vi "PLC_comm.vi"() -> ()   [LabVIEW 2017]
uses:
  <vilib>/addons/database/NI_Database_API.lvlib
  Global/DATA LOG.vi
  Global/Global 1.vi
  <vilib>/DATA AHEAD/SP7/typedefs/PLC Type.ctl
  <vilib>/DATA AHEAD/SP7/SP7.lvlib
  <vilib>/DATA AHEAD/SP7/functions/read/read String.vi
  <vilib>/DATA AHEAD/SP7/functions/write/write Dint array.vi
  <vilib>/DATA AHEAD/SP7/functions/read/read Dint array.vi
  <vilib>/Utility/error.llb/DialogType.ctl
  <vilib>/DATA AHEAD/SP7/functions/read/read real array.vi
  <vilib>/DATA AHEAD/SP7/functions/write/writeString.vi
  84f8396c-11e3-4f6e-927f-d6cb52f8486f.vi
  edb3f7e3-deb4-4efd-b63a-82a20ab466dd.vi
  737c4a97-5810-4f09-bfe1-7e6a970161fd.vi
  98a23aa7-5d76-4ce5-89a1-7ffa2d6e86d6.vi
  065602cd-1ec6-46a4-aff5-3b00a0c776c3.vi
  <vilib>/DATA AHEAD/SP7/typedefs/S7 Connection.ctl
  Control/PLC_Comm_State.ctl
  <vilib>/addons/database/Connection.llb/DB Tools Open Connec (String).vi
  f53d9a16-31ea-4c58-9ec6-4ab155e6634a.vi
  f2e501b8-8033-40fd-b99e-90a89dd29cf5.vi
  a17ecfbb-e8aa-4e6f-9723-a9b27e8c0652.vi
  3deaaee4-0312-4209-8b7c-ccc637c44985.vi
  adc7d8b8-ea76-443b-992e-07ffa118bf03.vi
  cf2a4f70-d875-4391-b4be-4b1ea527ec99.vi
  b767813d-b0bc-4642-82b7-59e8eeaf8486.vi
panel:
  out "error out 4":errorcluster
  out "error out 3":errorcluster
  out "IP1 8":string
  out "PLC 8":bool
  out "IP1 7":string
  out "PLC 7":bool
  out "IP1 6":string
  out "PLC 6":bool
  out "IP1 5":string
  out "PLC 5":bool
  out "PLC 4":bool
  out "PLC 3":bool
  out "PLC 1":bool
  out "IP1 4":string
  out "IP1 3":string
  out "IP1 2":string
  out "IP1":string
  in  "stop":bool
  out "error out":errorcluster
  in  "error in (no error)":errorcluster
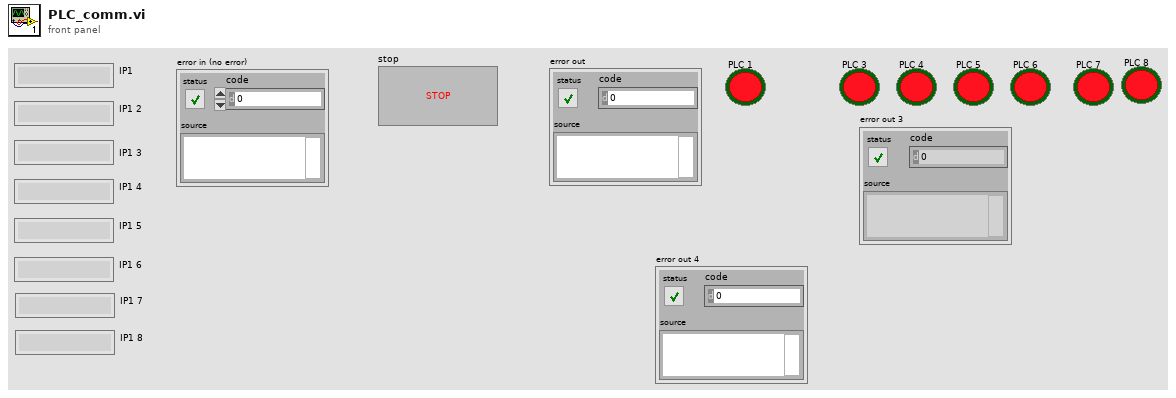
[diagram p1: front panel]
types:
  T1 = typedef "PLC_Comm_State.ctl" = enum16{"Int", "Connect", "Write", "Write2", "Write3", "Read", "Read2", "Read3", "Error", "Disconnect"}
  T2 = typedef "DialogType.ctl" = u16
  T3 = typedef "NI_Database_API.lvlib/Conn ObjectReference.ctl" = refnum<k1>
  T4 = typedef "SP7.lvlib/PLC Type.ctl" = enum16{"S7 200", "S7 300/400", "S7 1200", "S7 1500", "LOGO!8"}
  T5 = typedef "SP7.lvlib/S7 Connection.ctl" = cluster{"TCP Connection Ref":refnum<k5>, "IP address":string, "timeout ms":i32, "Connected?":bool, "PLC Type":T4, "Rack S7 400":u8, "Slot S7 400":u8, "PDU Size":u16, "connection semaphore":T6}
  T6 = typedef "Semaphore RefNum" = refnum<k1>
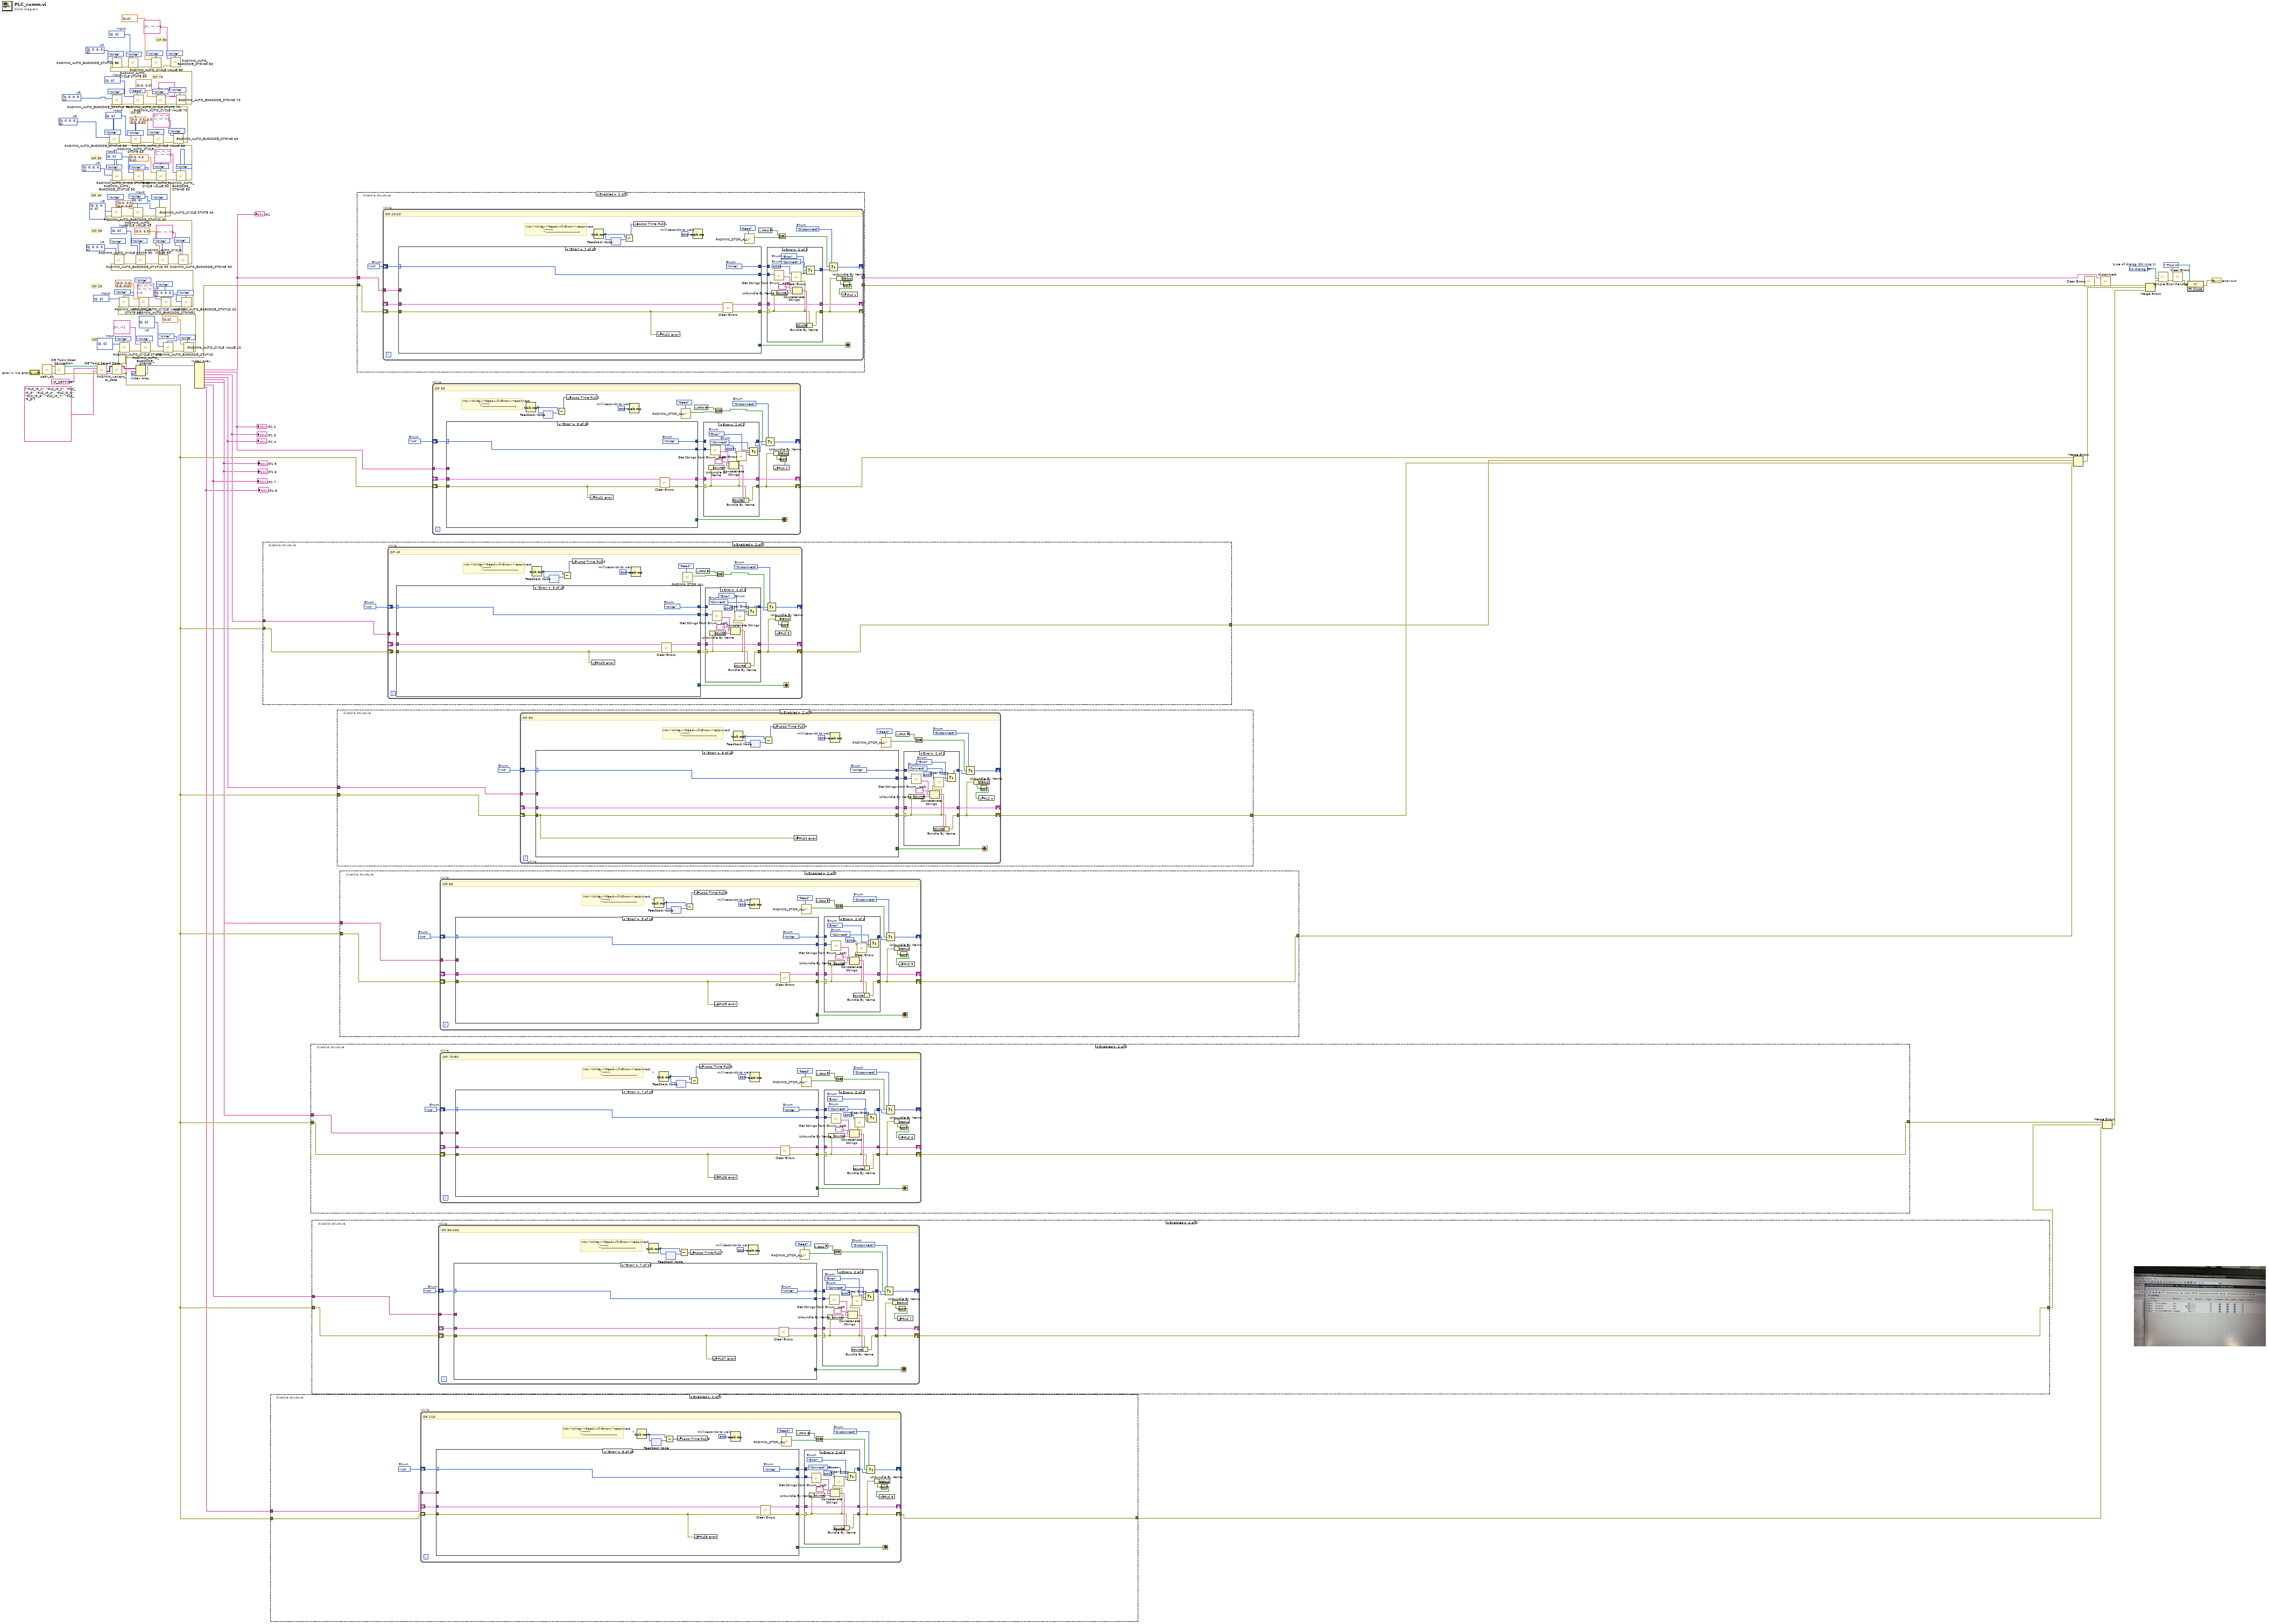
[diagram p0: block diagram]
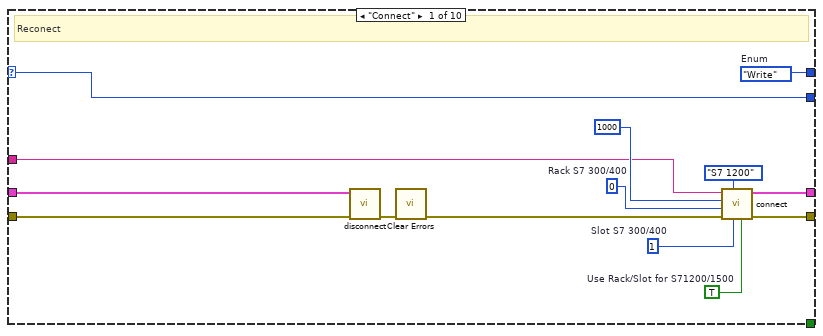
[diagram p3: hidden frame]
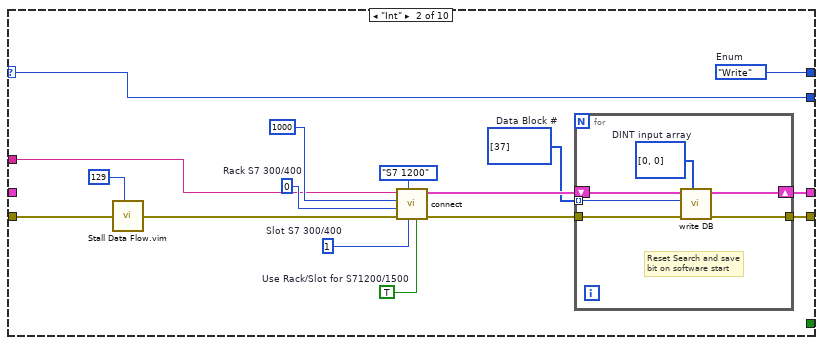
[diagram p4: hidden frame]
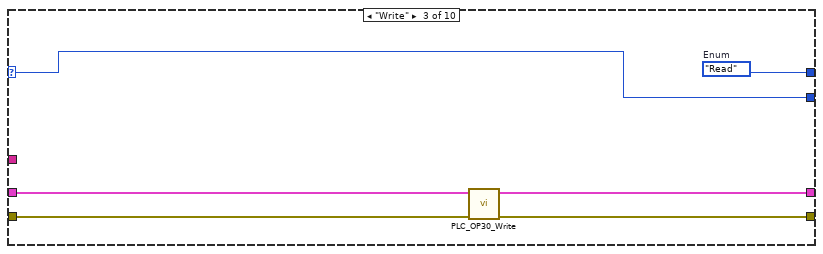
[diagram p5: hidden frame]
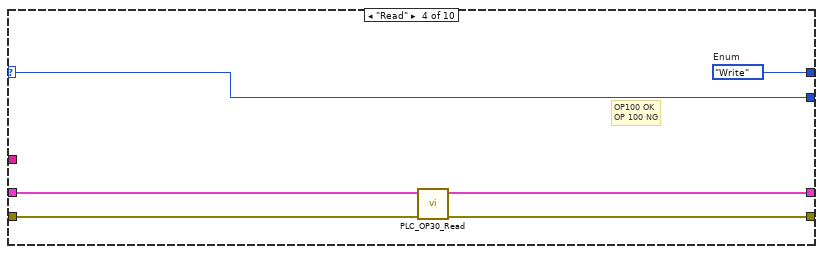
[diagram p6: hidden frame]
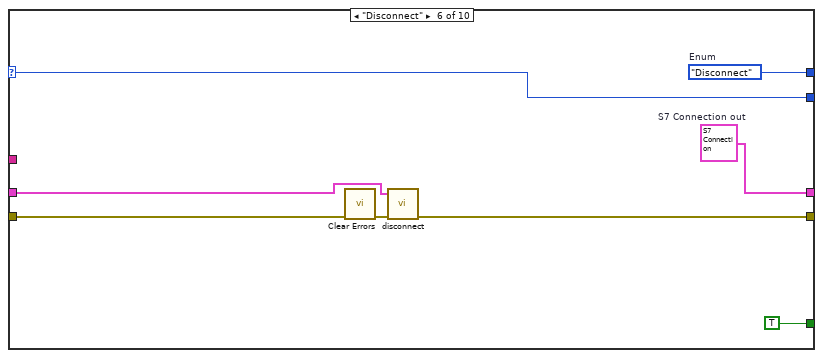
[diagram p7: hidden frame]
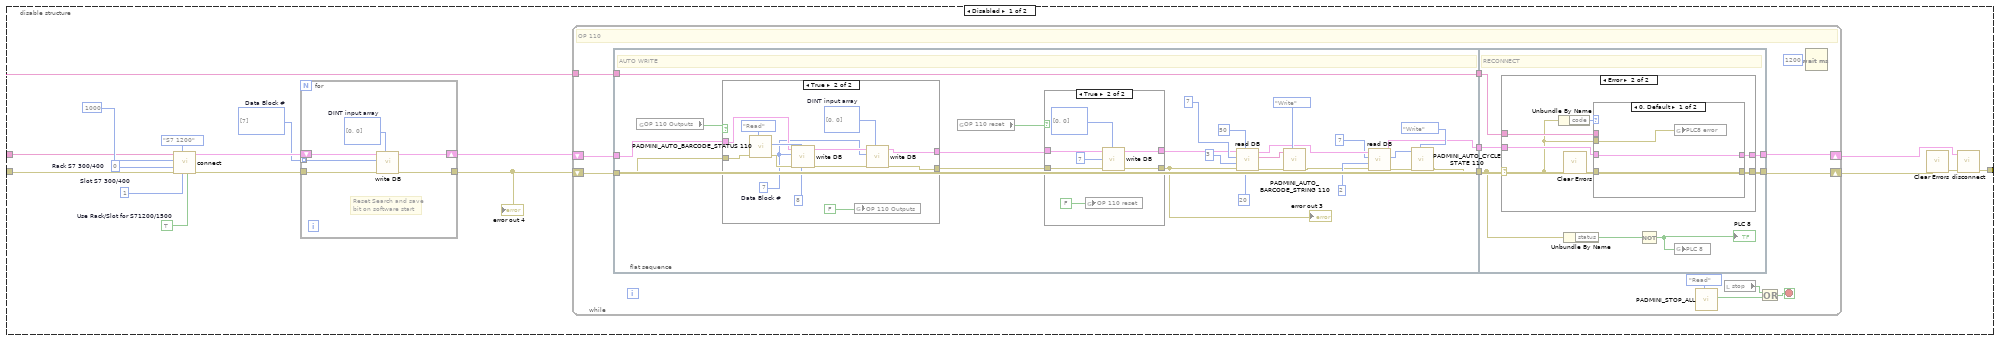
[diagram p12: hidden frame]
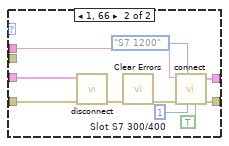
[diagram p16: hidden frame]
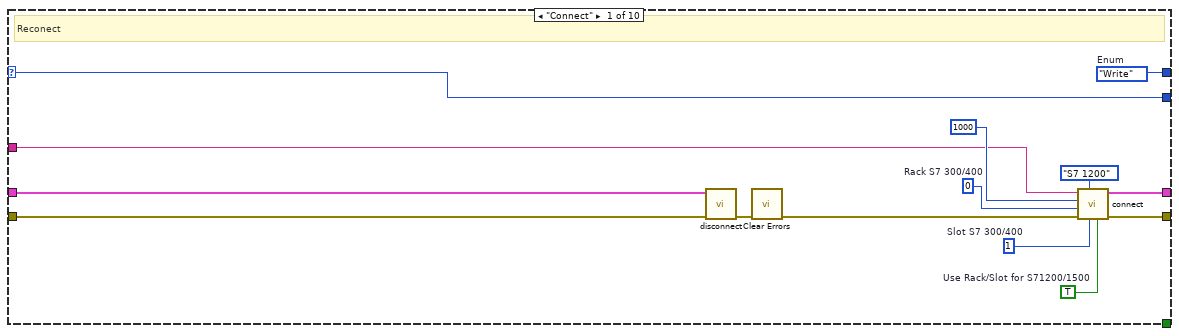
[diagram p18: hidden frame]
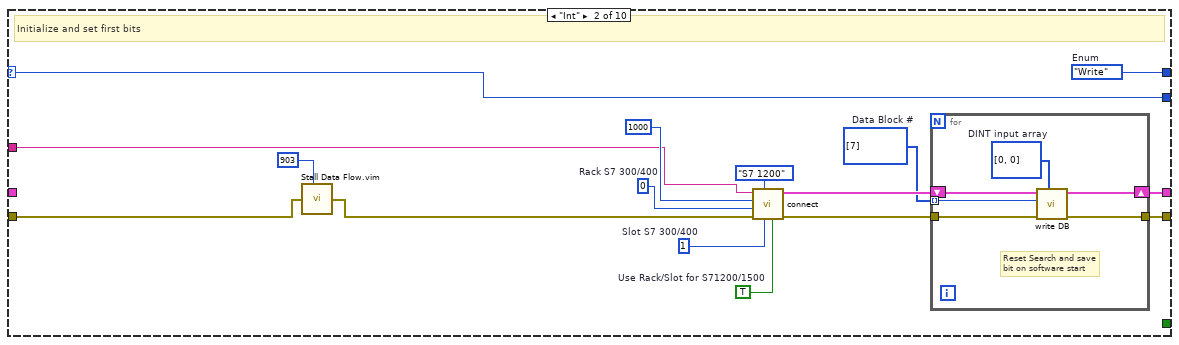
[diagram p19: hidden frame]
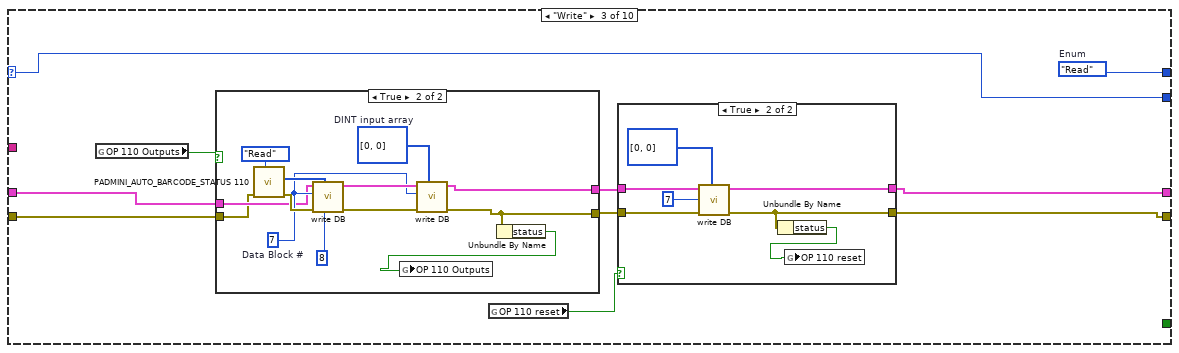
[diagram p20: hidden frame]
diagram:
  w1 = PLC_Comm_State."Int"  # Enum
  w10 = T2 0 items=["no dialog", "OK message", "continue or stop message", "OK message + warnings", "continue/stop + warnings"]  # type of dialog (OK msg:1)
  w12 = i32[] [0, 0, 0, 0, 0]  # I/P
  w13 = i32[] [0, 0]  # Input
  w15 = i32[] [0, 0]  # Input
  w16 = i32[] [0, 0]  # Input
  w18 = i32[] [0, 0]  # Input
  w14 = i32[] [0, 0, 0, 0, 0]  # I/P
  w17 = i32[] [0, 0, 0, 0, 0]  # I/P
  w19 = i32[] [0, 0, 0, 0, 0]  # I/P
  w20 = i32[] [0, 0, 0, 0, 0]  # I/P
  w21 = i32[] [0, 0]  # Input
  w22 = i32[] [0, 0]  # Input
  w23 = i32[] [0, 0, 0, 0, 0]  # I/P
  w24 = i32[] [0, 0, 0, 0, 0]  # I/P
  w25 = i32[] [0, 0]  # Input
  w26 = i32[] [0, 0]  # I/P
  w27 = i32[] [0, 0]  # Input
  # "OP 80"
  # "OP 70"
  # "OP 60"
  # "OP 50"
  # "OP 40"
  # "OP 30"
  # "OP 20"
  # "OP 10"
  n1 = call "path_db.vi"("error in"="error in (no error)") -> ("error out"=w128:errorcluster, "resulting string"=w133:string)  [unwired: 9 in]
  n2 = call-poly <vilib>:"DB Tools Open Connection.vi"("error in (no error)"=w128, "connection information"=w133) -> ("error out"=w132:errorcluster, "connection reference"=w131:T3)  [unwired: 6 in]
  n3 = call <vilib>:"DB Tools Select Data.vi"("error in (no error)"=w132, "columns"=string[] ["PLC_IP_1", "PLC_IP_2", "PLC_IP_3", "PLC_IP_4", "PLC_IP_5", "PLC_IP_6", "PLC_IP_7", "PLC_IP_8"], "table"="IP_SETTING", "connection reference"=w131) -> ("error out"=w130:errorcluster, "data"=w129:variant[][])  [unwired: 2 in, 1 out]
  n4 = call "PADMINI_varient_to_data.vi"("error in (no error)"=w130, "data"=w129) -> ("error out"=w9:errorcluster, "Array"=w124:string[][])  [unwired: 8 in]
  n5 = call "PADMINI_AUTO_CYCLE STATE.vi"("Enum"=enum16{"Read", "Write"}."Write", "error in (no error)"=w9, "Input"=w27) -> ("error out"=w114:errorcluster)  [unwired: 7 in, 1 out]
  n6 = Index Array(array=w124, index (row)=0) -> (element=w123:string[])  [unwired: 1 in]
  n7 = call "PADMINI_AUTO_BARCODE_STRING.vi"("Enum"=enum16{"Read", "Write"}."Write", "error in (no error)"=w114, "Input"=string[] ["", ""]) -> ("error out"=w111:errorcluster)  [unwired: 7 in, 1 out]
  n8 = call "PADMINI_AUTO_BARCODE_STATUS.vi"("Enum"=enum16{"Read", "Write"}."Write", "error in (no error)"=w111, "I/P"=w26) -> ("error out"=w109:errorcluster)  [unwired: 7 in, 1 out]
  n9 = call "PADMINI_AUTO_CYCLE VALUE 10.vi"("Enum"=enum16{"Read", "Write"}."Write", "error in (no error)"=w109, "Input"=dbl[] [0.0]) -> ("error out"=w103:errorcluster)  [unwired: 7 in, 1 out]
  n10 = call "PADMINI_AUTO_CYCLE STATE 20.vi"("Enum"=enum16{"Read", "Write"}."Write", "error in (no error)"=w103, "Input"=w13) -> ("error out"=w101:errorcluster)  [unwired: 7 in, 1 out]
  n11 = call "PADMINI_AUTO_CYCLE VALUE 20.vi"("Enum"=enum16{"Read", "Write"}."Write", "error in (no error)"=w101, "Input"=dbl[] [0.0, 0.0, 0.0, 0.0]) -> ("error out"=w97:errorcluster)  [unwired: 7 in, 1 out]
  n12 = call "PADMINI_AUTO_BARCODE_STRING2.vi"("Enum"=enum16{"Read", "Write"}."Write", "error in (no error)"=w97, "Input"=string[] ["", "", "", "", "", "", ""]) -> ("error out"=w95:errorcluster)  [unwired: 7 in, 1 out]
  n13 = call "PADMINI_AUTO_BARCODE_STATUS 20.vi"("Enum"=enum16{"Read", "Write"}."Write", "error in (no error)"=w95, "I/P"=w12) -> ("error out"=w93:errorcluster)  [unwired: 7 in, 1 out]
  n14 = call "PADMINI_AUTO_BARCODE_STATUS 30.vi"("Enum"=enum16{"Read", "Write"}."Write", "error in (no error)"=w93, "I/P"=w14) -> ("error out"=w90:errorcluster)  [unwired: 7 in, 1 out]
  n15 = call "PADMINI_AUTO_CYCLE STATE 30.vi"("Enum"=enum16{"Read", "Write"}."Write", "error in (no error)"=w90, "Input"=w15) -> ("error out"=w89:errorcluster)  [unwired: 7 in, 1 out]
  n16 = call "PADMINI_AUTO_CYCLE VALUE 30.vi"("Enum"=enum16{"Read", "Write"}."Write", "error in (no error)"=w89, "Input"=dbl[] [0.0, 0.0]) -> ("error out"=w86:errorcluster)  [unwired: 7 in, 1 out]
  n17 = call "PADMINI_AUTO_BARCODE_STRING 30.vi"("Enum"=enum16{"Read", "Write"}."Write", "error in (no error)"=w86, "Input"=string[] ["", "", ""]) -> ("error out"=w76:errorcluster)  [unwired: 7 in, 1 out]
  n18 = call "PADMINI_AUTO_BARCODE_STATUS 40.vi"("Enum"=enum16{"Read", "Write"}."Write", "error in (no error)"=w76, "I/P"=w17) -> ("error out"=w75:errorcluster)  [unwired: 7 in, 1 out]
  n19 = call "PADMINI_AUTO_CYCLE VALUE 40.vi"("Enum"=enum16{"Read", "Write"}."Write", "error in (no error)"=w75, "Input"=dbl[] [0.0, 0.0, 0.0, 0.0]) -> ("error out"=w74:errorcluster)  [unwired: 7 in, 1 out]
  n20 = call "PADMINI_AUTO_CYCLE STATE 40.vi"("Enum"=enum16{"Read", "Write"}."Write", "error in (no error)"=w74, "Input"=w16) -> ("error out"=w73:errorcluster)  [unwired: 7 in, 1 out]
  n21 = call "PADMINI_AUTO_BARCODE_STATUS 50.vi"("Enum"=enum16{"Read", "Write"}."Write", "error in (no error)"=w73, "I/P"=w19) -> ("error out"=w65:errorcluster)  [unwired: 7 in, 1 out]
  n22 = call "PADMINI_AUTO_CYCLE STATE 50.vi"("Enum"=enum16{"Read", "Write"}."Write", "error in (no error)"=w65, "Input"=w18) -> ("error out"=w69:errorcluster)  [unwired: 7 in, 1 out]
  n23 = call "PADMINI_AUTO_CYCLE VALUE 50.vi"("Enum"=enum16{"Read", "Write"}."Write", "error in (no error)"=w69, "Input"=dbl[] [0.0, 0.0, 0.0]) -> ("error out"=w66:errorcluster)  [unwired: 7 in, 1 out]
  n24 = call "PADMINI_AUTO_BARCODE_STRING 50.vi"("Enum"=enum16{"Read", "Write"}."Write", "error in (no error)"=w66, "Input"=string[] ["", "", "", "", "", ""]) -> ("error out"=w51:errorcluster)  [unwired: 7 in, 1 out]
  n25 = call "PADMINI_AUTO_BARCODE_STATUS 60.vi"("Enum"=enum16{"Read", "Write"}."Write", "error in (no error)"=w51, "I/P"=w20) -> ("error out"=w55:errorcluster)  [unwired: 7 in, 1 out]
  n26 = call "PADMINI_AUTO_CYCLE STATE 60.vi"("Enum"=enum16{"Read", "Write"}."Write", "error in (no error)"=w55, "Input"=w21) -> ("error out"=w57:errorcluster)  [unwired: 7 in, 1 out]
  n27 = call "PADMINI_AUTO_CYCLE VALUE 60.vi"("Enum"=enum16{"Read", "Write"}."Write", "error in (no error)"=w57, "Input"=dbl[] [0.0, 0.0, 0.0, 0.0, 0.0]) -> ("error out"=w60:errorcluster)  [unwired: 7 in, 1 out]
  n28 = call "PADMINI_AUTO_BARCODE_STRING 60.vi"("Enum"=enum16{"Read", "Write"}."Write", "error in (no error)"=w60, "Input"=string[] ["", "", "", "", "", ""]) -> ("error out"=w34:errorcluster)  [unwired: 7 in, 1 out]
  n29 = call "PADMINI_AUTO_BARCODE_STATUS 70.vi"("Enum"=enum16{"Read", "Write"}."Write", "error in (no error)"=w34, "I/P"=w23) -> ("error out"=w37:errorcluster)  [unwired: 7 in, 1 out]
  n30 = call "PADMINI_AUTO_CYCLE STATE 70.vi"("Enum"=enum16{"Read", "Write"}."Read", "error in (no error)"=w37, "Input"=w22) -> ("error out"=w49:errorcluster)  [unwired: 7 in, 1 out]
  n31 = call "PADMINI_AUTO_CYCLE VALUE 70.vi"("Enum"=enum16{"Read", "Write"}."Write", "error in (no error)"=w49, "Input"=dbl[] [0.0, 0.0]) -> ("error out"=w46:errorcluster)  [unwired: 7 in, 1 out]
  n32 = call "PADMINI_AUTO_BARCODE_STRING 70.vi"("Enum"=enum16{"Read", "Write"}."Write", "error in (no error)"=w46, "Input"=string[] ["", ""]) -> ("error out"=w31:errorcluster)  [unwired: 7 in, 1 out]
  n33 = call "PADMINI_AUTO_BARCODE_STATUS 80.vi"("Enum"=enum16{"Read", "Write"}."Write", "error in (no error)"=w31, "I/P"=w24) -> ("error out"=w38:errorcluster)  [unwired: 7 in, 1 out]
  n34 = call "PADMINI_AUTO_CYCLE STATE 80.vi"("Enum"=enum16{"Read", "Write"}."Write", "error in (no error)"=w38, "Input"=w25) -> ("error out"=w42:errorcluster)  [unwired: 7 in, 1 out]
  n35 = call "PADMINI_AUTO_CYCLE VALUE 80.vi"("Enum"=enum16{"Read", "Write"}."Write", "error in (no error)"=w42, "Input"=sgl[] [0.0]) -> ("error out"=w45:errorcluster)  [unwired: 7 in, 1 out]
  n36 = call "PADMINI_AUTO_BARCODE_STRING 80.vi"("Enum"=enum16{"Read", "Write"}."Write", "error in (no error)"=w45, "Input"=string[] ["", "", ""]) -> ()  [unwired: 7 in, 2 out]
  n37 = Index Array(array=w123) -> (element #1=w82:string, element #2=w83:string, element #3=w81:string, element #4=w71:string, element #5=w61:string, element #6=w30:string, element #7=w29:string, element #8=w8:string)  [unwired: 8 in]
  "IP1" <- w82
  "IP1 2" <- w83
  "IP1 3" <- w81
  "IP1 4" <- w71
  "IP1 5" <- w61
  "IP1 6" <- w30
  "IP1 7" <- w29
  "IP1 8" <- w8
  n38 = disable-structure shown="Enabled" {
    disable-tunnel: w81 -> [w148 w270]
    disable-tunnel: w9 -> [w139 w269]
    disable-tunnel: [w134 w268] -> w3
    frame Disabled {
      w136 = TRUE  # Use Rack/Slot for S71200/1500
      w137 = u8 0  # Rack S7 300/400
      w138 = u8 1  # Slot S7 300/400
      w144 = i32[] [0, 0]  # DINT input array
      # "Reset Search and save \nbit on software start"
      n39 = call <vilib>:"connect.vi"("Use Rack/Slot for S71200/1500"=w136, "Slot S7 300/400"=w138, "PLC Type"=PLC_Type."S7 1200" ("PLC Type 2"), "error in (no error)"=w139, "Rack S7 300/400"=w137, "timeout [ms]"=1000 ("timeout [ms] 2"), "IP address"=w148) -> ("error out"=w141:errorcluster, "S7 Connection out"=w140:T5)  [unwired: 3 in]
      n40 = call-poly <vilib>:"write DB.vi"("DINT input array"=w144, "error in (no error)"=w141, "Data Block #"=u16 56, "S7 Connection in"=w140) -> ("error out"=w143:errorcluster, "S7 Connection out"=w142:T5)  [unwired: 4 in, 2 out]
      n41 = while {
        shift-right: [w153] -> w146
        shift-left: w142 -> [w163]
        shift-right: [w161] -> w147
        shift-left: w143 -> [w162]
        tunnel: w148 -> [w152]
        stop <- w155 stop-if-true
        # "OP 40"
        n42 = flat-sequence {
          tunnel: [w165] -> w159
          tunnel: [w168] -> w154
          tunnel: w162 -> [w213]
          tunnel: w163 -> [w212]
          tunnel: w152 -> [w200]
          tunnel: [w200] -> w151
          tunnel: [w241] -> w161
          tunnel: [w240] -> w153
          tunnel: w159 -> [w243]
          tunnel: w154 -> [w242]
          tunnel: w151 -> [w239]
          frame #0 {
            w193 = u16 57 ("Data Block #")
            w164 = u16 56 ("Data Block #")
            # "AUTO WRITE"
            n43 = global read "DATA LOG.vi" "OP 40 Outputs"() -> (w211:bool)
            n44 = case shown="True" w211 {
              tunnel: w212 -> [w224 w237]
              tunnel: [w225 w229] -> w198
              tunnel: [w224 w231] -> w199
              tunnel: w213 -> [w225 w234]
              frame False {
              }
              frame True {
                w238 = u16 57  # Data Block #
                n45 = call "PADMINI_AUTO_BARCODE_STATUS 40.vi"("Enum"=enum16{"Read", "Write"}."Read", "error in (no error)"=w234) -> ("error out"=w233:errorcluster, "O/P"=w235:i32[])  [unwired: 8 in]
                n46 = global write "DATA LOG.vi" "OP 40 Outputs"(FALSE) -> ()
                n47 = call-poly <vilib>:"write DB.vi"("DINT input array"=w235, "error in (no error)"=w233, "Data Block #"=w238, "S7 Connection in"=w237) -> ("error out"=w228:errorcluster, "S7 Connection out"=w230:T5)  [unwired: 4 in, 2 out]
                n48 = call-poly <vilib>:"write DB.vi"("DINT input array"=i32[] [0], "error in (no error)"=w228, "Data Block #"=u16 56, "S7 Connection in"=w230) -> ("error out"=w229:errorcluster, "S7 Connection out"=w231:T5)  [unwired: 4 in, 2 out]
              }
            }
            n49 = global read "DATA LOG.vi" "OP 40 reset"() -> (w197:bool)
            n50 = global read "DATA LOG.vi" "Auto Cycle On"() -> (w175:bool)
            n51 = case shown="True" w197 {
              tunnel: w198 -> [w214 w223]
              tunnel: [w214 w222] -> w186
              tunnel: w199 -> [w215 w221]
              tunnel: [w215 w220] -> w187
              frame False {
              }
              frame True {
                n52 = global write "DATA LOG.vi" "OP 40 reset"(FALSE) -> ()
                n53 = call-poly <vilib>:"write DB.vi"("Item offset [byte]"=u16 4 ("Data Block #"), "DINT input array"=i32[] [0], "error in (no error)"=w223, "Data Block #"=u16 56, "S7 Connection in"=w221) -> ("error out"=w222:errorcluster, "S7 Connection out"=w220:T5)  [unwired: 3 in, 2 out]
              }
            }
            n54 = Boolean To (0,1)(Boolean=w175) -> (0, 1=w174:i16)
            n55 = Build Array(w174) -> (w173:i16[])
            n56 = global read "Global 1.vi" "Filtered BARCODE selected"() -> (w196:string[])
            n57 = call-poly <vilib>:"write DB.vi"("Item offset [byte]"=u32 20, "DINT input array"=w173, "error in (no error)"=w186, "Data Block #"=w193, "S7 Connection in"=w187) -> ("error out"=w191:errorcluster, "S7 Connection out"=w190:T5)  [unwired: 3 in, 2 out]
            n58 = call-poly <vilib>:"write DB.vi"("Item offset [byte]"=u32 24, "Input STRINGS"=w196, "error in (no error)"=w191, "String length reserved in DB (default=254)"=u16 15, "Data Block #"=w193, "S7 Connection in"=w190) -> ("error out"=w188:errorcluster, "S7 Connection out"=w189:T5)  [unwired: 2 in, 2 out]
            n59 = call-poly <vilib>:"read DB.vi"("Item offset [byte]"=u32 8, "error in (no error)"=w188, "items #"=u16 4 ("Items # [byte]"), "Data Block #"=w164, "S7 Connection in"=w189) -> ("error out"=w203:errorcluster, "REAL result array"=w201:sgl[], "S7 Connection out"=w209:T5)  [unwired: 4 in]
            n60 = call "PADMINI_AUTO_CYCLE VALUE 40.vi"("Enum"=enum16{"Read", "Write"}."Write", "error in (no error)"=w203, "Input"=w201) -> ("error out"=w202:errorcluster)  [unwired: 7 in, 1 out]
            n61 = call-poly <vilib>:"read DB.vi"("Item offset [byte]"=u32 24, "String length reserved in DB (default=254)"=u16 50, "error in (no error)"=w202, "items #"=u16 1 ("Items # [byte]"), "Data Block #"=w164, "S7 Connection in"=w209) -> ("error out"=w185:errorcluster, "STRING result Array"=w178:string[], "S7 Connection out"=w183:T5)  [unwired: 2 in, 1 out]
            n62 = call-poly <vilib>:"read DB.vi"("Item offset [byte]"=u32 76, "String length reserved in DB (default=254)"=u16 10, "error in (no error)"=w185, "items #"=u16 4 ("Items # [byte]"), "Data Block #"=w164, "S7 Connection in"=w183) -> ("error out"=w184:errorcluster, "STRING result Array"=w177:string[], "S7 Connection out"=w166:T5)  [unwired: 2 in, 1 out]
            n63 = Build Array (concatenate)(w178, w177) -> (w176:string[])
            n64 = call "PADMINI_AUTO_BARCODE_STRING 40.vi"("Enum"=enum16{"Read", "Write"}."Write", "error in (no error)"=w184, "Input"=w176) -> ("error out"=w167:errorcluster)  [unwired: 7 in, 1 out]
            n65 = call-poly <vilib>:"read DB.vi"("error in (no error)"=w167, "items #"=u16 2 ("Items # [byte]"), "Data Block #"=w164, "S7 Connection in"=w166) -> ("error out"=w172:errorcluster, "DINT result array"=w171:i32[], "S7 Connection out"=w165:T5)  [unwired: 5 in]
            n66 = call "PADMINI_AUTO_CYCLE STATE 40.vi"("Enum"=enum16{"Read", "Write"}."Write", "error in (no error)"=w172, "Input"=w171) -> ("error out"=w168:errorcluster)  [unwired: 7 in, 1 out]
          }
          frame #1 {
            # "RECONNECT"
            n67 = case shown="Error" w242 {
              selector: w242 -> [w247 w248]
              tunnel: [w246 w252] -> w240
              tunnel: [w247 w253] -> w241
              tunnel: w243 -> [w246 w251]
              tunnel: w239 -> [_ w250]
              frame No Error {
              }
              frame Error {
                n68 = Unbundle By Name(w248) -> ("code"=w249:i32)
                n69 = call <vilib>:"Clear Errors.vi"("error in (no error)"=w248) -> ("error out"=w254:errorcluster)  [unwired: 5 in, 1 out]
                n70 = case shown="0, Default" w249 {
                  tunnel: w254 -> [w256 w267]
                  tunnel: [w256 w265] -> w253
                  tunnel: [w257 w264] -> w252
                  tunnel: w251 -> [w257 w261]
                  tunnel: w250 -> [_ w260]
                  tunnel: w248 -> [w255 _]
                  frame 0, Default {
                    n71 = global write "Global 1.vi" "PLC3 error"(w255) -> ()
                  }
                  frame 1 {
                    n72 = call <vilib>:"disconnect.vi"("error in (no error)"=w267, "S7 Connection in"=w261) -> ("error out"=w266:errorcluster)  [unwired: 8 in, 1 out]
                    n73 = call <vilib>:"Clear Errors.vi"("error in (no error)"=w266) -> ("error out"=w263:errorcluster)  [unwired: 5 in, 1 out]
                    n74 = call <vilib>:"connect.vi"("Use Rack/Slot for S71200/1500"=TRUE, "Slot S7 300/400"=u8 1, "PLC Type"=PLC_Type."S7 1200" ("PLC Type 2"), "error in (no error)"=w263, "IP address"=w260) -> ("error out"=w265:errorcluster, "S7 Connection out"=w264:T5)  [unwired: 5 in]
                  }
                }
              }
            }
            n75 = Unbundle By Name(w242) -> ("status"=w245:bool)
            n76 = Not(x=w245) -> (.not. x?=w244:bool)
            "PLC 3" <- w244
            n77 = global write "Global 1.vi" "PLC 3"(w244) -> ()
          }
        }
        n78 = call "PADMINI_STOP_ALL.vi"("Enum"=enum16{"Read", "Write"}."Read") -> ("Boolean 2"=w157:bool)  [unwired: 9 in, 1 out]
        n79 = local read "stop"() -> (w156:bool)
        n80 = Or(x=w156, y=w157) -> (x .or. y?=w155:bool)
        n81 = Wait (ms)(milliseconds to wait=u32 1200) -> ()  [unwired: 1 out]
      }
      n82 = call <vilib>:"Clear Errors.vi"("error in (no error)"=w147) -> ("error out"=w135:errorcluster)  [unwired: 5 in, 1 out]
      n83 = call <vilib>:"disconnect.vi"("error in (no error)"=w135, "S7 Connection in"=w146) -> ("error out"=w134:errorcluster)  [unwired: 8 in, 1 out]
    }
    frame Enabled {
      w271 = PLC_Comm_State."Int"  # Enum
      n84 = while {
        shift-right: [w285] -> _
        shift-left: w271 -> [w294]
        shift-right: [w275] -> w268
        shift-left: w269 -> [w293]
        shift-right: [w288] -> _
        shift-left: _ -> [w292]
        tunnel: w270 -> [w291]
        stop <- w286 stop-if-true
        w282 = PLC_Comm_State."Disconnect"  # Enum
        w290 = u32 800  # milliseconds to wait
        # "Int-->Write-->Read---if--Error-->reconnect\n               ^------v                                       v\n                ^------------------------------v"
        # "OP 40"
        n85 = case shown="\"Error\"" w294 {
          selector: w294 -> [w313 w331 w369 w422 w434 w438 _ _ _ _]
          tunnel: [w318 w333 w350 w397 w435 w443 w445 w448 w450 w452] -> w295
          tunnel: [w319 w329 w348 w395 w436 w440 w446 w447 w449 w451] -> w287
          tunnel: w293 -> [w316 w327 w351 w398 w432 w441 w445 w448 w450 w452]
          tunnel: w292 -> [w314 _ w349 w396 w436 w442 w446 w447 w449 w451]
          tunnel: w291 -> [w320 w332 _ _ _ _ _ _ _ _]
          tunnel: [w312 w330 w368 w421 w433 w437 _ _ _ _] -> w289
          tunnel: [_ _ _ _ _ TRUE _ _ _ _] -> w286
          tunnel: [w313 w331 w369 w422 w434 w438 _ _ _ _] -> w283
          frame "Connect" {
            w312 = PLC_Comm_State."Write"  # Enum
            w325 = TRUE  # Use Rack/Slot for S71200/1500
            w324 = u8 1  # Slot S7 300/400
            w322 = u8 0  # Rack S7 300/400
            # "Reconect"
            n86 = call <vilib>:"disconnect.vi"("error in (no error)"=w316, "S7 Connection in"=w314) -> ("error out"=w317:errorcluster)  [unwired: 8 in, 1 out]
            n87 = call <vilib>:"Clear Errors.vi"("error in (no error)"=w317) -> ("error out"=w315:errorcluster)  [unwired: 5 in, 1 out]
            n88 = call <vilib>:"connect.vi"("Use Rack/Slot for S71200/1500"=w325, "Slot S7 300/400"=w324, "PLC Type"=PLC_Type."S7 1200" ("PLC Type 2"), "error in (no error)"=w315, "Rack S7 300/400"=w322, "timeout [ms]"=1000 ("timeout [ms] 2"), "IP address"=w320) -> ("error out"=w318:errorcluster, "S7 Connection out"=w319:T5)  [unwired: 3 in]
          }
          frame "Int" {
            w330 = PLC_Comm_State."Write"  # Enum
            w334 = TRUE  # Use Rack/Slot for S71200/1500
            w335 = u8 1  # Slot S7 300/400
            w336 = u8 0  # Rack S7 300/400
            w337 = u16[] [56]  # Data Block #
            n89 = call "Stall Data Flow.vim"("value in"=w327, "milliseconds to wait"=u32 258) -> ("value out"=w326:errorcluster)  [unwired: 1 out]
            n90 = call <vilib>:"connect.vi"("Use Rack/Slot for S71200/1500"=w334, "Slot S7 300/400"=w335, "PLC Type"=PLC_Type."S7 1200" ("PLC Type 2"), "error in (no error)"=w326, "Rack S7 300/400"=w336, "timeout [ms]"=1000 ("timeout [ms] 2"), "IP address"=w332) -> ("error out"=w339:errorcluster, "S7 Connection out"=w338:T5)  [unwired: 3 in]
            n91 = for {
              tunnel: w337 -> [w347] mode=indexing
              shift-right: [w345] -> w329
              shift-left: w338 -> [w343]
              tunnel: w339 -> [w344]
              tunnel: [w342] -> w333
              w346 = i32[] [0, 0]  # DINT input array
              # "Reset Search and save \nbit on software start"
              n92 = call-poly <vilib>:"write DB.vi"("DINT input array"=w346, "error in (no error)"=w344, "Data Block #"=w347, "S7 Connection in"=w343) -> ("error out"=w342:errorcluster, "S7 Connection out"=w345:T5)  [unwired: 4 in, 2 out]
            }
          }
          frame "Write" {
            w353 = u16 57 ("Data Block #")
            w368 = PLC_Comm_State."Read"  # Enum
            n93 = global read "DATA LOG.vi" "OP 40 Outputs"() -> (w367:bool)
            n94 = case shown="True" w367 {
              tunnel: w349 -> [w380 w382]
              tunnel: [w381 w384] -> w365
              tunnel: [w380 w389] -> w366
              tunnel: w351 -> [w381 w391]
              frame False {
              }
              frame True {
                w394 = u16 57  # Data Block #
                n95 = call "PADMINI_AUTO_BARCODE_STATUS 40.vi"("Enum"=enum16{"Read", "Write"}."Read", "error in (no error)"=w391) -> ("error out"=w390:errorcluster, "O/P"=w392:i32[])  [unwired: 8 in]
                n96 = call-poly <vilib>:"write DB.vi"("DINT input array"=w392, "error in (no error)"=w390, "Data Block #"=w394, "S7 Connection in"=w382) -> ("error out"=w387:errorcluster, "S7 Connection out"=w388:T5)  [unwired: 4 in, 2 out]
                n97 = call-poly <vilib>:"write DB.vi"("DINT input array"=i32[] [0], "error in (no error)"=w387, "Data Block #"=u16 56, "S7 Connection in"=w388) -> ("error out"=w384:errorcluster, "S7 Connection out"=w389:T5)  [unwired: 4 in, 2 out]
                n98 = Unbundle By Name(w384) -> ("status"=w383:bool)
                n99 = global write "DATA LOG.vi" "OP 40 Outputs"(w383) -> ()
              }
            }
            n100 = global read "DATA LOG.vi" "OP 40 reset"() -> (w364:bool)
            n101 = case shown="True" w364 {
              tunnel: w365 -> [w370 w379]
              tunnel: [w370 w374] -> w359
              tunnel: w366 -> [w371 w378]
              tunnel: [w371 w372] -> w360
              frame False {
              }
              frame True {
                n102 = call-poly <vilib>:"write DB.vi"("Item offset [byte]"=u16 4 ("Data Block #"), "DINT input array"=i32[] [0], "error in (no error)"=w379, "Data Block #"=u16 56, "S7 Connection in"=w378) -> ("error out"=w374:errorcluster, "S7 Connection out"=w372:T5)  [unwired: 3 in, 2 out]
                n103 = Unbundle By Name(w374) -> ("status"=w373:bool)
                n104 = global write "DATA LOG.vi" "OP 40 reset"(w373) -> ()
              }
            }
            n105 = global read "DATA LOG.vi" "Auto Cycle On"() -> (w358:bool)
            n106 = global read "Global 1.vi" "Filtered BARCODE selected"() -> (w363:string[])
            n107 = Boolean To (0,1)(Boolean=w358) -> (0, 1=w357:i16)
            n108 = Build Array(w357) -> (w356:i16[])
            n109 = call-poly <vilib>:"write DB.vi"("Item offset [byte]"=u32 20, "DINT input array"=w356, "error in (no error)"=w359, "Data Block #"=w353, "S7 Connection in"=w360) -> ("error out"=w362:errorcluster, "S7 Connection out"=w361:T5)  [unwired: 3 in, 2 out]
            n110 = call-poly <vilib>:"write DB.vi"("Item offset [byte]"=u32 24, "Input STRINGS"=w363, "error in (no error)"=w362, "String length reserved in DB (default=254)"=u16 15, "Data Block #"=w353, "S7 Connection in"=w361) -> ("error out"=w350:errorcluster, "S7 Connection out"=w348:T5)  [unwired: 2 in, 2 out]
          }
          frame "Read" {
            w407 = u16 56 ("Data Block #")
            w421 = PLC_Comm_State."Write"  # Enum
            n111 = call-poly <vilib>:"read DB.vi"("Item offset [byte]"=u32 8, "error in (no error)"=w398, "items #"=u16 4 ("Items # [byte]"), "Data Block #"=w407, "S7 Connection in"=w396) -> ("error out"=w417:errorcluster, "REAL result array"=w420:sgl[], "S7 Connection out"=w418:T5)  [unwired: 4 in]
            n112 = call-poly <vilib>:"read DB.vi"("Item offset [byte]"=u32 24, "String length reserved in DB (default=254)"=u16 50, "error in (no error)"=w417, "items #"=u16 1 ("Items # [byte]"), "Data Block #"=w407, "S7 Connection in"=w418) -> ("error out"=w416:errorcluster, "STRING result Array"=w413:string[], "S7 Connection out"=w414:T5)  [unwired: 2 in, 1 out]
            n113 = call-poly <vilib>:"read DB.vi"("Item offset [byte]"=u32 76, "String length reserved in DB (default=254)"=u16 10, "error in (no error)"=w416, "items #"=u16 4 ("Items # [byte]"), "Data Block #"=w407, "S7 Connection in"=w414) -> ("error out"=w415:errorcluster, "STRING result Array"=w412:string[], "S7 Connection out"=w409:T5)  [unwired: 2 in, 1 out]
            n114 = Build Array (concatenate)(w413, w412) -> (w419:string[])
            n115 = call-poly <vilib>:"read DB.vi"("error in (no error)"=w415, "items #"=u16 2 ("Items # [byte]"), "Data Block #"=w407, "S7 Connection in"=w409) -> ("error out"=w411:errorcluster, "DINT result array"=w410:i32[], "S7 Connection out"=w395:T5)  [unwired: 5 in]
            n116 = case shown="No Error" w411 {
              selector: w411 -> [w426 w431]
              tunnel: w410 -> [w430 _]
              tunnel: w419 -> [w428 _]
              tunnel: w420 -> [w424 _]
              tunnel: [w423 w431] -> w397
              frame No Error {
                w425 = enum16{"Read", "Write"}."Write" ("Enum")
                n117 = call "PADMINI_AUTO_CYCLE VALUE 40.vi"("Enum"=w425, "error in (no error)"=w426, "Input"=w424) -> ("error out"=w427:errorcluster)  [unwired: 7 in, 1 out]
                n118 = call "PADMINI_AUTO_BARCODE_STRING 40.vi"("Enum"=w425, "error in (no error)"=w427, "Input"=w428) -> ("error out"=w429:errorcluster)  [unwired: 7 in, 1 out]
                n119 = call "PADMINI_AUTO_CYCLE STATE 40.vi"("Enum"=w425, "error in (no error)"=w429, "Input"=w430) -> ("error out"=w423:errorcluster)  [unwired: 7 in, 1 out]
              }
              frame Error {
              }
            }
          }
          frame "Error" {
            w433 = PLC_Comm_State."Write"  # Enum
            n120 = global write "Global 1.vi" "PLC3 error"(w432) -> ()
            n121 = call <vilib>:"Clear Errors.vi"("error in (no error)"=w432) -> ("error out"=w435:errorcluster)  [unwired: 5 in, 1 out]
          }
          frame "Disconnect" {
            w437 = PLC_Comm_State."Disconnect"  # Enum
            w440 = T5 {"TCP Connection Ref"=refnum, "IP address"="", "timeout ms"=5000, "Connected?"=FALSE, "PLC Type"=enum."S7 1200", "Rack S7 400"=0, "Slot S7 400"=0, "PDU Size"=0, "connection semaphore"=refnum}  # S7 Connection out
            n122 = call <vilib>:"Clear Errors.vi"("error in (no error)"=w441) -> ("error out"=w444:errorcluster)  [unwired: 5 in, 1 out]
            n123 = call <vilib>:"disconnect.vi"("error in (no error)"=w444, "S7 Connection in"=w442) -> ("error out"=w443:errorcluster)  [unwired: 8 in, 1 out]
          }
          frame "Write2" {
            # "No Use"
          }
          frame "Write3" {
            # "No Use"
          }
          frame "Read2" {
            # "No Use"
          }
          frame "Read3" {
            # "No Use"
          }
        }
        n124 = Tick Count (ms)() -> (millisecond timer value=w274:u32)
        n125 = feedback #1() -> (w273:u32)  [unwired: 1 in]
        n126 = feedback-in #1(w274) -> ()
        n127 = Subtract(x=w274, y=w273) -> (x-y=w272:u32)
        n128 = global write "Global 1.vi" "Loop Time PLC 3"(w272) -> ()
        n129 = Wait (ms)(milliseconds to wait=w290) -> ()  [unwired: 1 out]
        n130 = call "PADMINI_STOP_ALL.vi"("Enum"=enum16{"Read", "Write"}."Read") -> ("Boolean 2"=w281:bool)  [unwired: 9 in, 1 out]
        n131 = local read "stop"() -> (w280:bool)
        n132 = case shown="Error" w295 {
          selector: w295 -> [w298 w301]
          tunnel: [w298 w305] -> w275
          tunnel: [w297 w300] -> w284
          tunnel: w289 -> [w297 _]
          tunnel: [w296 w311] -> w288
          tunnel: w287 -> [w296 w311]
          tunnel: w283 -> [_ w309]
          frame No Error {
          }
          frame Error {
            w302 = PLC_Comm_State."Connect"  # Enum
            w299 = PLC_Comm_State."Error"  # Enum
            n133 = Unbundle By Name(w301) -> ("source"=w310:string)
            n134 = call <userlib>:"Get Strings from Enum__ogtk.vi"("Enum"=w309) -> ("String Value"=w308:string)  [unwired: 7 in, 3 out]
            n135 = Concatenate Strings(w308, "    " ("string"), w310) -> (w306:string)
            n136 = Bundle By Name(cluster=w301, "source"=w306) -> (w305:errorcluster)
            n137 = call <vilib>:"Clear Errors.vi"("error in (no error)"=w301, "specific error code to clear (0: all)"=6002) -> ("specific error cleared?"=w304:bool)  [unwired: 4 in, 1 out]
            n138 = Select(t=w302, s=w304, f=w299) -> (s? t:f=w300:T1)
          }
        }
        n139 = Or(x=w280, y=w281) -> (x .or. y?=w278:bool)
        n140 = Select(t=w282, s=w278, f=w284) -> (s? t:f=w285:T1)
        n141 = Unbundle By Name(w275) -> ("status"=w277:bool)
        n142 = Not(x=w277) -> (.not. x?=w276:bool)
        n143 = global write "Global 1.vi" "PLC 3"(w276) -> ()
      }
    }
  }
  n144 = disable-structure shown="Enabled" {
    disable-tunnel: w9 -> [w462 w567]
    disable-tunnel: w8 -> [w460 w568]
    disable-tunnel: [w456 w566] -> w7
    frame Disabled {
      w453 = TRUE  # Use Rack/Slot for S71200/1500
      w454 = u8 1  # Slot S7 300/400
      w455 = u8 0  # Rack S7 300/400
      w461 = u16[] [7]  # Data Block #
      n145 = call <vilib>:"connect.vi"("Use Rack/Slot for S71200/1500"=w453, "Slot S7 300/400"=w454, "PLC Type"=PLC_Type."S7 1200" ("PLC Type 2"), "error in (no error)"=w462, "Rack S7 300/400"=w455, "timeout [ms]"=1000 ("timeout [ms] 2"), "IP address"=w460) -> ("error out"=w464:errorcluster, "S7 Connection out"=w463:T5)  [unwired: 3 in]
      n146 = for {
        tunnel: w461 -> [w474] mode=indexing
        shift-right: [w472] -> w467
        shift-left: w463 -> [w469]
        tunnel: w464 -> [w470]
        tunnel: [w471] -> w468
        w473 = i32[] [0, 0]  # DINT input array
        # "Reset Search and save \nbit on software start"
        n147 = call-poly <vilib>:"write DB.vi"("DINT input array"=w473, "error in (no error)"=w470, "Data Block #"=w474, "S7 Connection in"=w469) -> ("error out"=w471:errorcluster, "S7 Connection out"=w472:T5)  [unwired: 4 in, 2 out]
      }
      "error out 4" <- w468
      n148 = while {
        shift-right: [w477] -> w457
        shift-left: w467 -> [w487]
        shift-right: [w485] -> w458
        shift-left: w468 -> [w486]
        tunnel: w460 -> [w476]
        stop <- w479 stop-if-true
        # "OP 110"
        n149 = flat-sequence {
          tunnel: [w491] -> w483
          tunnel: [w492] -> w478
          tunnel: w486 -> [w510]
          tunnel: w487 -> [w511]
          tunnel: w476 -> [w512]
          tunnel: [w512] -> w475
          tunnel: [w539] -> w485
          tunnel: [w538] -> w477
          tunnel: w483 -> [w541]
          tunnel: w478 -> [w540]
          tunnel: w475 -> [w537]
          frame #0 {
            # "AUTO WRITE"
            n150 = global read "DATA LOG.vi" "OP 110 Outputs"() -> (w509:bool)
            n151 = case shown="True" w509 {
              tunnel: [w522 w527] -> w501
              tunnel: [w523 w528] -> w500
              tunnel: w510 -> [w522 w532]
              tunnel: w511 -> [w523 w531]
              frame False {
              }
              frame True {
                w524 = i32[] [0, 0]  # DINT input array
                w525 = u16 7  # Data Block #
                n152 = call "PADMINI_AUTO_BARCODE_STATUS 110.vi"("Enum"=enum16{"Read", "Write"}."Read", "error in (no error)"=w532) -> ("error out"=w534:errorcluster, "O/P"=w535:i32[])  [unwired: 8 in]
                n153 = call-poly <vilib>:"write DB.vi"("Item offset [byte]"=u32 8, "DINT input array"=w535, "error in (no error)"=w534, "Data Block #"=w525, "S7 Connection in"=w531) -> ("error out"=w526:errorcluster, "S7 Connection out"=w529:T5)  [unwired: 3 in, 2 out]
                n154 = global write "DATA LOG.vi" "OP 110 Outputs"(FALSE) -> ()
                n155 = call-poly <vilib>:"write DB.vi"("DINT input array"=w524, "error in (no error)"=w526, "Data Block #"=w525, "S7 Connection in"=w529) -> ("error out"=w527:errorcluster, "S7 Connection out"=w528:T5)  [unwired: 4 in, 2 out]
              }
            }
            n156 = global read "DATA LOG.vi" "OP 110 reset"() -> (w498:bool)
            n157 = case shown="True" w498 {
              tunnel: w501 -> [w513 w521]
              tunnel: [w513 w520] -> w502
              tunnel: w500 -> [w514 w519]
              tunnel: [w514 w518] -> w499
              frame False {
              }
              frame True {
                n158 = global write "DATA LOG.vi" "OP 110 reset"(FALSE) -> ()
                n159 = call-poly <vilib>:"write DB.vi"("DINT input array"=i32[] [0, 0], "error in (no error)"=w521, "Data Block #"=u16 7, "S7 Connection in"=w519) -> ("error out"=w520:errorcluster, "S7 Connection out"=w518:T5)  [unwired: 4 in, 2 out]
              }
            }
            "error out 3" <- w502
            n160 = call-poly <vilib>:"read DB.vi"("Item offset [byte]"=u32 20, "String length reserved in DB (default=254)"=u16 50, "error in (no error)"=w502, "items #"=u16 3 ("Items # [byte]"), "Data Block #"=u16 7, "S7 Connection in"=w499) -> ("error out"=w504:errorcluster, "STRING result Array"=w505:string[], "S7 Connection out"=w490:T5)  [unwired: 2 in, 1 out]
            n161 = call "PADMINI_AUTO_BARCODE_STRING 110.vi"("Enum"=enum16{"Read", "Write"}."Write", "error in (no error)"=w504, "Input"=w505) -> ("error out"=w493:errorcluster)  [unwired: 7 in, 1 out]
            n162 = call-poly <vilib>:"read DB.vi"("error in (no error)"=w493, "items #"=u16 2 ("Items # [byte]"), "Data Block #"=u16 7, "S7 Connection in"=w490) -> ("error out"=w497:errorcluster, "DINT result array"=w496:i32[], "S7 Connection out"=w491:T5)  [unwired: 5 in]
            n163 = call "PADMINI_AUTO_CYCLE STATE 110.vi"("Enum"=enum16{"Read", "Write"}."Write", "error in (no error)"=w497, "Input"=w496) -> ("error out"=w492:errorcluster)  [unwired: 7 in, 1 out]
          }
          frame #1 {
            # "RECONNECT"
            n164 = case shown="Error" w540 {
              selector: w540 -> [w545 w546]
              tunnel: [w544 w550] -> w538
              tunnel: [w545 w551] -> w539
              tunnel: w541 -> [w544 w549]
              tunnel: w537 -> [_ w548]
              frame No Error {
              }
              frame Error {
                n165 = Unbundle By Name(w546) -> ("code"=w547:i32)
                n166 = call <vilib>:"Clear Errors.vi"("error in (no error)"=w546) -> ("error out"=w552:errorcluster)  [unwired: 5 in, 1 out]
                n167 = case shown="0, Default" w547 {
                  tunnel: w552 -> [w554 w565]
                  tunnel: [w554 w563] -> w551
                  tunnel: [w555 w562] -> w550
                  tunnel: w549 -> [w555 w559]
                  tunnel: w548 -> [_ w558]
                  tunnel: w546 -> [w553 _]
                  frame 0, Default {
                    n168 = global write "Global 1.vi" "PLC8 error"(w553) -> ()
                  }
                  frame 1, 66 {
                    w557 = u8 1  # Slot S7 300/400
                    n169 = call <vilib>:"disconnect.vi"("error in (no error)"=w565, "S7 Connection in"=w559) -> ("error out"=w564:errorcluster)  [unwired: 8 in, 1 out]
                    n170 = call <vilib>:"Clear Errors.vi"("error in (no error)"=w564) -> ("error out"=w561:errorcluster)  [unwired: 5 in, 1 out]
                    n171 = call <vilib>:"connect.vi"("Use Rack/Slot for S71200/1500"=TRUE, "Slot S7 300/400"=w557, "PLC Type"=PLC_Type."S7 1200" ("PLC Type 2"), "error in (no error)"=w561, "IP address"=w558) -> ("error out"=w563:errorcluster, "S7 Connection out"=w562:T5)  [unwired: 5 in]
                  }
                }
              }
            }
            n172 = Unbundle By Name(w540) -> ("status"=w543:bool)
            n173 = Not(x=w543) -> (.not. x?=w542:bool)
            "PLC 8" <- w542
            n174 = global write "Global 1.vi" "PLC 8"(w542) -> ()
          }
        }
        n175 = call "PADMINI_STOP_ALL.vi"("Enum"=enum16{"Read", "Write"}."Read") -> ("Boolean 2"=w481:bool)  [unwired: 9 in, 1 out]
        n176 = local read "stop"() -> (w480:bool)
        n177 = Or(x=w480, y=w481) -> (x .or. y?=w479:bool)
        n178 = Wait (ms)(milliseconds to wait=u32 1200) -> ()  [unwired: 1 out]
      }
      n179 = call <vilib>:"Clear Errors.vi"("error in (no error)"=w458) -> ("error out"=w459:errorcluster)  [unwired: 5 in, 1 out]
      n180 = call <vilib>:"disconnect.vi"("error in (no error)"=w459, "S7 Connection in"=w457) -> ("error out"=w456:errorcluster)  [unwired: 8 in, 1 out]
    }
    frame Enabled {
      w569 = PLC_Comm_State."Int"  # Enum
      n181 = while {
        shift-right: [w584] -> _
        shift-left: w569 -> [w592]
        shift-right: [w576] -> w566
        shift-left: w567 -> [w591]
        shift-right: [w587] -> _
        shift-left: _ -> [w590]
        tunnel: w568 -> [w573]
        stop <- w585 stop-if-true
        w581 = PLC_Comm_State."Disconnect"  # Enum
        w589 = u32 800  # milliseconds to wait
        # "Int-->Write-->Read---if--Error-->reconnect\n               ^------v                                       v\n                ^------------------------------v"
        # "OP 110"
        n182 = case shown="\"Error\"" w592 {
          selector: w592 -> [w612 w629 w655 w696 w706 w710 _ _ _ _]
          tunnel: [w617 w631 w648 w682 w707 w715 w717 w720 w722 w724] -> w593
          tunnel: [w618 w630 w649 w683 w708 w712 w718 w719 w721 w723] -> w586
          tunnel: w591 -> [w615 w625 w646 w680 w704 w713 w717 w720 w722 w724]
          tunnel: w590 -> [w613 _ w647 w681 w708 w714 w718 w719 w721 w723]
          tunnel: [w611 w628 w654 w695 w705 w709 _ _ _ _] -> w588
          tunnel: [_ _ _ _ _ TRUE _ _ _ _] -> w585
          tunnel: [w612 w629 w655 w696 w706 w710 _ _ _ _] -> w582
          tunnel: w573 -> [w610 w627 _ _ _ _ _ _ _ _]
          frame "Connect" {
            w611 = PLC_Comm_State."Write"  # Enum
            w623 = TRUE  # Use Rack/Slot for S71200/1500
            w622 = u8 1  # Slot S7 300/400
            w620 = u8 0  # Rack S7 300/400
            # "Reconect"
            n183 = call <vilib>:"disconnect.vi"("error in (no error)"=w615, "S7 Connection in"=w613) -> ("error out"=w616:errorcluster)  [unwired: 8 in, 1 out]
            n184 = call <vilib>:"Clear Errors.vi"("error in (no error)"=w616) -> ("error out"=w614:errorcluster)  [unwired: 5 in, 1 out]
            n185 = call <vilib>:"connect.vi"("Use Rack/Slot for S71200/1500"=w623, "Slot S7 300/400"=w622, "PLC Type"=PLC_Type."S7 1200" ("PLC Type 2"), "error in (no error)"=w614, "Rack S7 300/400"=w620, "timeout [ms]"=1000 ("timeout [ms] 2"), "IP address"=w610) -> ("error out"=w617:errorcluster, "S7 Connection out"=w618:T5)  [unwired: 3 in]
          }
          frame "Int" {
            w628 = PLC_Comm_State."Write"  # Enum
            w632 = TRUE  # Use Rack/Slot for S71200/1500
            w633 = u8 1  # Slot S7 300/400
            w634 = u8 0  # Rack S7 300/400
            w635 = u16[] [7]  # Data Block #
            # "Initialize and set first bits"
            n186 = call "Stall Data Flow.vim"("value in"=w625, "milliseconds to wait"=u32 903) -> ("value out"=w624:errorcluster)  [unwired: 1 out]
            n187 = call <vilib>:"connect.vi"("Use Rack/Slot for S71200/1500"=w632, "Slot S7 300/400"=w633, "PLC Type"=PLC_Type."S7 1200" ("PLC Type 2"), "error in (no error)"=w624, "Rack S7 300/400"=w634, "timeout [ms]"=1000 ("timeout [ms] 2"), "IP address"=w627) -> ("error out"=w637:errorcluster, "S7 Connection out"=w636:T5)  [unwired: 3 in]
            n188 = for {
              tunnel: w635 -> [w645] mode=indexing
              shift-right: [w643] -> w630
              shift-left: w636 -> [w641]
              tunnel: w637 -> [w642]
              tunnel: [w640] -> w631
              w644 = i32[] [0, 0]  # DINT input array
              # "Reset Search and save \nbit on software start"
              n189 = call-poly <vilib>:"write DB.vi"("DINT input array"=w644, "error in (no error)"=w642, "Data Block #"=w645, "S7 Connection in"=w641) -> ("error out"=w640:errorcluster, "S7 Connection out"=w643:T5)  [unwired: 4 in, 2 out]
            }
          }
          frame "Write" {
            w654 = PLC_Comm_State."Read"  # Enum
            n190 = global read "DATA LOG.vi" "OP 110 Outputs"() -> (w653:bool)
            n191 = case shown="True" w653 {
              tunnel: [w665 w670] -> w652
              tunnel: [w666 w674] -> w651
              tunnel: w647 -> [w666 w668]
              tunnel: w646 -> [w665 w667]
              frame False {
              }
              frame True {
                w671 = i32[] [0, 0]  # DINT input array
                w672 = u16 7  # Data Block #
                n192 = call "PADMINI_AUTO_BARCODE_STATUS 110.vi"("Enum"=enum16{"Read", "Write"}."Read", "error in (no error)"=w667) -> ("error out"=w677:errorcluster, "O/P"=w678:i32[])  [unwired: 8 in]
                n193 = call-poly <vilib>:"write DB.vi"("Item offset [byte]"=u32 8, "DINT input array"=w678, "error in (no error)"=w677, "Data Block #"=w672, "S7 Connection in"=w668) -> ("error out"=w673:errorcluster, "S7 Connection out"=w675:T5)  [unwired: 3 in, 2 out]
                n194 = call-poly <vilib>:"write DB.vi"("DINT input array"=w671, "error in (no error)"=w673, "Data Block #"=w672, "S7 Connection in"=w675) -> ("error out"=w670:errorcluster, "S7 Connection out"=w674:T5)  [unwired: 4 in, 2 out]
                n195 = Unbundle By Name(w670) -> ("status"=w669:bool)
                n196 = global write "DATA LOG.vi" "OP 110 Outputs"(w669) -> ()
              }
            }
            n197 = global read "DATA LOG.vi" "OP 110 reset"() -> (w650:bool)
            n198 = case shown="True" w650 {
              tunnel: w652 -> [w656 w664]
              tunnel: [w656 w659] -> w648
              tunnel: w651 -> [w657 w663]
              tunnel: [w657 w662] -> w649
              frame False {
              }
              frame True {
                n199 = call-poly <vilib>:"write DB.vi"("DINT input array"=i32[] [0, 0], "error in (no error)"=w664, "Data Block #"=u16 7, "S7 Connection in"=w663) -> ("error out"=w659:errorcluster, "S7 Connection out"=w662:T5)  [unwired: 4 in, 2 out]
                n200 = Unbundle By Name(w659) -> ("status"=w658:bool)
                n201 = global write "DATA LOG.vi" "OP 110 reset"(w658) -> ()
              }
            }
          }
          frame "Read" {
            w695 = PLC_Comm_State."Write"  # Enum
            n202 = call-poly <vilib>:"read DB.vi"("Item offset [byte]"=u32 20, "String length reserved in DB (default=254)"=u16 50, "error in (no error)"=w680, "items #"=u16 3 ("Items # [byte]"), "Data Block #"=u16 7, "S7 Connection in"=w681) -> ("error out"=w693:errorcluster, "STRING result Array"=w694:string[], "S7 Connection out"=w690:T5)  [unwired: 2 in, 1 out]
            n203 = call-poly <vilib>:"read DB.vi"("error in (no error)"=w693, "items #"=u16 2 ("Items # [byte]"), "Data Block #"=u16 7, "S7 Connection in"=w690) -> ("error out"=w692:errorcluster, "DINT result array"=w691:i32[], "S7 Connection out"=w683:T5)  [unwired: 5 in]
            n204 = case shown="Error" w692 {
              selector: w692 -> [w701 w703]
              tunnel: w691 -> [w702 _]
              tunnel: w694 -> [w698 _]
              tunnel: [w697 w703] -> w682
              frame No Error {
                w699 = enum16{"Read", "Write"}."Write" ("Enum")
                n205 = call "PADMINI_AUTO_BARCODE_STRING 110.vi"("Enum"=w699, "error in (no error)"=w701, "Input"=w698) -> ("error out"=w700:errorcluster)  [unwired: 7 in, 1 out]
                n206 = call "PADMINI_AUTO_CYCLE STATE 110.vi"("Enum"=w699, "error in (no error)"=w700, "Input"=w702) -> ("error out"=w697:errorcluster)  [unwired: 7 in, 1 out]
              }
              frame Error {
              }
            }
          }
          frame "Error" {
            w705 = PLC_Comm_State."Write"  # Enum
            n207 = global write "Global 1.vi" "PLC8 error"(w704) -> ()
            n208 = call <vilib>:"Clear Errors.vi"("error in (no error)"=w704) -> ("error out"=w707:errorcluster)  [unwired: 5 in, 1 out]
          }
          frame "Disconnect" {
            w709 = PLC_Comm_State."Disconnect"  # Enum
            w712 = T5 {"TCP Connection Ref"=refnum, "IP address"="", "timeout ms"=5000, "Connected?"=FALSE, "PLC Type"=enum."S7 1200", "Rack S7 400"=0, "Slot S7 400"=0, "PDU Size"=0, "connection semaphore"=refnum}  # S7 Connection out
            n209 = call <vilib>:"Clear Errors.vi"("error in (no error)"=w713) -> ("error out"=w716:errorcluster)  [unwired: 5 in, 1 out]
            n210 = call <vilib>:"disconnect.vi"("error in (no error)"=w716, "S7 Connection in"=w714) -> ("error out"=w715:errorcluster)  [unwired: 8 in, 1 out]
          }
          frame "Write2" {
            # "No Use"
          }
          frame "Write3" {
            # "No Use"
          }
          frame "Read2" {
            # "No Use"
          }
          frame "Read3" {
            # "No Use"
          }
        }
        n211 = Tick Count (ms)() -> (millisecond timer value=w572:u32)
        n212 = feedback #2() -> (w571:u32)  [unwired: 1 in]
        n213 = feedback-in #2(w572) -> ()
        n214 = Subtract(x=w572, y=w571) -> (x-y=w570:u32)
        n215 = global write "Global 1.vi" "Loop Time PLC 8"(w570) -> ()
        n216 = Wait (ms)(milliseconds to wait=w589) -> ()  [unwired: 1 out]
        n217 = call "PADMINI_STOP_ALL.vi"("Enum"=enum16{"Read", "Write"}."Read") -> ("Boolean 2"=w580:bool)  [unwired: 9 in, 1 out]
        n218 = local read "stop"() -> (w575:bool)
        n219 = case shown="Error" w593 {
          selector: w593 -> [w596 w597]
          tunnel: [w596 w603] -> w576
          tunnel: [w595 w599] -> w583
          tunnel: w588 -> [w595 _]
          tunnel: [w594 w609] -> w587
          tunnel: w586 -> [w594 w609]
          tunnel: w582 -> [_ w607]
          frame No Error {
          }
          frame Error {
            w600 = PLC_Comm_State."Connect"  # Enum
            w598 = PLC_Comm_State."Error"  # Enum
            n220 = Unbundle By Name(w597) -> ("source"=w608:string)
            n221 = call <userlib>:"Get Strings from Enum__ogtk.vi"("Enum"=w607) -> ("String Value"=w606:string)  [unwired: 7 in, 3 out]
            n222 = Concatenate Strings(w606, "    " ("string"), w608) -> (w604:string)
            n223 = Bundle By Name(cluster=w597, "source"=w604) -> (w603:errorcluster)
            n224 = call <vilib>:"Clear Errors.vi"("error in (no error)"=w597, "specific error code to clear (0: all)"=6002) -> ("specific error cleared?"=w602:bool)  [unwired: 4 in, 1 out]
            n225 = Select(t=w600, s=w602, f=w598) -> (s? t:f=w599:T1)
          }
        }
        n226 = Or(x=w575, y=w580) -> (x .or. y?=w578:bool)
        n227 = Select(t=w581, s=w578, f=w583) -> (s? t:f=w584:T1)
        n228 = Unbundle By Name(w576) -> ("status"=w577:bool)
        n229 = Not(x=w577) -> (.not. x?=w574:bool)
        n230 = global write "Global 1.vi" "PLC 8"(w574) -> ()
      }
    }
  }
  n231 = disable-structure shown="Enabled" {
    disable-tunnel: w30 -> [w736 w950]
    disable-tunnel: w9 -> [w730 w949]
    disable-tunnel: [w725 w947] -> w5
    frame Disabled {
      w727 = TRUE  # Use Rack/Slot for S71200/1500
      w728 = u8 1  # Slot S7 300/400
      w729 = u8 0  # Rack S7 300/400
      n232 = call <vilib>:"connect.vi"("Use Rack/Slot for S71200/1500"=w727, "Slot S7 300/400"=w728, "PLC Type"=PLC_Type."S7 1200" ("PLC Type 2"), "error in (no error)"=w730, "Rack S7 300/400"=w729, "timeout [ms]"=1000 ("timeout [ms] 2"), "IP address"=w736) -> ("error out"=w731:errorcluster, "S7 Connection out"=w732:T5)  [unwired: 3 in]
      n233 = for {
        tunnel: u16[] [80, 82] ("Data Block #") -> [w746] mode=indexing
        shift-right: [w744] -> w733
        shift-left: w732 -> [w741]
        tunnel: w731 -> [w742]
        tunnel: [w743] -> w734
        w745 = i32[] [0, 0]  # DINT input array
        # "Reset Search and save \nbit on software start"
        n234 = call-poly <vilib>:"write DB.vi"("DINT input array"=w745, "error in (no error)"=w742, "Data Block #"=w746, "S7 Connection in"=w741) -> ("error out"=w743:errorcluster, "S7 Connection out"=w744:T5)  [unwired: 4 in, 2 out]
      }
      n235 = while {
        shift-right: [w749] -> w737
        shift-left: w733 -> [w759]
        shift-right: [w757] -> w738
        shift-left: w734 -> [w758]
        tunnel: w736 -> [w748]
        stop <- w751 stop-if-true
        # "OP 70 - 80"
        n236 = flat-sequence {
          tunnel: [w761] -> w755
          tunnel: [w765] -> w750
          tunnel: w758 -> [w867]
          tunnel: w759 -> [w866]
          tunnel: w748 -> [w854]
          tunnel: [w854] -> w747
          tunnel: [w920] -> w757
          tunnel: [w919] -> w749
          tunnel: w755 -> [w922]
          tunnel: w750 -> [w921]
          tunnel: w747 -> [w918]
          frame #0 {
            w786 = u32 500  # milliseconds to wait
            w813 = u16 83 ("Data Block #")
            w836 = u16 81 ("Data Block #")
            w797 = u16 82 ("Data Block #")
            w773 = u16 80 ("Data Block #")
            # "AUTO WRITE"
            n237 = global read "DATA LOG.vi" "OP 70 Outputs"() -> (w865:bool)
            n238 = case shown="True" w865 {
              tunnel: w866 -> [w903 w916]
              tunnel: [w904 w907] -> w841
              tunnel: [w903 w908] -> w840
              tunnel: w867 -> [w904 w913]
              frame False {
              }
              frame True {
                w917 = u16 81  # Data Block #
                n239 = call "PADMINI_AUTO_BARCODE_STATUS 70.vi"("Enum"=enum16{"Read", "Write"}."Read", "error in (no error)"=w913) -> ("error out"=w912:errorcluster, "O/P"=w914:i32[])  [unwired: 8 in]
                n240 = global write "DATA LOG.vi" "OP 70 Outputs"(FALSE) -> ()
                n241 = call-poly <vilib>:"write DB.vi"("DINT input array"=w914, "error in (no error)"=w912, "Data Block #"=w917, "S7 Connection in"=w916) -> ("error out"=w905:errorcluster, "S7 Connection out"=w906:T5)  [unwired: 4 in, 2 out]
                n242 = call-poly <vilib>:"write DB.vi"("DINT input array"=i32[] [0] ("Data Byte"), "error in (no error)"=w905, "Data Block #"=u16 80, "S7 Connection in"=w906) -> ("error out"=w907:errorcluster, "S7 Connection out"=w908:T5)  [unwired: 4 in, 2 out]
              }
            }
            n243 = global read "DATA LOG.vi" "OP 70 reset"() -> (w842:bool)
            n244 = global read "DATA LOG.vi" "Auto Cycle On"() -> (w790:bool)
            n245 = case shown="True" w842 {
              tunnel: w841 -> [w878 w887]
              tunnel: [w878 w886] -> w831
              tunnel: w840 -> [w879 w885]
              tunnel: [w879 w884] -> w832
              frame False {
              }
              frame True {
                n246 = global write "DATA LOG.vi" "OP 70 reset"(FALSE) -> ()
                n247 = call-poly <vilib>:"write DB.vi"("Item offset [byte]"=u16 4 ("Data Block #"), "DINT input array"=i32[] [0], "error in (no error)"=w887, "Data Block #"=u16 80, "S7 Connection in"=w885) -> ("error out"=w886:errorcluster, "S7 Connection out"=w884:T5)  [unwired: 3 in, 2 out]
              }
            }
            n248 = Boolean To (0,1)(Boolean=w790) -> (0, 1=w789:i16)
            n249 = Build Array(w789) -> (w788:i16[])
            n250 = call "Stall Data Flow.vim"("value in"=w831, "milliseconds to wait"=w786) -> ("value out"=w787:errorcluster)  [unwired: 1 out]
            n251 = global read "Global 1.vi" "Filtered BARCODE selected"() -> (w833:string[])
            n252 = call-poly <vilib>:"write DB.vi"("Item offset [byte]"=u32 20, "DINT input array"=w788, "error in (no error)"=w787, "Data Block #"=w836, "S7 Connection in"=w832) -> ("error out"=w838:errorcluster, "S7 Connection out"=w839:T5)  [unwired: 3 in, 2 out]
            n253 = call-poly <vilib>:"write DB.vi"("Item offset [byte]"=u32 24, "Input STRINGS"=w833, "error in (no error)"=w838, "String length reserved in DB (default=254)"=u16 15, "Data Block #"=w836, "S7 Connection in"=w839) -> ("error out"=w829:errorcluster, "S7 Connection out"=w830:T5)  [unwired: 2 in, 2 out]
            n254 = call "Stall Data Flow.vim"("value in"=w829, "milliseconds to wait"=u32 300) -> ("value out"=w785:errorcluster)  [unwired: 1 out]
            n255 = call-poly <vilib>:"read DB.vi"("Item offset [byte]"=u32 8, "error in (no error)"=w785, "items #"=u16 2 ("Items # [byte]"), "Data Block #"=w773, "S7 Connection in"=w830) -> ("error out"=w857:errorcluster, "REAL result array"=w855:sgl[], "S7 Connection out"=w863:T5)  [unwired: 4 in]
            n256 = call "PADMINI_AUTO_CYCLE VALUE 70.vi"("Enum"=enum16{"Read", "Write"}."Write", "error in (no error)"=w857, "Input"=w855) -> ("error out"=w856:errorcluster)  [unwired: 7 in, 1 out]
            n257 = call "Stall Data Flow.vim"("value in"=w856, "milliseconds to wait"=u32 0) -> ("value out"=w783:errorcluster)  [unwired: 1 out]
            n258 = call-poly <vilib>:"read DB.vi"("Item offset [byte]"=u32 16, "String length reserved in DB (default=254)"=u16 50, "error in (no error)"=w783, "items #"=u16 1 ("Items # [byte]"), "Data Block #"=w773, "S7 Connection in"=w863) -> ("error out"=w822:errorcluster, "STRING result Array"=w821:string[], "S7 Connection out"=w823:T5)  [unwired: 2 in, 1 out]
            n259 = call-poly <vilib>:"read DB.vi"("Item offset [byte]"=u32 68, "String length reserved in DB (default=254)"=u16 10, "error in (no error)"=w822, "items #"=u16 1 ("Items # [byte]"), "Data Block #"=w773, "S7 Connection in"=w823) -> ("error out"=w824:errorcluster, "STRING result Array"=w825:string[], "S7 Connection out"=w772:T5)  [unwired: 2 in, 1 out]
            n260 = Build Array (concatenate)(w821, w825) -> (w819:string[])
            n261 = call "PADMINI_AUTO_BARCODE_STRING 70.vi"("Enum"=enum16{"Read", "Write"}."Write", "error in (no error)"=w824, "Input"=w819) -> ("error out"=w770:errorcluster)  [unwired: 7 in, 1 out]
            n262 = call-poly <vilib>:"read DB.vi"("error in (no error)"=w770, "items #"=u16 2 ("Items # [byte]"), "Data Block #"=w773, "S7 Connection in"=w772) -> ("error out"=w775:errorcluster, "DINT result array"=w777:i32[], "S7 Connection out"=w771:T5)  [unwired: 5 in]
            n263 = call "PADMINI_AUTO_CYCLE STATE 70.vi"("Enum"=enum16{"Read", "Write"}."Write", "error in (no error)"=w775, "Input"=w777) -> ("error out"=w760:errorcluster)  [unwired: 7 in, 1 out]
            n264 = global read "DATA LOG.vi" "OP 80 Outputs"() -> (w843:bool)
            n265 = case shown="True" w843 {
              tunnel: [w889 w892] -> w818
              tunnel: [w888 w893] -> w795
              tunnel: w760 -> [w889 w899]
              tunnel: w771 -> [w888 w896]
              frame False {
              }
              frame True {
                w902 = u16 83  # Data Block #
                n266 = call "PADMINI_AUTO_BARCODE_STATUS 80.vi"("Enum"=enum16{"Read", "Write"}."Read", "error in (no error)"=w899) -> ("error out"=w898:errorcluster, "O/P"=w900:i32[])  [unwired: 8 in]
                n267 = global write "DATA LOG.vi" "OP 80 Outputs"(FALSE) -> ()
                n268 = call-poly <vilib>:"write DB.vi"("DINT input array"=w900, "error in (no error)"=w898, "Data Block #"=w902, "S7 Connection in"=w896) -> ("error out"=w890:errorcluster, "S7 Connection out"=w891:T5)  [unwired: 4 in, 2 out]
                n269 = call-poly <vilib>:"write DB.vi"("DINT input array"=i32[] [0] ("Data Byte"), "error in (no error)"=w890, "Data Block #"=u16 82, "S7 Connection in"=w891) -> ("error out"=w892:errorcluster, "S7 Connection out"=w893:T5)  [unwired: 4 in, 2 out]
              }
            }
            n270 = global read "DATA LOG.vi" "OP 80 reset"() -> (w817:bool)
            n271 = global read "DATA LOG.vi" "Auto Cycle On"() -> (w793:bool)
            n272 = case shown="True" w817 {
              tunnel: w818 -> [w869 w877]
              tunnel: [w869 w872] -> _
              tunnel: [w869 w872] -> w807
              tunnel: w795 -> [w868 w871]
              tunnel: [w868 w870] -> w794
              frame False {
              }
              frame True {
                n273 = global write "DATA LOG.vi" "OP 80 reset"(FALSE) -> ()
                n274 = call-poly <vilib>:"write DB.vi"("Item offset [byte]"=u16 4 ("Data Block #"), "DINT input array"=i32[] [0], "error in (no error)"=w877, "Data Block #"=u16 82, "S7 Connection in"=w871) -> ("error out"=w872:errorcluster, "S7 Connection out"=w870:T5)  [unwired: 3 in, 2 out]
              }
            }
            n275 = Boolean To (0,1)(Boolean=w793) -> (0, 1=w792:i16)
            n276 = Build Array(w792) -> (w791:i16[])
            n277 = global read "Global 1.vi" "Filtered BARCODE selected"() -> (w810:string[])
            n278 = call-poly <vilib>:"write DB.vi"("Item offset [byte]"=u32 20, "DINT input array"=w791, "error in (no error)"=w807, "Data Block #"=w813, "S7 Connection in"=w794) -> ("error out"=w815:errorcluster, "S7 Connection out"=w816:T5)  [unwired: 3 in, 2 out]
            n279 = call-poly <vilib>:"write DB.vi"("Item offset [byte]"=u32 24, "Input STRINGS"=w810, "error in (no error)"=w815, "String length reserved in DB (default=254)"=u16 15, "Data Block #"=w813, "S7 Connection in"=w816) -> ("error out"=w808:errorcluster, "S7 Connection out"=w809:T5)  [unwired: 2 in, 2 out]
            n280 = call-poly <vilib>:"read DB.vi"("Item offset [byte]"=u32 8, "error in (no error)"=w808, "items #"=u16 1 ("Items # [byte]"), "Data Block #"=w797, "S7 Connection in"=w809) -> ("error out"=w851:errorcluster, "REAL result array"=w853:sgl[], "S7 Connection out"=w845:T5)  [unwired: 4 in]
            n281 = call "PADMINI_AUTO_CYCLE VALUE 80.vi"("Enum"=enum16{"Read", "Write"}."Write", "error in (no error)"=w851, "Input"=w853) -> ("error out"=w852:errorcluster)  [unwired: 7 in, 1 out]
            n282 = call "Stall Data Flow.vim"("value in"=w852, "milliseconds to wait"=u32 300) -> ("value out"=w781:errorcluster)  [unwired: 1 out]
            n283 = call-poly <vilib>:"read DB.vi"("Item offset [byte]"=u32 12, "String length reserved in DB (default=254)"=u16 50, "error in (no error)"=w781, "items #"=u16 1 ("Items # [byte]"), "Data Block #"=w797, "S7 Connection in"=w845) -> ("error out"=w802:errorcluster, "STRING result Array"=w800:string[], "S7 Connection out"=w798:T5)  [unwired: 2 in, 1 out]
            n284 = call "Stall Data Flow.vim"("value in"=w802, "milliseconds to wait"=u32 300) -> ("value out"=w779:errorcluster)  [unwired: 1 out]
            n285 = call-poly <vilib>:"read DB.vi"("Item offset [byte]"=u32 64, "String length reserved in DB (default=254)"=u16 10, "error in (no error)"=w779, "items #"=u16 2 ("Items # [byte]"), "Data Block #"=w797, "S7 Connection in"=w798) -> ("error out"=w801:errorcluster, "STRING result Array"=w806:string[], "S7 Connection out"=w762:T5)  [unwired: 2 in, 1 out]
            n286 = Build Array (concatenate)(w800, w806) -> (w799:string[])
            n287 = call "PADMINI_AUTO_BARCODE_STRING 80.vi"("Enum"=enum16{"Read", "Write"}."Write", "error in (no error)"=w801, "Input"=w799) -> ("error out"=w764:errorcluster)  [unwired: 7 in, 1 out]
            n288 = call-poly <vilib>:"read DB.vi"("error in (no error)"=w764, "items #"=u16 2 ("Items # [byte]"), "Data Block #"=u16 82, "S7 Connection in"=w762) -> ("error out"=w768:errorcluster, "DINT result array"=w766:i32[], "S7 Connection out"=w761:T5)  [unwired: 5 in]
            n289 = call "PADMINI_AUTO_CYCLE STATE 80.vi"("Enum"=enum16{"Read", "Write"}."Write", "error in (no error)"=w768, "Input"=w766) -> ("error out"=w765:errorcluster)  [unwired: 7 in, 1 out]
          }
          frame #1 {
            # "RECONNECT"
            n290 = case shown="Error" w921 {
              selector: w921 -> [w926 w927]
              tunnel: [w925 w931] -> w919
              tunnel: [w926 w932] -> w920
              tunnel: w922 -> [w925 w930]
              tunnel: w918 -> [_ w929]
              frame No Error {
              }
              frame Error {
                n291 = Unbundle By Name(w927) -> ("code"=w928:i32)
                n292 = call <vilib>:"Clear Errors.vi"("error in (no error)"=w927) -> ("error out"=w933:errorcluster)  [unwired: 5 in, 1 out]
                n293 = case shown="1, 66" w928 {
                  tunnel: w933 -> [w935 w946]
                  tunnel: [w935 w944] -> w932
                  tunnel: [w936 w943] -> w931
                  tunnel: w930 -> [w936 w940]
                  tunnel: w929 -> [_ w939]
                  tunnel: w927 -> [w934 _]
                  frame 0, Default {
                    n294 = global write "Global 1.vi" "PLC6 error"(w934) -> ()
                  }
                  frame 1, 66 {
                    n295 = call <vilib>:"disconnect.vi"("error in (no error)"=w946, "S7 Connection in"=w940) -> ("error out"=w945:errorcluster)  [unwired: 8 in, 1 out]
                    n296 = call <vilib>:"Clear Errors.vi"("error in (no error)"=w945) -> ("error out"=w942:errorcluster)  [unwired: 5 in, 1 out]
                    n297 = call <vilib>:"connect.vi"("Use Rack/Slot for S71200/1500"=TRUE, "Slot S7 300/400"=u8 1, "PLC Type"=PLC_Type."S7 1200" ("PLC Type 2"), "error in (no error)"=w942, "IP address"=w939) -> ("error out"=w944:errorcluster, "S7 Connection out"=w943:T5)  [unwired: 5 in]
                  }
                }
              }
            }
            n298 = Unbundle By Name(w921) -> ("status"=w924:bool)
            n299 = Not(x=w924) -> (.not. x?=w923:bool)
            "PLC 6" <- w923
            n300 = global write "Global 1.vi" "PLC 6"(w923) -> ()
          }
        }
        n301 = call "PADMINI_STOP_ALL.vi"("Enum"=enum16{"Read", "Write"}."Read") -> ("Boolean 2"=w753:bool)  [unwired: 9 in, 1 out]
        n302 = local read "stop"() -> (w752:bool)
        n303 = Or(x=w752, y=w753) -> (x .or. y?=w751:bool)
        n304 = Wait (ms)(milliseconds to wait=u32 1000) -> ()  [unwired: 1 out]
      }
      n305 = call <vilib>:"Clear Errors.vi"("error in (no error)"=w738) -> ("error out"=w726:errorcluster)  [unwired: 5 in, 1 out]
      n306 = call <vilib>:"disconnect.vi"("error in (no error)"=w726, "S7 Connection in"=w737) -> ("error out"=w725:errorcluster)  [unwired: 8 in, 1 out]
    }
    frame Enabled {
      w948 = PLC_Comm_State."Int"  # Enum
      n307 = while {
        shift-right: [w965] -> _
        shift-left: w948 -> [w973]
        shift-right: [w957] -> w947
        shift-left: w949 -> [w972]
        shift-right: [w968] -> _
        shift-left: _ -> [w971]
        tunnel: w950 -> [w954]
        stop <- w966 stop-if-true
        w962 = PLC_Comm_State."Disconnect"  # Enum
        w970 = u32 800  # milliseconds to wait
        # "Int-->Write-->Read---if--Error-->reconnect\n               ^------v                                       v\n                ^------------------------------v"
        # "OP 70-80"
        n308 = case shown="\"Error\"" w973 {
          selector: w973 -> [w993 w1011 w1048 w1100 w1154 w1191 w1204 w1208 _ _]
          tunnel: [w998 w1013 w1028 w1082 w1128 w1167 w1205 w1213 w1216 w1218] -> w974
          tunnel: [w999 w1012 w1027 w1083 w1127 w1166 w1206 w1210 w1215 w1217] -> w967
          tunnel: w972 -> [w996 w1007 w1029 w1081 w1129 w1164 w1202 w1211 w1216 w1218]
          tunnel: w971 -> [w994 _ w1030 w1080 w1130 w1165 w1206 w1212 w1215 w1217]
          tunnel: [w992 w1010 w1047 w1101 w1153 w1192 w1203 w1207 _ _] -> w969
          tunnel: [_ _ _ _ _ _ _ TRUE _ _] -> w966
          tunnel: [w993 w1011 w1048 w1100 w1154 w1191 w1204 w1208 _ _] -> w963
          tunnel: w954 -> [w991 w1009 _ _ _ _ _ _ _ _]
          frame "Connect" {
            w992 = PLC_Comm_State."Write"  # Enum
            w1004 = TRUE  # Use Rack/Slot for S71200/1500
            w1003 = u8 1  # Slot S7 300/400
            w1001 = u8 0  # Rack S7 300/400
            # "Reconect"
            n309 = call <vilib>:"disconnect.vi"("error in (no error)"=w996, "S7 Connection in"=w994) -> ("error out"=w997:errorcluster)  [unwired: 8 in, 1 out]
            n310 = call <vilib>:"Clear Errors.vi"("error in (no error)"=w997) -> ("error out"=w995:errorcluster)  [unwired: 5 in, 1 out]
            n311 = call <vilib>:"connect.vi"("Use Rack/Slot for S71200/1500"=w1004, "Slot S7 300/400"=w1003, "PLC Type"=PLC_Type."S7 1200" ("PLC Type 2"), "error in (no error)"=w995, "Rack S7 300/400"=w1001, "timeout [ms]"=1000 ("timeout [ms] 2"), "IP address"=w991) -> ("error out"=w998:errorcluster, "S7 Connection out"=w999:T5)  [unwired: 3 in]
          }
          frame "Int" {
            w1010 = PLC_Comm_State."Write"  # Enum
            w1014 = TRUE  # Use Rack/Slot for S71200/1500
            w1015 = u8 1  # Slot S7 300/400
            w1016 = u8 0  # Rack S7 300/400
            # "Initialize and set first bits"
            n312 = call "Stall Data Flow.vim"("value in"=w1007, "milliseconds to wait"=u32 645) -> ("value out"=w1006:errorcluster)  [unwired: 1 out]
            n313 = call <vilib>:"connect.vi"("Use Rack/Slot for S71200/1500"=w1014, "Slot S7 300/400"=w1015, "PLC Type"=PLC_Type."S7 1200" ("PLC Type 2"), "error in (no error)"=w1006, "Rack S7 300/400"=w1016, "timeout [ms]"=1000 ("timeout [ms] 2"), "IP address"=w1009) -> ("error out"=w1018:errorcluster, "S7 Connection out"=w1017:T5)  [unwired: 3 in]
            n314 = for {
              tunnel: u16[] [80, 82] ("Data Block #") -> [w1026] mode=indexing
              shift-right: [w1024] -> w1012
              shift-left: w1017 -> [w1022]
              tunnel: w1018 -> [w1023]
              tunnel: [w1021] -> w1013
              w1025 = i32[] [0, 0]  # DINT input array
              # "Reset Search and save \nbit on software start"
              n315 = call-poly <vilib>:"write DB.vi"("DINT input array"=w1025, "error in (no error)"=w1023, "Data Block #"=w1026, "S7 Connection in"=w1022) -> ("error out"=w1021:errorcluster, "S7 Connection out"=w1024:T5)  [unwired: 4 in, 2 out]
            }
          }
          frame "Write" {
            w1032 = u16 81 ("Data Block #")
            w1047 = PLC_Comm_State."Write2"  # Enum
            # "OP 70 Write"
            n316 = global read "DATA LOG.vi" "OP 70 Outputs"() -> (w1046:bool)
            n317 = case shown="True" w1046 {
              tunnel: w1030 -> [w1062 w1075]
              tunnel: [w1063 w1064] -> w1044
              tunnel: [w1062 w1068] -> w1043
              tunnel: w1029 -> [w1063 w1072]
              frame False {
              }
              frame True {
                w1076 = u16 81  # Data Block #
                n318 = call "PADMINI_AUTO_BARCODE_STATUS 70.vi"("Enum"=enum16{"Read", "Write"}."Read", "error in (no error)"=w1072) -> ("error out"=w1071:errorcluster, "O/P"=w1073:i32[])  [unwired: 8 in]
                n319 = call-poly <vilib>:"write DB.vi"("DINT input array"=w1073, "error in (no error)"=w1071, "Data Block #"=w1076, "S7 Connection in"=w1075) -> ("error out"=w1066:errorcluster, "S7 Connection out"=w1067:T5)  [unwired: 4 in, 2 out]
                n320 = call-poly <vilib>:"write DB.vi"("DINT input array"=i32[] [0] ("Data Byte"), "error in (no error)"=w1066, "Data Block #"=u16 80, "S7 Connection in"=w1067) -> ("error out"=w1065:errorcluster, "S7 Connection out"=w1068:T5)  [unwired: 4 in, 2 out]
                n321 = case shown="No Error" w1065 {
                  selector: w1065 -> [w1077 w1079]
                  tunnel: [w1077 w1079] -> w1064
                  frame No Error {
                    n322 = global write "DATA LOG.vi" "OP 70 Outputs"(FALSE) -> ()
                  }
                  frame Error {
                  }
                }
              }
            }
            n323 = global read "DATA LOG.vi" "OP 70 reset"() -> (w1045:bool)
            n324 = global read "DATA LOG.vi" "Auto Cycle On"() -> (w1037:bool)
            n325 = case shown="True" w1045 {
              tunnel: w1044 -> [w1049 w1058]
              tunnel: [w1049 w1051] -> w1038
              tunnel: w1043 -> [w1050 w1057]
              tunnel: [w1050 w1056] -> w1039
              frame False {
              }
              frame True {
                n326 = call-poly <vilib>:"write DB.vi"("Item offset [byte]"=u16 4 ("Data Block #"), "DINT input array"=i32[] [0], "error in (no error)"=w1058, "Data Block #"=u16 80, "S7 Connection in"=w1057) -> ("error out"=w1052:errorcluster, "S7 Connection out"=w1056:T5)  [unwired: 3 in, 2 out]
                n327 = case shown="No Error" w1052 {
                  selector: w1052 -> [w1059 w1061]
                  tunnel: [w1059 w1061] -> w1051
                  frame No Error {
                    n328 = global write "DATA LOG.vi" "OP 70 reset"(FALSE) -> ()
                  }
                  frame Error {
                  }
                }
              }
            }
            n329 = Boolean To (0,1)(Boolean=w1037) -> (0, 1=w1036:i16)
            n330 = Build Array(w1036) -> (w1035:i16[])
            n331 = global read "Global 1.vi" "Filtered BARCODE selected"() -> (w1040:string[])
            n332 = call-poly <vilib>:"write DB.vi"("Item offset [byte]"=u32 20, "DINT input array"=w1035, "error in (no error)"=w1038, "Data Block #"=w1032, "S7 Connection in"=w1039) -> ("error out"=w1041:errorcluster, "S7 Connection out"=w1042:T5)  [unwired: 3 in, 2 out]
            n333 = call-poly <vilib>:"write DB.vi"("Item offset [byte]"=u32 24, "Input STRINGS"=w1040, "error in (no error)"=w1041, "String length reserved in DB (default=254)"=u16 15, "Data Block #"=w1032, "S7 Connection in"=w1042) -> ("error out"=w1028:errorcluster, "S7 Connection out"=w1027:T5)  [unwired: 2 in, 2 out]
          }
          frame "Write2" {
            w1085 = u16 83 ("Data Block #")
            w1101 = PLC_Comm_State."Read"  # Enum
            # "op 80 wirte 2"
            n334 = global read "DATA LOG.vi" "OP 80 Outputs"() -> (w1099:bool)
            n335 = case shown="True" w1099 {
              tunnel: [w1113 w1115] -> w1098
              tunnel: [w1112 w1118] -> w1092
              tunnel: w1081 -> [w1113 w1123]
              tunnel: w1080 -> [w1112 w1121]
              frame False {
              }
              frame True {
                w1126 = u16 83  # Data Block #
                n336 = call "PADMINI_AUTO_BARCODE_STATUS 80.vi"("Enum"=enum16{"Read", "Write"}."Read", "error in (no error)"=w1123) -> ("error out"=w1122:errorcluster, "O/P"=w1124:i32[])  [unwired: 8 in]
                n337 = call-poly <vilib>:"write DB.vi"("DINT input array"=w1124, "error in (no error)"=w1122, "Data Block #"=w1126, "S7 Connection in"=w1121) -> ("error out"=w1116:errorcluster, "S7 Connection out"=w1117:T5)  [unwired: 4 in, 2 out]
                n338 = call-poly <vilib>:"write DB.vi"("DINT input array"=i32[] [0] ("Data Byte"), "error in (no error)"=w1116, "Data Block #"=u16 82, "S7 Connection in"=w1117) -> ("error out"=w1115:errorcluster, "S7 Connection out"=w1118:T5)  [unwired: 4 in, 2 out]
                n339 = Unbundle By Name(w1115) -> ("status"=w1114:bool)
                n340 = global write "DATA LOG.vi" "OP 80 Outputs"(w1114) -> ()
              }
            }
            n341 = global read "DATA LOG.vi" "OP 80 reset"() -> (w1097:bool)
            n342 = case shown="True" w1097 {
              tunnel: w1098 -> [w1103 w1111]
              tunnel: [w1103 w1105] -> _
              tunnel: [w1103 w1105] -> w1093
              tunnel: w1092 -> [w1102 w1107]
              tunnel: [w1102 w1106] -> w1091
              frame False {
              }
              frame True {
                n343 = call-poly <vilib>:"write DB.vi"("Item offset [byte]"=u16 4 ("Data Block #"), "DINT input array"=i32[] [0], "error in (no error)"=w1111, "Data Block #"=u16 82, "S7 Connection in"=w1107) -> ("error out"=w1105:errorcluster, "S7 Connection out"=w1106:T5)  [unwired: 3 in, 2 out]
                n344 = Unbundle By Name(w1105) -> ("status"=w1104:bool)
                n345 = global write "DATA LOG.vi" "OP 80 reset"(w1104) -> ()
              }
            }
            n346 = global read "DATA LOG.vi" "Auto Cycle On"() -> (w1090:bool)
            n347 = Boolean To (0,1)(Boolean=w1090) -> (0, 1=w1089:i16)
            n348 = Build Array(w1089) -> (w1088:i16[])
            n349 = global read "Global 1.vi" "Filtered BARCODE selected"() -> (w1094:string[])
            n350 = call-poly <vilib>:"write DB.vi"("Item offset [byte]"=u32 20, "DINT input array"=w1088, "error in (no error)"=w1093, "Data Block #"=w1085, "S7 Connection in"=w1091) -> ("error out"=w1095:errorcluster, "S7 Connection out"=w1096:T5)  [unwired: 3 in, 2 out]
            n351 = call-poly <vilib>:"write DB.vi"("Item offset [byte]"=u32 24, "Input STRINGS"=w1094, "error in (no error)"=w1095, "String length reserved in DB (default=254)"=u16 15, "Data Block #"=w1085, "S7 Connection in"=w1096) -> ("error out"=w1082:errorcluster, "S7 Connection out"=w1083:T5)  [unwired: 2 in, 2 out]
          }
          frame "Read" {
            w1139 = u16 80 ("Data Block #")
            w1153 = PLC_Comm_State."Read2"  # Enum
            # "OP70 read"
            n352 = call-poly <vilib>:"read DB.vi"("Item offset [byte]"=u32 8, "error in (no error)"=w1129, "items #"=u16 2 ("Items # [byte]"), "Data Block #"=w1139, "S7 Connection in"=w1130) -> ("error out"=w1149:errorcluster, "REAL result array"=w1152:sgl[], "S7 Connection out"=w1150:T5)  [unwired: 4 in]
            n353 = call-poly <vilib>:"read DB.vi"("Item offset [byte]"=u32 16, "String length reserved in DB (default=254)"=u16 50, "error in (no error)"=w1149, "items #"=u16 1 ("Items # [byte]"), "Data Block #"=w1139, "S7 Connection in"=w1150) -> ("error out"=w1145:errorcluster, "STRING result Array"=w1144:string[], "S7 Connection out"=w1146:T5)  [unwired: 2 in, 1 out]
            n354 = call-poly <vilib>:"read DB.vi"("Item offset [byte]"=u32 68, "String length reserved in DB (default=254)"=u16 10, "error in (no error)"=w1145, "items #"=u16 1 ("Items # [byte]"), "Data Block #"=w1139, "S7 Connection in"=w1146) -> ("error out"=w1147:errorcluster, "STRING result Array"=w1148:string[], "S7 Connection out"=w1141:T5)  [unwired: 2 in, 1 out]
            n355 = Build Array (concatenate)(w1144, w1148) -> (w1151:string[])
            n356 = call-poly <vilib>:"read DB.vi"("error in (no error)"=w1147, "items #"=u16 2 ("Items # [byte]"), "Data Block #"=w1139, "S7 Connection in"=w1141) -> ("error out"=w1142:errorcluster, "DINT result array"=w1143:i32[], "S7 Connection out"=w1127:T5)  [unwired: 5 in]
            n357 = case shown="No Error" w1142 {
              selector: w1142 -> [w1157 w1163]
              tunnel: w1143 -> [w1162 _]
              tunnel: w1151 -> [w1161 _]
              tunnel: w1152 -> [w1158 _]
              tunnel: [w1156 w1163] -> w1128
              frame No Error {
                w1160 = enum16{"Read", "Write"}."Write" ("Enum")
                n358 = call "PADMINI_AUTO_BARCODE_STRING 70.vi"("Enum"=w1160, "error in (no error)"=w1157, "Input"=w1161) -> ("error out"=w1159:errorcluster)  [unwired: 7 in, 1 out]
                n359 = call "PADMINI_AUTO_CYCLE VALUE 70.vi"("Enum"=w1160, "error in (no error)"=w1159, "Input"=w1158) -> ("error out"=w1155:errorcluster)  [unwired: 7 in, 1 out]
                n360 = call "PADMINI_AUTO_CYCLE STATE 70.vi"("Enum"=w1160, "error in (no error)"=w1155, "Input"=w1162) -> ("error out"=w1156:errorcluster)  [unwired: 7 in, 1 out]
              }
              frame Error {
              }
            }
          }
          frame "Read2" {
            w1173 = u16 82 ("Data Block #")
            w1192 = PLC_Comm_State."Write"  # Enum
            # "Op80 Read2"
            n361 = call-poly <vilib>:"read DB.vi"("Item offset [byte]"=u32 8, "error in (no error)"=w1164, "items #"=u16 1 ("Items # [byte]"), "Data Block #"=w1173, "S7 Connection in"=w1165) -> ("error out"=w1179:errorcluster, "REAL result array"=w1190:sgl[], "S7 Connection out"=w1180:T5)  [unwired: 4 in]
            n362 = call-poly <vilib>:"read DB.vi"("Item offset [byte]"=u32 12, "String length reserved in DB (default=254)"=u16 50, "error in (no error)"=w1179, "items #"=u16 1 ("Items # [byte]"), "Data Block #"=w1173, "S7 Connection in"=w1180) -> ("error out"=w1182:errorcluster, "STRING result Array"=w1184:string[], "S7 Connection out"=w1185:T5)  [unwired: 2 in, 1 out]
            n363 = call-poly <vilib>:"read DB.vi"("Item offset [byte]"=u32 64, "String length reserved in DB (default=254)"=u16 10, "error in (no error)"=w1182, "items #"=u16 2 ("Items # [byte]"), "Data Block #"=w1173, "S7 Connection in"=w1185) -> ("error out"=w1183:errorcluster, "STRING result Array"=w1181:string[], "S7 Connection out"=w1188:T5)  [unwired: 2 in, 1 out]
            n364 = Build Array (concatenate)(w1184, w1181) -> (w1189:string[])
            n365 = call-poly <vilib>:"read DB.vi"("error in (no error)"=w1183, "items #"=u16 2 ("Items # [byte]"), "Data Block #"=u16 82, "S7 Connection in"=w1188) -> ("error out"=w1186:errorcluster, "DINT result array"=w1187:i32[], "S7 Connection out"=w1166:T5)  [unwired: 5 in]
            n366 = case shown="No Error" w1186 {
              selector: w1186 -> [w1195 w1201]
              tunnel: w1187 -> [w1200 _]
              tunnel: w1189 -> [w1198 _]
              tunnel: w1190 -> [w1197 _]
              tunnel: [w1193 w1201] -> w1167
              frame No Error {
                w1196 = enum16{"Read", "Write"}."Write" ("Enum")
                n367 = call "PADMINI_AUTO_CYCLE VALUE 80.vi"("Enum"=w1196, "error in (no error)"=w1195, "Input"=w1197) -> ("error out"=w1199:errorcluster)  [unwired: 7 in, 1 out]
                n368 = call "PADMINI_AUTO_BARCODE_STRING 80.vi"("Enum"=w1196, "error in (no error)"=w1199, "Input"=w1198) -> ("error out"=w1194:errorcluster)  [unwired: 7 in, 1 out]
                n369 = call "PADMINI_AUTO_CYCLE STATE 80.vi"("Enum"=w1196, "error in (no error)"=w1194, "Input"=w1200) -> ("error out"=w1193:errorcluster)  [unwired: 7 in, 1 out]
              }
              frame Error {
              }
            }
          }
          frame "Error" {
            w1203 = PLC_Comm_State."Write"  # Enum
            n370 = global write "Global 1.vi" "PLC6 error"(w1202) -> ()
            n371 = call <vilib>:"Clear Errors.vi"("error in (no error)"=w1202) -> ("error out"=w1205:errorcluster)  [unwired: 5 in, 1 out]
          }
          frame "Disconnect" {
            w1207 = PLC_Comm_State."Disconnect"  # Enum
            w1210 = T5 {"TCP Connection Ref"=refnum, "IP address"="", "timeout ms"=5000, "Connected?"=FALSE, "PLC Type"=enum."S7 1200", "Rack S7 400"=0, "Slot S7 400"=0, "PDU Size"=0, "connection semaphore"=refnum}  # S7 Connection out
            n372 = call <vilib>:"Clear Errors.vi"("error in (no error)"=w1211) -> ("error out"=w1214:errorcluster)  [unwired: 5 in, 1 out]
            n373 = call <vilib>:"disconnect.vi"("error in (no error)"=w1214, "S7 Connection in"=w1212) -> ("error out"=w1213:errorcluster)  [unwired: 8 in, 1 out]
          }
          frame "Write3" {
            # "No Use"
          }
          frame "Read3" {
            # "No Use"
          }
        }
        n374 = Tick Count (ms)() -> (millisecond timer value=w953:u32)
        n375 = feedback #3() -> (w952:u32)  [unwired: 1 in]
        n376 = feedback-in #3(w953) -> ()
        n377 = Subtract(x=w953, y=w952) -> (x-y=w951:u32)
        n378 = global write "Global 1.vi" "Loop Time PLC 6"(w951) -> ()
        n379 = Wait (ms)(milliseconds to wait=w970) -> ()  [unwired: 1 out]
        n380 = call "PADMINI_STOP_ALL.vi"("Enum"=enum16{"Read", "Write"}."Read") -> ("Boolean 2"=w961:bool)  [unwired: 9 in, 1 out]
        n381 = local read "stop"() -> (w956:bool)
        n382 = case shown="Error" w974 {
          selector: w974 -> [w977 w978]
          tunnel: [w977 w984] -> w957
          tunnel: [w976 w980] -> w964
          tunnel: w969 -> [w976 _]
          tunnel: [w975 w990] -> w968
          tunnel: w967 -> [w975 w990]
          tunnel: w963 -> [_ w988]
          frame No Error {
          }
          frame Error {
            w981 = PLC_Comm_State."Connect"  # Enum
            w979 = PLC_Comm_State."Error"  # Enum
            n383 = Unbundle By Name(w978) -> ("source"=w989:string)
            n384 = call <userlib>:"Get Strings from Enum__ogtk.vi"("Enum"=w988) -> ("String Value"=w987:string)  [unwired: 7 in, 3 out]
            n385 = Concatenate Strings(w987, "    " ("string"), w989) -> (w985:string)
            n386 = Bundle By Name(cluster=w978, "source"=w985) -> (w984:errorcluster)
            n387 = call <vilib>:"Clear Errors.vi"("error in (no error)"=w978, "specific error code to clear (0: all)"=6002) -> ("specific error cleared?"=w983:bool)  [unwired: 4 in, 1 out]
            n388 = Select(t=w981, s=w983, f=w979) -> (s? t:f=w980:T1)
          }
        }
        n389 = Or(x=w956, y=w961) -> (x .or. y?=w959:bool)
        n390 = Select(t=w962, s=w959, f=w964) -> (s? t:f=w965:T1)
        n391 = Unbundle By Name(w957) -> ("status"=w958:bool)
        n392 = Not(x=w958) -> (.not. x?=w955:bool)
        n393 = global write "Global 1.vi" "PLC 6"(w955) -> ()
      }
    }
  }
  n394 = disable-structure shown="Enabled" {
    disable-tunnel: w29 -> [w1231 w1431]
    disable-tunnel: [w1230 w1429] -> w2
    disable-tunnel: w9 -> [w1224 w1430]
    frame Disabled {
      w1221 = TRUE  # Use Rack/Slot for S71200/1500
      w1222 = u8 1  # Slot S7 300/400
      w1223 = u8 0  # Rack S7 300/400
      n395 = call <vilib>:"connect.vi"("Use Rack/Slot for S71200/1500"=w1221, "Slot S7 300/400"=w1222, "PLC Type"=PLC_Type."S7 1200" ("PLC Type 2"), "error in (no error)"=w1224, "Rack S7 300/400"=w1223, "timeout [ms]"=1000 ("timeout [ms] 2"), "IP address"=w1231) -> ("error out"=w1226:errorcluster, "S7 Connection out"=w1225:T5)  [unwired: 3 in]
      n396 = for {
        tunnel: u16[] [69, 71] ("Data Block #") -> [w1239] mode=indexing
        shift-right: [w1237] -> w1228
        shift-left: w1225 -> [w1234]
        tunnel: w1226 -> [w1235]
        tunnel: [w1236] -> w1227
        w1238 = i32[] [0, 0]  # DINT input array
        # "Reset Search and save \nbit on software start"
        n397 = call-poly <vilib>:"write DB.vi"("DINT input array"=w1238, "error in (no error)"=w1235, "Data Block #"=w1239, "S7 Connection in"=w1234) -> ("error out"=w1236:errorcluster, "S7 Connection out"=w1237:T5)  [unwired: 4 in, 2 out]
      }
      n398 = while {
        shift-right: [w1242] -> w1219
        shift-left: w1228 -> [w1252]
        shift-right: [w1250] -> w1230
        shift-left: w1227 -> [w1251]
        tunnel: w1231 -> [w1241]
        stop <- w1244 stop-if-true
        # "OP 90 - 100"
        n399 = flat-sequence {
          tunnel: [w1254] -> w1248
          tunnel: [w1324] -> w1243
          tunnel: w1251 -> [w1349]
          tunnel: w1252 -> [w1348]
          tunnel: w1241 -> [w1336]
          tunnel: [w1336] -> w1240
          tunnel: [w1402] -> w1250
          tunnel: [w1401] -> w1242
          tunnel: w1248 -> [w1404]
          tunnel: w1243 -> [w1403]
          tunnel: w1240 -> [w1400]
          frame #0 {
            w1293 = u16 72 ("Data Block #")
            w1317 = u16 70 ("Data Block #")
            w1253 = u16 71 ("Data Block #")
            w1261 = u16 69 ("Data Block #")
            # "AUTO WRITE"
            n400 = global read "DATA LOG.vi" "OP 90 Outputs"() -> (w1347:bool)
            n401 = case shown="True" w1347 {
              tunnel: w1348 -> [w1385 w1398]
              tunnel: [w1386 w1387] -> w1322
              tunnel: [w1385 w1388] -> w1323
              tunnel: w1349 -> [w1386 w1395]
              frame False {
              }
              frame True {
                w1399 = u16 70  # Data Block #
                n402 = call "PADMINI_AUTO_BARCODE_STATUS 90.vi"("Enum"=enum16{"Read", "Write"}."Read", "error in (no error)"=w1395) -> ("error out"=w1394:errorcluster, "O/P"=w1396:i32[])  [unwired: 8 in]
                n403 = global write "DATA LOG.vi" "OP 90 Outputs"(FALSE) -> ()
                n404 = call-poly <vilib>:"write DB.vi"("DINT input array"=w1396, "error in (no error)"=w1394, "Data Block #"=w1399, "S7 Connection in"=w1398) -> ("error out"=w1390:errorcluster, "S7 Connection out"=w1389:T5)  [unwired: 4 in, 2 out]
                n405 = call-poly <vilib>:"write DB.vi"("DINT input array"=i32[] [0] ("Data Byte"), "error in (no error)"=w1390, "Data Block #"=u16 69, "S7 Connection in"=w1389) -> ("error out"=w1387:errorcluster, "S7 Connection out"=w1388:T5)  [unwired: 4 in, 2 out]
              }
            }
            n406 = global read "DATA LOG.vi" "OP 90 reset"() -> (w1321:bool)
            n407 = case shown="True" w1321 {
              tunnel: w1322 -> [w1360 w1369]
              tunnel: [w1360 w1368] -> w1310
              tunnel: w1323 -> [w1361 w1367]
              tunnel: [w1361 w1366] -> w1311
              frame False {
              }
              frame True {
                n408 = global write "DATA LOG.vi" "OP 90 reset"(FALSE) -> ()
                n409 = call-poly <vilib>:"write DB.vi"("Item offset [byte]"=u16 4 ("Data Block #"), "DINT input array"=i32[] [0], "error in (no error)"=w1369, "Data Block #"=u16 69, "S7 Connection in"=w1367) -> ("error out"=w1368:errorcluster, "S7 Connection out"=w1366:T5)  [unwired: 3 in, 2 out]
              }
            }
            n410 = global read "DATA LOG.vi" "Auto Cycle On"() -> (w1276:bool)
            n411 = Boolean To (0,1)(Boolean=w1276) -> (0, 1=w1275:i16)
            n412 = Build Array(w1275) -> (w1274:i16[])
            n413 = global read "Global 1.vi" "Filtered BARCODE selected"() -> (w1320:string[])
            n414 = call-poly <vilib>:"write DB.vi"("Item offset [byte]"=u32 20, "DINT input array"=w1274, "error in (no error)"=w1310, "Data Block #"=w1317, "S7 Connection in"=w1311) -> ("error out"=w1315:errorcluster, "S7 Connection out"=w1314:T5)  [unwired: 3 in, 2 out]
            n415 = call-poly <vilib>:"write DB.vi"("Item offset [byte]"=u32 24, "Input STRINGS"=w1320, "error in (no error)"=w1315, "String length reserved in DB (default=254)"=u16 15, "Data Block #"=w1317, "S7 Connection in"=w1314) -> ("error out"=w1312:errorcluster, "S7 Connection out"=w1313:T5)  [unwired: 2 in, 2 out]
            n416 = call-poly <vilib>:"read DB.vi"("Item offset [byte]"=u32 8, "error in (no error)"=w1312, "items #"=u16 2 ("Items # [byte]"), "Data Block #"=w1261, "S7 Connection in"=w1313) -> ("error out"=w1339:errorcluster, "REAL result array"=w1337:sgl[], "S7 Connection out"=w1345:T5)  [unwired: 4 in]
            n417 = call "PADMINI_AUTO_CYCLE VALUE 90.vi"("Enum"=enum16{"Read", "Write"}."Write", "error in (no error)"=w1339, "Input"=w1337) -> ("error out"=w1338:errorcluster)  [unwired: 7 in, 1 out]
            n418 = call-poly <vilib>:"read DB.vi"("Item offset [byte]"=u32 16, "String length reserved in DB (default=254)"=u16 50, "error in (no error)"=w1338, "items #"=u16 1 ("Items # [byte]"), "Data Block #"=w1261, "S7 Connection in"=w1345) -> ("error out"=w1309:errorcluster, "STRING result Array"=w1302:string[], "S7 Connection out"=w1308:T5)  [unwired: 2 in, 1 out]
            n419 = call-poly <vilib>:"read DB.vi"("Item offset [byte]"=u32 68, "String length reserved in DB (default=254)"=u16 10, "error in (no error)"=w1309, "items #"=u16 3 ("Items # [byte]"), "Data Block #"=w1261, "S7 Connection in"=w1308) -> ("error out"=w1307:errorcluster, "STRING result Array"=w1301:string[], "S7 Connection out"=w1264:T5)  [unwired: 2 in, 1 out]
            n420 = Build Array (concatenate)(w1302, w1301) -> (w1300:string[])
            n421 = call "PADMINI_AUTO_BARCODE_STRING 90.vi"("Enum"=enum16{"Read", "Write"}."Write", "error in (no error)"=w1307, "Input"=w1300) -> ("error out"=w1263:errorcluster)  [unwired: 7 in, 1 out]
            n422 = call-poly <vilib>:"read DB.vi"("error in (no error)"=w1263, "items #"=u16 2 ("Items # [byte]"), "Data Block #"=w1261, "S7 Connection in"=w1264) -> ("error out"=w1267:errorcluster, "DINT result array"=w1269:i32[], "S7 Connection out"=w1265:T5)  [unwired: 5 in]
            n423 = call "PADMINI_AUTO_CYCLE STATE 90.vi"("Enum"=enum16{"Read", "Write"}."Write", "error in (no error)"=w1267, "Input"=w1269) -> ("error out"=w1262:errorcluster)  [unwired: 7 in, 1 out]
            n424 = global read "DATA LOG.vi" "OP 100 Outputs"() -> (w1325:bool)
            n425 = case shown="True" w1325 {
              tunnel: w1265 -> [w1370 w1383]
              tunnel: [w1371 w1374] -> w1298
              tunnel: [w1370 w1375] -> w1299
              tunnel: w1262 -> [w1371 w1380]
              frame False {
              }
              frame True {
                w1384 = u16 72  # Data Block #
                n426 = call "PADMINI_AUTO_BARCODE_STATUS 100.vi"("Enum"=enum16{"Read", "Write"}."Read", "error in (no error)"=w1380) -> ("error out"=w1379:errorcluster, "O/P"=w1381:i32[])  [unwired: 8 in]
                n427 = global write "DATA LOG.vi" "OP 100 Outputs"(FALSE) -> ()
                n428 = call-poly <vilib>:"write DB.vi"("DINT input array"=w1381, "error in (no error)"=w1379, "Data Block #"=w1384, "S7 Connection in"=w1383) -> ("error out"=w1373:errorcluster, "S7 Connection out"=w1372:T5)  [unwired: 4 in, 2 out]
                n429 = call-poly <vilib>:"write DB.vi"("DINT input array"=i32[] [0] ("Data Byte"), "error in (no error)"=w1373, "Data Block #"=u16 71, "S7 Connection in"=w1372) -> ("error out"=w1374:errorcluster, "S7 Connection out"=w1375:T5)  [unwired: 4 in, 2 out]
              }
            }
            n430 = global read "DATA LOG.vi" "OP 100 reset"() -> (w1297:bool)
            n431 = case shown="True" w1297 {
              tunnel: w1298 -> [w1350 w1359]
              tunnel: [w1350 w1358] -> w1289
              tunnel: w1299 -> [w1351 w1357]
              tunnel: [w1351 w1356] -> w1288
              frame False {
              }
              frame True {
                n432 = global write "DATA LOG.vi" "OP 100 reset"(FALSE) -> ()
                n433 = call-poly <vilib>:"write DB.vi"("Item offset [byte]"=u16 4 ("Data Block #"), "DINT input array"=i32[] [0], "error in (no error)"=w1359, "Data Block #"=u16 71, "S7 Connection in"=w1357) -> ("error out"=w1358:errorcluster, "S7 Connection out"=w1356:T5)  [unwired: 3 in, 2 out]
              }
            }
            n434 = global read "DATA LOG.vi" "Auto Cycle On"() -> (w1273:bool)
            n435 = Boolean To (0,1)(Boolean=w1273) -> (0, 1=w1272:i16)
            n436 = Build Array(w1272) -> (w1271:i16[])
            n437 = global read "Global 1.vi" "Filtered BARCODE selected"() -> (w1290:string[])
            n438 = call-poly <vilib>:"write DB.vi"("Item offset [byte]"=u32 20, "DINT input array"=w1271, "error in (no error)"=w1289, "Data Block #"=w1293, "S7 Connection in"=w1288) -> ("error out"=w1295:errorcluster, "S7 Connection out"=w1296:T5)  [unwired: 3 in, 2 out]
            n439 = call-poly <vilib>:"write DB.vi"("Item offset [byte]"=u32 24, "Input STRINGS"=w1290, "error in (no error)"=w1295, "String length reserved in DB (default=254)"=u16 15, "Data Block #"=w1293, "S7 Connection in"=w1296) -> ("error out"=w1286:errorcluster, "S7 Connection out"=w1287:T5)  [unwired: 2 in, 2 out]
            n440 = call-poly <vilib>:"read DB.vi"("Item offset [byte]"=u32 8, "error in (no error)"=w1286, "items #"=u16 11 ("Items # [byte]"), "Data Block #"=w1253, "S7 Connection in"=w1287) -> ("error out"=w1333:errorcluster, "REAL result array"=w1335:sgl[], "S7 Connection out"=w1327:T5)  [unwired: 4 in]
            n441 = call "PADMINI_AUTO_CYCLE VALUE 100.vi"("Enum"=enum16{"Read", "Write"}."Write", "error in (no error)"=w1333, "Input"=w1335) -> ("error out"=w1334:errorcluster)  [unwired: 7 in, 1 out]
            n442 = call-poly <vilib>:"read DB.vi"("Item offset [byte]"=u32 52, "String length reserved in DB (default=254)"=u16 50, "error in (no error)"=w1334, "items #"=u16 1 ("Items # [byte]"), "Data Block #"=w1253, "S7 Connection in"=w1327) -> ("error out"=w1283:errorcluster, "STRING result Array"=w1281:string[], "S7 Connection out"=w1282:T5)  [unwired: 2 in, 1 out]
            n443 = call-poly <vilib>:"read DB.vi"("Item offset [byte]"=u32 104, "String length reserved in DB (default=254)"=u16 10, "error in (no error)"=w1283, "items #"=u16 2 ("Items # [byte]"), "Data Block #"=w1253, "S7 Connection in"=w1282) -> ("error out"=w1284:errorcluster, "STRING result Array"=w1279:string[], "S7 Connection out"=w1255:T5)  [unwired: 2 in, 1 out]
            n444 = Build Array (concatenate)(w1281, w1279) -> (w1280:string[])
            n445 = call "PADMINI_AUTO_BARCODE_STRING 100.vi"("Enum"=enum16{"Read", "Write"}."Write", "error in (no error)"=w1284, "Input"=w1280) -> ("error out"=w1256:errorcluster)  [unwired: 7 in, 1 out]
            n446 = call-poly <vilib>:"read DB.vi"("error in (no error)"=w1256, "items #"=u16 2 ("Items # [byte]"), "Data Block #"=w1253, "S7 Connection in"=w1255) -> ("error out"=w1259:errorcluster, "DINT result array"=w1260:i32[], "S7 Connection out"=w1254:T5)  [unwired: 5 in]
            n447 = call "PADMINI_AUTO_CYCLE STATE 100.vi"("Enum"=enum16{"Read", "Write"}."Write", "error in (no error)"=w1259, "Input"=w1260) -> ("error out"=w1324:errorcluster)  [unwired: 7 in, 1 out]
          }
          frame #1 {
            # "RECONNECT"
            n448 = case shown="Error" w1403 {
              selector: w1403 -> [w1408 w1409]
              tunnel: [w1407 w1413] -> w1401
              tunnel: [w1408 w1414] -> w1402
              tunnel: w1404 -> [w1407 w1412]
              tunnel: w1400 -> [_ w1411]
              frame No Error {
              }
              frame Error {
                n449 = Unbundle By Name(w1409) -> ("code"=w1410:i32)
                n450 = call <vilib>:"Clear Errors.vi"("error in (no error)"=w1409) -> ("error out"=w1415:errorcluster)  [unwired: 5 in, 1 out]
                n451 = case shown="1, 66" w1410 {
                  tunnel: w1415 -> [w1417 w1428]
                  tunnel: [w1417 w1426] -> w1414
                  tunnel: [w1418 w1425] -> w1413
                  tunnel: w1412 -> [w1418 w1422]
                  tunnel: w1411 -> [_ w1421]
                  tunnel: w1409 -> [w1416 _]
                  frame 0, Default {
                    n452 = global write "Global 1.vi" "PLC7 error"(w1416) -> ()
                  }
                  frame 1, 66 {
                    n453 = call <vilib>:"disconnect.vi"("error in (no error)"=w1428, "S7 Connection in"=w1422) -> ("error out"=w1427:errorcluster)  [unwired: 8 in, 1 out]
                    n454 = call <vilib>:"Clear Errors.vi"("error in (no error)"=w1427) -> ("error out"=w1424:errorcluster)  [unwired: 5 in, 1 out]
                    n455 = call <vilib>:"connect.vi"("Use Rack/Slot for S71200/1500"=TRUE, "Slot S7 300/400"=u8 1, "PLC Type"=PLC_Type."S7 1200" ("PLC Type 2"), "error in (no error)"=w1424, "IP address"=w1421) -> ("error out"=w1426:errorcluster, "S7 Connection out"=w1425:T5)  [unwired: 5 in]
                  }
                }
              }
            }
            n456 = Unbundle By Name(w1403) -> ("status"=w1406:bool)
            n457 = Not(x=w1406) -> (.not. x?=w1405:bool)
            "PLC 7" <- w1405
            n458 = global write "Global 1.vi" "PLC 7"(w1405) -> ()
          }
        }
        n459 = call "PADMINI_STOP_ALL.vi"("Enum"=enum16{"Read", "Write"}."Read") -> ("Boolean 2"=w1246:bool)  [unwired: 9 in, 1 out]
        n460 = local read "stop"() -> (w1245:bool)
        n461 = Or(x=w1245, y=w1246) -> (x .or. y?=w1244:bool)
        n462 = Wait (ms)(milliseconds to wait=u32 1200) -> ()  [unwired: 1 out]
      }
      n463 = call <vilib>:"Clear Errors.vi"() -> ("error out"=w1220:errorcluster)  [unwired: 6 in, 1 out]
      n464 = call <vilib>:"disconnect.vi"("error in (no error)"=w1220, "S7 Connection in"=w1219) -> ()  [unwired: 8 in, 2 out]
    }
    frame Enabled {
      w1432 = PLC_Comm_State."Int"  # Enum
      n465 = while {
        shift-right: [w1447] -> _
        shift-left: w1432 -> [w1455]
        shift-right: [w1439] -> w1429
        shift-left: w1430 -> [w1454]
        shift-right: [w1450] -> _
        shift-left: _ -> [w1453]
        tunnel: w1431 -> [w1436]
        stop <- w1448 stop-if-true
        w1444 = PLC_Comm_State."Disconnect"  # Enum
        w1452 = u32 800  # milliseconds to wait
        # "Int-->Write-->Read---if--Error-->reconnect\n               ^------v                                       v\n                ^------------------------------v"
        # "OP 90-100"
        n466 = case shown="\"Error\"" w1455 {
          selector: w1455 -> [w1475 w1493 w1530 w1576 w1630 w1666 w1679 w1683 _ _]
          tunnel: [w1480 w1495 w1512 w1557 w1606 w1642 w1680 w1688 w1691 w1693] -> w1456
          tunnel: [w1481 w1494 w1511 w1556 w1607 w1643 w1681 w1685 w1690 w1692] -> w1449
          tunnel: w1454 -> [w1478 w1489 w1509 w1559 w1610 w1641 w1677 w1686 w1691 w1693]
          tunnel: w1453 -> [w1476 _ w1510 w1558 w1611 w1640 w1681 w1687 w1690 w1692]
          tunnel: [w1474 w1492 w1529 w1577 w1629 w1667 w1678 w1682 _ _] -> w1451
          tunnel: [_ _ _ _ _ _ _ TRUE _ _] -> w1448
          tunnel: [w1475 w1493 w1530 w1576 w1630 w1666 w1679 w1683 _ _] -> w1445
          tunnel: w1436 -> [w1473 w1491 _ _ _ _ _ _ _ _]
          frame "Connect" {
            w1474 = PLC_Comm_State."Write"  # Enum
            w1486 = TRUE  # Use Rack/Slot for S71200/1500
            w1485 = u8 1  # Slot S7 300/400
            w1483 = u8 0  # Rack S7 300/400
            # "Reconect"
            n467 = call <vilib>:"disconnect.vi"("error in (no error)"=w1478, "S7 Connection in"=w1476) -> ("error out"=w1479:errorcluster)  [unwired: 8 in, 1 out]
            n468 = call <vilib>:"Clear Errors.vi"("error in (no error)"=w1479) -> ("error out"=w1477:errorcluster)  [unwired: 5 in, 1 out]
            n469 = call <vilib>:"connect.vi"("Use Rack/Slot for S71200/1500"=w1486, "Slot S7 300/400"=w1485, "PLC Type"=PLC_Type."S7 1200" ("PLC Type 2"), "error in (no error)"=w1477, "Rack S7 300/400"=w1483, "timeout [ms]"=1000 ("timeout [ms] 2"), "IP address"=w1473) -> ("error out"=w1480:errorcluster, "S7 Connection out"=w1481:T5)  [unwired: 3 in]
          }
          frame "Int" {
            w1492 = PLC_Comm_State."Write"  # Enum
            w1496 = TRUE  # Use Rack/Slot for S71200/1500
            w1497 = u8 1  # Slot S7 300/400
            w1498 = u8 0  # Rack S7 300/400
            # "Initialize and set first bits"
            n470 = call "Stall Data Flow.vim"("value in"=w1489, "milliseconds to wait"=u32 774) -> ("value out"=w1488:errorcluster)  [unwired: 1 out]
            n471 = call <vilib>:"connect.vi"("Use Rack/Slot for S71200/1500"=w1496, "Slot S7 300/400"=w1497, "PLC Type"=PLC_Type."S7 1200" ("PLC Type 2"), "error in (no error)"=w1488, "Rack S7 300/400"=w1498, "timeout [ms]"=1000 ("timeout [ms] 2"), "IP address"=w1491) -> ("error out"=w1500:errorcluster, "S7 Connection out"=w1499:T5)  [unwired: 3 in]
            n472 = for {
              tunnel: u16[] [69, 71] ("Data Block #") -> [w1508] mode=indexing
              shift-right: [w1506] -> w1494
              shift-left: w1499 -> [w1504]
              tunnel: w1500 -> [w1505]
              tunnel: [w1503] -> w1495
              w1507 = i32[] [0, 0]  # DINT input array
              # "Reset Search and save \nbit on software start"
              n473 = call-poly <vilib>:"write DB.vi"("DINT input array"=w1507, "error in (no error)"=w1505, "Data Block #"=w1508, "S7 Connection in"=w1504) -> ("error out"=w1503:errorcluster, "S7 Connection out"=w1506:T5)  [unwired: 4 in, 2 out]
            }
          }
          frame "Write" {
            w1514 = u16 70 ("Data Block #")
            w1529 = PLC_Comm_State."Write2"  # Enum
            # "OP 90 Write"
            n474 = global read "DATA LOG.vi" "OP 90 Outputs"() -> (w1522:bool)
            n475 = case shown="True" w1522 {
              tunnel: [w1541 w1546] -> w1523
              tunnel: [w1542 w1547] -> w1524
              tunnel: w1510 -> [w1542 w1544]
              tunnel: w1509 -> [w1541 w1543]
              frame False {
              }
              frame True {
                w1555 = u16 70  # Data Block #
                n476 = call "PADMINI_AUTO_BARCODE_STATUS 90.vi"("Enum"=enum16{"Read", "Write"}."Read", "error in (no error)"=w1543) -> ("error out"=w1552:errorcluster, "O/P"=w1553:i32[])  [unwired: 8 in]
                n477 = call-poly <vilib>:"write DB.vi"("DINT input array"=w1553, "error in (no error)"=w1552, "Data Block #"=w1555, "S7 Connection in"=w1544) -> ("error out"=w1549:errorcluster, "S7 Connection out"=w1548:T5)  [unwired: 4 in, 2 out]
                n478 = call-poly <vilib>:"write DB.vi"("DINT input array"=i32[] [0] ("Data Byte"), "error in (no error)"=w1549, "Data Block #"=u16 69, "S7 Connection in"=w1548) -> ("error out"=w1546:errorcluster, "S7 Connection out"=w1547:T5)  [unwired: 4 in, 2 out]
                n479 = Unbundle By Name(w1546) -> ("status"=w1545:bool)
                n480 = global write "DATA LOG.vi" "OP 90 Outputs"(w1545) -> ()
              }
            }
            n481 = global read "DATA LOG.vi" "Auto Cycle On"() -> (w1518:bool)
            n482 = global read "DATA LOG.vi" "OP 90 reset"() -> (w1528:bool)
            n483 = Boolean To (0,1)(Boolean=w1518) -> (0, 1=w1517:i16)
            n484 = case shown="True" w1528 {
              tunnel: w1523 -> [w1531 w1537]
              tunnel: w1524 -> [w1532 w1536]
              tunnel: [w1532 w1535] -> w1525
              tunnel: [w1531 w1534] -> w1526
              frame False {
              }
              frame True {
                n485 = call-poly <vilib>:"write DB.vi"("Item offset [byte]"=u16 4 ("Data Block #"), "DINT input array"=i32[] [0], "error in (no error)"=w1537, "Data Block #"=u16 69, "S7 Connection in"=w1536) -> ("error out"=w1534:errorcluster, "S7 Connection out"=w1535:T5)  [unwired: 3 in, 2 out]
                n486 = Unbundle By Name(w1534) -> ("status"=w1533:bool)
                n487 = global write "DATA LOG.vi" "OP 90 reset"(w1533) -> ()
              }
            }
            n488 = Build Array(w1517) -> (w1527:i16[])
            n489 = global read "Global 1.vi" "Filtered BARCODE selected"() -> (w1521:string[])
            n490 = call-poly <vilib>:"write DB.vi"("Item offset [byte]"=u32 20, "DINT input array"=w1527, "error in (no error)"=w1526, "Data Block #"=w1514, "S7 Connection in"=w1525) -> ("error out"=w1520:errorcluster, "S7 Connection out"=w1519:T5)  [unwired: 3 in, 2 out]
            n491 = call-poly <vilib>:"write DB.vi"("Item offset [byte]"=u32 24, "Input STRINGS"=w1521, "error in (no error)"=w1520, "String length reserved in DB (default=254)"=u16 15, "Data Block #"=w1514, "S7 Connection in"=w1519) -> ("error out"=w1512:errorcluster, "S7 Connection out"=w1511:T5)  [unwired: 2 in, 2 out]
          }
          frame "Write2" {
            w1561 = u16 72 ("Data Block #")
            w1577 = PLC_Comm_State."Read"  # Enum
            # "op 100 wirte 2"
            n492 = global read "DATA LOG.vi" "OP 100 Outputs"() -> (w1575:bool)
            n493 = case shown="True" w1575 {
              tunnel: w1558 -> [w1588 w1601]
              tunnel: [w1589 w1591] -> w1573
              tunnel: [w1588 w1594] -> w1574
              tunnel: w1559 -> [w1589 w1598]
              frame False {
              }
              frame True {
                w1602 = u16 72  # Data Block #
                n494 = call "PADMINI_AUTO_BARCODE_STATUS 100.vi"("Enum"=enum16{"Read", "Write"}."Read", "error in (no error)"=w1598) -> ("error out"=w1597:errorcluster, "O/P"=w1599:i32[])  [unwired: 8 in]
                n495 = call-poly <vilib>:"write DB.vi"("DINT input array"=w1599, "error in (no error)"=w1597, "Data Block #"=w1602, "S7 Connection in"=w1601) -> ("error out"=w1593:errorcluster, "S7 Connection out"=w1592:T5)  [unwired: 4 in, 2 out]
                n496 = call-poly <vilib>:"write DB.vi"("DINT input array"=i32[] [0] ("Data Byte"), "error in (no error)"=w1593, "Data Block #"=u16 71, "S7 Connection in"=w1592) -> ("error out"=w1591:errorcluster, "S7 Connection out"=w1594:T5)  [unwired: 4 in, 2 out]
                n497 = Unbundle By Name(w1591) -> ("status"=w1590:bool)
                n498 = global write "DATA LOG.vi" "OP 100 Outputs"(w1590) -> ()
              }
            }
            n499 = global read "DATA LOG.vi" "OP 100 reset"() -> (w1572:bool)
            n500 = case shown="True" w1572 {
              tunnel: w1573 -> [w1578 w1587]
              tunnel: [w1578 w1581] -> w1568
              tunnel: w1574 -> [w1579 w1586]
              tunnel: [w1579 w1585] -> w1567
              frame False {
              }
              frame True {
                n501 = call-poly <vilib>:"write DB.vi"("Item offset [byte]"=u16 4 ("Data Block #"), "DINT input array"=i32[] [0], "error in (no error)"=w1587, "Data Block #"=u16 71, "S7 Connection in"=w1586) -> ("error out"=w1581:errorcluster, "S7 Connection out"=w1585:T5)  [unwired: 3 in, 2 out]
                n502 = Unbundle By Name(w1581) -> ("status"=w1580:bool)
                n503 = global write "DATA LOG.vi" "OP 100 reset"(w1580) -> ()
              }
            }
            n504 = global read "DATA LOG.vi" "Auto Cycle On"() -> (w1566:bool)
            n505 = global read "Global 1.vi" "Filtered BARCODE selected"() -> (w1569:string[])
            n506 = Boolean To (0,1)(Boolean=w1566) -> (0, 1=w1565:i16)
            n507 = Build Array(w1565) -> (w1564:i16[])
            n508 = call-poly <vilib>:"write DB.vi"("Item offset [byte]"=u32 20, "DINT input array"=w1564, "error in (no error)"=w1568, "Data Block #"=w1561, "S7 Connection in"=w1567) -> ("error out"=w1570:errorcluster, "S7 Connection out"=w1571:T5)  [unwired: 3 in, 2 out]
            n509 = call-poly <vilib>:"write DB.vi"("Item offset [byte]"=u32 24, "Input STRINGS"=w1569, "error in (no error)"=w1570, "String length reserved in DB (default=254)"=u16 15, "Data Block #"=w1561, "S7 Connection in"=w1571) -> ("error out"=w1557:errorcluster, "S7 Connection out"=w1556:T5)  [unwired: 2 in, 2 out]
          }
          frame "Read" {
            w1620 = u16 69 ("Data Block #")
            w1629 = PLC_Comm_State."Read2"  # Enum
            # "OP90 read"
            n510 = call-poly <vilib>:"read DB.vi"("Item offset [byte]"=u32 8, "error in (no error)"=w1610, "items #"=u16 2 ("Items # [byte]"), "Data Block #"=w1620, "S7 Connection in"=w1611) -> ("error out"=w1627:errorcluster, "REAL result array"=w1603:sgl[], "S7 Connection out"=w1628:T5)  [unwired: 4 in]
            n511 = call-poly <vilib>:"read DB.vi"("Item offset [byte]"=u32 16, "String length reserved in DB (default=254)"=u16 50, "error in (no error)"=w1627, "items #"=u16 1 ("Items # [byte]"), "Data Block #"=w1620, "S7 Connection in"=w1628) -> ("error out"=w1626:errorcluster, "STRING result Array"=w1624:string[], "S7 Connection out"=w1625:T5)  [unwired: 2 in, 1 out]
            n512 = call-poly <vilib>:"read DB.vi"("Item offset [byte]"=u32 68, "String length reserved in DB (default=254)"=u16 10, "error in (no error)"=w1626, "items #"=u16 3 ("Items # [byte]"), "Data Block #"=w1620, "S7 Connection in"=w1625) -> ("error out"=w1604:errorcluster, "STRING result Array"=w1623:string[], "S7 Connection out"=w1622:T5)  [unwired: 2 in, 1 out]
            n513 = Build Array (concatenate)(w1624, w1623) -> (w1609:string[])
            n514 = call-poly <vilib>:"read DB.vi"("error in (no error)"=w1604, "items #"=u16 2 ("Items # [byte]"), "Data Block #"=w1620, "S7 Connection in"=w1622) -> ("error out"=w1605:errorcluster, "DINT result array"=w1608:i32[], "S7 Connection out"=w1607:T5)  [unwired: 5 in]
            n515 = case shown="No Error" w1605 {
              selector: w1605 -> [w1633 w1639]
              tunnel: w1608 -> [w1638 _]
              tunnel: w1609 -> [w1637 _]
              tunnel: [w1632 w1639] -> w1606
              tunnel: w1603 -> [w1631 _]
              frame No Error {
                w1636 = enum16{"Read", "Write"}."Write" ("Enum")
                n516 = call "PADMINI_AUTO_CYCLE VALUE 90.vi"("Enum"=w1636, "error in (no error)"=w1633, "Input"=w1631) -> ("error out"=w1635:errorcluster)  [unwired: 7 in, 1 out]
                n517 = call "PADMINI_AUTO_BARCODE_STRING 90.vi"("Enum"=w1636, "error in (no error)"=w1635, "Input"=w1637) -> ("error out"=w1634:errorcluster)  [unwired: 7 in, 1 out]
                n518 = call "PADMINI_AUTO_CYCLE STATE 90.vi"("Enum"=w1636, "error in (no error)"=w1634, "Input"=w1638) -> ("error out"=w1632:errorcluster)  [unwired: 7 in, 1 out]
              }
              frame Error {
              }
            }
          }
          frame "Read2" {
            w1652 = u16 71 ("Data Block #")
            w1667 = PLC_Comm_State."Write"  # Enum
            # "Op100 Read2"
            n519 = call-poly <vilib>:"read DB.vi"("Item offset [byte]"=u32 8, "error in (no error)"=w1641, "items #"=u16 11 ("Items # [byte]"), "Data Block #"=w1652, "S7 Connection in"=w1640) -> ("error out"=w1663:errorcluster, "REAL result array"=w1665:sgl[], "S7 Connection out"=w1662:T5)  [unwired: 4 in]
            n520 = call-poly <vilib>:"read DB.vi"("Item offset [byte]"=u32 52, "String length reserved in DB (default=254)"=u16 50, "error in (no error)"=w1663, "items #"=u16 1 ("Items # [byte]"), "Data Block #"=w1652, "S7 Connection in"=w1662) -> ("error out"=w1660:errorcluster, "STRING result Array"=w1658:string[], "S7 Connection out"=w1659:T5)  [unwired: 2 in, 1 out]
            n521 = call-poly <vilib>:"read DB.vi"("Item offset [byte]"=u32 104, "String length reserved in DB (default=254)"=u16 10, "error in (no error)"=w1660, "items #"=u16 2 ("Items # [byte]"), "Data Block #"=w1652, "S7 Connection in"=w1659) -> ("error out"=w1661:errorcluster, "STRING result Array"=w1657:string[], "S7 Connection out"=w1654:T5)  [unwired: 2 in, 1 out]
            n522 = Build Array (concatenate)(w1658, w1657) -> (w1664:string[])
            n523 = call-poly <vilib>:"read DB.vi"("error in (no error)"=w1661, "items #"=u16 2 ("Items # [byte]"), "Data Block #"=w1652, "S7 Connection in"=w1654) -> ("error out"=w1655:errorcluster, "DINT result array"=w1656:i32[], "S7 Connection out"=w1643:T5)  [unwired: 5 in]
            n524 = case shown="No Error" w1655 {
              selector: w1655 -> [w1672 w1676]
              tunnel: w1656 -> [w1675 _]
              tunnel: w1664 -> [w1670 _]
              tunnel: w1665 -> [w1669 _]
              tunnel: [w1668 w1676] -> w1642
              frame No Error {
                w1671 = enum16{"Read", "Write"}."Write" ("Enum")
                n525 = call "PADMINI_AUTO_CYCLE VALUE 100.vi"("Enum"=w1671, "error in (no error)"=w1672, "Input"=w1669) -> ("error out"=w1673:errorcluster)  [unwired: 7 in, 1 out]
                n526 = call "PADMINI_AUTO_BARCODE_STRING 100.vi"("Enum"=w1671, "error in (no error)"=w1673, "Input"=w1670) -> ("error out"=w1674:errorcluster)  [unwired: 7 in, 1 out]
                n527 = call "PADMINI_AUTO_CYCLE STATE 100.vi"("Enum"=w1671, "error in (no error)"=w1674, "Input"=w1675) -> ("error out"=w1668:errorcluster)  [unwired: 7 in, 1 out]
              }
              frame Error {
              }
            }
          }
          frame "Error" {
            w1678 = PLC_Comm_State."Write"  # Enum
            n528 = global write "Global 1.vi" "PLC7 error"(w1677) -> ()
            n529 = call <vilib>:"Clear Errors.vi"("error in (no error)"=w1677) -> ("error out"=w1680:errorcluster)  [unwired: 5 in, 1 out]
          }
          frame "Disconnect" {
            w1682 = PLC_Comm_State."Disconnect"  # Enum
            w1685 = T5 {"TCP Connection Ref"=refnum, "IP address"="", "timeout ms"=5000, "Connected?"=FALSE, "PLC Type"=enum."S7 1200", "Rack S7 400"=0, "Slot S7 400"=0, "PDU Size"=0, "connection semaphore"=refnum}  # S7 Connection out
            n530 = call <vilib>:"Clear Errors.vi"("error in (no error)"=w1686) -> ("error out"=w1689:errorcluster)  [unwired: 5 in, 1 out]
            n531 = call <vilib>:"disconnect.vi"("error in (no error)"=w1689, "S7 Connection in"=w1687) -> ("error out"=w1688:errorcluster)  [unwired: 8 in, 1 out]
          }
          frame "Write3" {
            # "No Use"
          }
          frame "Read3" {
            # "No Use"
          }
        }
        n532 = Tick Count (ms)() -> (millisecond timer value=w1435:u32)
        n533 = feedback #4() -> (w1434:u32)  [unwired: 1 in]
        n534 = feedback-in #4(w1435) -> ()
        n535 = Subtract(x=w1435, y=w1434) -> (x-y=w1433:u32)
        n536 = global write "Global 1.vi" "Loop Time PLC 7"(w1433) -> ()
        n537 = Wait (ms)(milliseconds to wait=w1452) -> ()  [unwired: 1 out]
        n538 = call "PADMINI_STOP_ALL.vi"("Enum"=enum16{"Read", "Write"}."Read") -> ("Boolean 2"=w1443:bool)  [unwired: 9 in, 1 out]
        n539 = local read "stop"() -> (w1438:bool)
        n540 = case shown="Error" w1456 {
          selector: w1456 -> [w1459 w1460]
          tunnel: [w1459 w1466] -> w1439
          tunnel: [w1458 w1462] -> w1446
          tunnel: w1451 -> [w1458 _]
          tunnel: [w1457 w1472] -> w1450
          tunnel: w1449 -> [w1457 w1472]
          tunnel: w1445 -> [_ w1470]
          frame No Error {
          }
          frame Error {
            w1463 = PLC_Comm_State."Connect"  # Enum
            w1461 = PLC_Comm_State."Error"  # Enum
            n541 = Unbundle By Name(w1460) -> ("source"=w1471:string)
            n542 = call <userlib>:"Get Strings from Enum__ogtk.vi"("Enum"=w1470) -> ("String Value"=w1469:string)  [unwired: 7 in, 3 out]
            n543 = Concatenate Strings(w1469, "    " ("string"), w1471) -> (w1467:string)
            n544 = Bundle By Name(cluster=w1460, "source"=w1467) -> (w1466:errorcluster)
            n545 = call <vilib>:"Clear Errors.vi"("error in (no error)"=w1460, "specific error code to clear (0: all)"=6002) -> ("specific error cleared?"=w1465:bool)  [unwired: 4 in, 1 out]
            n546 = Select(t=w1463, s=w1465, f=w1461) -> (s? t:f=w1462:T1)
          }
        }
        n547 = Or(x=w1438, y=w1443) -> (x .or. y?=w1441:bool)
        n548 = Select(t=w1444, s=w1441, f=w1446) -> (s? t:f=w1447:T1)
        n549 = Unbundle By Name(w1439) -> ("status"=w1440:bool)
        n550 = Not(x=w1440) -> (.not. x?=w1437:bool)
        n551 = global write "Global 1.vi" "PLC 7"(w1437) -> ()
      }
    }
  }
  n552 = disable-structure shown="Enabled" {
    disable-tunnel: w71 -> [w1706 w1831]
    disable-tunnel: w9 -> [w1699 w1830]
    disable-tunnel: [w1694 w1829] -> w4
    frame Disabled {
      w1696 = TRUE  # Use Rack/Slot for S71200/1500
      w1697 = u8 1  # Slot S7 300/400
      w1698 = u8 0  # Rack S7 300/400
      w1705 = i32[] [0, 0]  # DINT input array
      # "Reset Search and save \nbit on software start"
      n553 = call <vilib>:"connect.vi"("Use Rack/Slot for S71200/1500"=w1696, "Slot S7 300/400"=w1697, "PLC Type"=PLC_Type."S7 1200" ("PLC Type 2"), "error in (no error)"=w1699, "Rack S7 300/400"=w1698, "timeout [ms]"=1000 ("timeout [ms] 2"), "IP address"=w1706) -> ("error out"=w1701:errorcluster, "S7 Connection out"=w1700:T5)  [unwired: 3 in]
      n554 = call-poly <vilib>:"write DB.vi"("DINT input array"=w1705, "error in (no error)"=w1701, "Data Block #"=u16 56, "S7 Connection in"=w1700) -> ("error out"=w1702:errorcluster, "S7 Connection out"=w1703:T5)  [unwired: 4 in, 2 out]
      n555 = while {
        shift-right: [w1713] -> w1710
        shift-left: w1703 -> [w1723]
        shift-right: [w1721] -> w1709
        shift-left: w1702 -> [w1722]
        tunnel: w1706 -> [w1712]
        stop <- w1715 stop-if-true
        # "OP 50"
        n556 = flat-sequence {
          tunnel: [w1726] -> w1719
          tunnel: [w1724] -> w1714
          tunnel: w1722 -> [w1774]
          tunnel: w1723 -> [w1773]
          tunnel: w1712 -> [w1761]
          tunnel: [w1761] -> w1711
          tunnel: [w1802] -> w1721
          tunnel: [w1801] -> w1713
          tunnel: w1719 -> [w1804]
          tunnel: w1714 -> [w1803]
          tunnel: w1711 -> [w1800]
          frame #0 {
            w1744 = u16 57 ("Data Block #")
            w1752 = u16 56 ("Data Block #")
            # "AUTO WRITE"
            n557 = global read "DATA LOG.vi" "OP 50 Outputs"() -> (w1772:bool)
            n558 = case shown="True" w1772 {
              tunnel: w1773 -> [w1785 w1798]
              tunnel: [w1786 w1787] -> w1760
              tunnel: [w1785 w1790] -> w1759
              tunnel: w1774 -> [w1786 w1795]
              frame False {
              }
              frame True {
                w1799 = u16 57  # Data Block #
                n559 = call "PADMINI_AUTO_BARCODE_STATUS 50.vi"("Enum"=enum16{"Read", "Write"}."Read", "error in (no error)"=w1795) -> ("error out"=w1794:errorcluster, "O/P"=w1796:i32[])  [unwired: 8 in]
                n560 = global write "DATA LOG.vi" "OP 50 Outputs"(FALSE) -> ()
                n561 = call-poly <vilib>:"write DB.vi"("DINT input array"=w1796, "error in (no error)"=w1794, "Data Block #"=w1799, "S7 Connection in"=w1798) -> ("error out"=w1788:errorcluster, "S7 Connection out"=w1789:T5)  [unwired: 4 in, 2 out]
                n562 = call-poly <vilib>:"write DB.vi"("DINT input array"=i32[] [0] ("Data Byte"), "error in (no error)"=w1788, "Data Block #"=u16 56, "S7 Connection in"=w1789) -> ("error out"=w1787:errorcluster, "S7 Connection out"=w1790:T5)  [unwired: 4 in, 2 out]
              }
            }
            n563 = global read "DATA LOG.vi" "OP 50 reset"() -> (w1758:bool)
            n564 = global read "DATA LOG.vi" "Auto Cycle On"() -> (w1735:bool)
            n565 = case shown="True" w1758 {
              tunnel: w1760 -> [w1775 w1784]
              tunnel: [w1775 w1783] -> w1737
              tunnel: w1759 -> [w1776 w1782]
              tunnel: [w1776 w1781] -> w1740
              frame False {
              }
              frame True {
                n566 = global write "DATA LOG.vi" "OP 50 reset"(FALSE) -> ()
                n567 = call-poly <vilib>:"write DB.vi"("Item offset [byte]"=u16 4 ("Data Block #"), "DINT input array"=i32[] [0], "error in (no error)"=w1784, "Data Block #"=u16 56, "S7 Connection in"=w1782) -> ("error out"=w1783:errorcluster, "S7 Connection out"=w1781:T5)  [unwired: 3 in, 2 out]
              }
            }
            n568 = Boolean To (0,1)(Boolean=w1735) -> (0, 1=w1734:i16)
            n569 = Build Array(w1734) -> (w1733:i16[])
            n570 = global read "Global 1.vi" "Filtered BARCODE selected"() -> (w1741:string[])
            n571 = call-poly <vilib>:"write DB.vi"("Item offset [byte]"=u32 20, "DINT input array"=w1733, "error in (no error)"=w1737, "Data Block #"=w1744, "S7 Connection in"=w1740) -> ("error out"=w1746:errorcluster, "S7 Connection out"=w1747:T5)  [unwired: 3 in, 2 out]
            n572 = call-poly <vilib>:"write DB.vi"("Item offset [byte]"=u32 24, "Input STRINGS"=w1741, "error in (no error)"=w1746, "String length reserved in DB (default=254)"=u16 15, "Data Block #"=w1744, "S7 Connection in"=w1747) -> ("error out"=w1738:errorcluster, "S7 Connection out"=w1739:T5)  [unwired: 2 in, 2 out]
            n573 = call-poly <vilib>:"read DB.vi"("Item offset [byte]"=u32 8, "error in (no error)"=w1738, "items #"=u16 3 ("Items # [byte]"), "Data Block #"=w1752, "S7 Connection in"=w1739) -> ("error out"=w1764:errorcluster, "REAL result array"=w1762:sgl[], "S7 Connection out"=w1770:T5)  [unwired: 4 in]
            n574 = call "PADMINI_AUTO_CYCLE VALUE 50.vi"("Enum"=enum16{"Read", "Write"}."Write", "error in (no error)"=w1764, "Input"=w1762) -> ("error out"=w1763:errorcluster)  [unwired: 7 in, 1 out]
            n575 = call-poly <vilib>:"read DB.vi"("Item offset [byte]"=u32 20, "String length reserved in DB (default=254)"=u16 50, "error in (no error)"=w1763, "items #"=u16 1 ("Items # [byte]"), "Data Block #"=w1752, "S7 Connection in"=w1770) -> ("error out"=w1754:errorcluster, "STRING result Array"=w1751:string[], "S7 Connection out"=w1753:T5)  [unwired: 2 in, 1 out]
            n576 = call-poly <vilib>:"read DB.vi"("Item offset [byte]"=u32 72, "String length reserved in DB (default=254)"=u16 10, "error in (no error)"=w1754, "items #"=u16 5 ("Items # [byte]"), "Data Block #"=w1752, "S7 Connection in"=w1753) -> ("error out"=w1755:errorcluster, "STRING result Array"=w1750:string[], "S7 Connection out"=w1727:T5)  [unwired: 2 in, 1 out]
            n577 = Build Array (concatenate)(w1751, w1750) -> (w1749:string[])
            n578 = call "PADMINI_AUTO_BARCODE_STRING 50.vi"("Enum"=enum16{"Read", "Write"}."Write", "error in (no error)"=w1755, "Input"=w1749) -> ("error out"=w1725:errorcluster)  [unwired: 7 in, 1 out]
            n579 = call-poly <vilib>:"read DB.vi"("error in (no error)"=w1725, "items #"=u16 2 ("Items # [byte]"), "Data Block #"=u16 56, "S7 Connection in"=w1727) -> ("error out"=w1729:errorcluster, "DINT result array"=w1731:i32[], "S7 Connection out"=w1726:T5)  [unwired: 5 in]
            n580 = call "PADMINI_AUTO_CYCLE STATE 50.vi"("Enum"=enum16{"Read", "Write"}."Write", "error in (no error)"=w1729, "Input"=w1731) -> ("error out"=w1724:errorcluster)  [unwired: 7 in, 1 out]
          }
          frame #1 {
            # "RECONNECT"
            n581 = case shown="Error" w1803 {
              selector: w1803 -> [w1808 w1809]
              tunnel: [w1807 w1813] -> w1801
              tunnel: [w1808 w1814] -> w1802
              tunnel: w1804 -> [w1807 w1812]
              tunnel: w1800 -> [_ w1811]
              frame No Error {
              }
              frame Error {
                n582 = Unbundle By Name(w1809) -> ("code"=w1810:i32)
                n583 = call <vilib>:"Clear Errors.vi"("error in (no error)"=w1809) -> ("error out"=w1815:errorcluster)  [unwired: 5 in, 1 out]
                n584 = case shown="1, 66" w1810 {
                  tunnel: w1815 -> [w1817 w1828]
                  tunnel: [w1817 w1826] -> w1814
                  tunnel: [w1818 w1825] -> w1813
                  tunnel: w1812 -> [w1818 w1822]
                  tunnel: w1811 -> [_ w1821]
                  tunnel: w1809 -> [w1816 _]
                  frame 0, Default {
                    n585 = global write "Global 1.vi" "PLC4 error"(w1816) -> ()
                  }
                  frame 1, 66 {
                    n586 = call <vilib>:"disconnect.vi"("error in (no error)"=w1828, "S7 Connection in"=w1822) -> ("error out"=w1827:errorcluster)  [unwired: 8 in, 1 out]
                    n587 = call <vilib>:"Clear Errors.vi"("error in (no error)"=w1827) -> ("error out"=w1824:errorcluster)  [unwired: 5 in, 1 out]
                    n588 = call <vilib>:"connect.vi"("Use Rack/Slot for S71200/1500"=TRUE, "Slot S7 300/400"=u8 1, "PLC Type"=PLC_Type."S7 1200" ("PLC Type 2"), "error in (no error)"=w1824, "IP address"=w1821) -> ("error out"=w1826:errorcluster, "S7 Connection out"=w1825:T5)  [unwired: 5 in]
                  }
                }
              }
            }
            n589 = Unbundle By Name(w1803) -> ("status"=w1806:bool)
            n590 = Not(x=w1806) -> (.not. x?=w1805:bool)
            "PLC 4" <- w1805
            n591 = global write "Global 1.vi" "PLC 4"(w1805) -> ()
          }
        }
        n592 = call "PADMINI_STOP_ALL.vi"("Enum"=enum16{"Read", "Write"}."Read") -> ("Boolean 2"=w1717:bool)  [unwired: 9 in, 1 out]
        n593 = local read "stop"() -> (w1716:bool)
        n594 = Or(x=w1716, y=w1717) -> (x .or. y?=w1715:bool)
        n595 = Wait (ms)(milliseconds to wait=u32 1200) -> ()  [unwired: 1 out]
      }
      n596 = call <vilib>:"Clear Errors.vi"("error in (no error)"=w1709) -> ("error out"=w1695:errorcluster)  [unwired: 5 in, 1 out]
      n597 = call <vilib>:"disconnect.vi"("error in (no error)"=w1695, "S7 Connection in"=w1710) -> ("error out"=w1694:errorcluster)  [unwired: 8 in, 1 out]
    }
    frame Enabled {
      w1832 = PLC_Comm_State."Int"  # Enum
      n598 = while {
        shift-right: [w1847] -> _
        shift-left: w1832 -> [w1855]
        shift-right: [w1839] -> w1829
        shift-left: w1830 -> [w1854]
        shift-right: [w1850] -> _
        shift-left: _ -> [w1853]
        tunnel: w1831 -> [w1836]
        stop <- w1848 stop-if-true
        w1844 = PLC_Comm_State."Disconnect"  # Enum
        w1852 = u32 800  # milliseconds to wait
        # "Int-->Write-->Read---if--Error-->reconnect\n               ^------v                                       v\n                ^------------------------------v"
        # "OP 50"
        n599 = case shown="\"Error\"" w1855 {
          selector: w1855 -> [w1875 w1892 w1930 w1983 w1995 w1998 _ _ _ _]
          tunnel: [w1880 w1894 w1910 w1958 w1994 w2003 w2005 w2008 w2010 w2012] -> w1856
          tunnel: [w1881 w1893 w1909 w1957 w1996 w2000 w2006 w2007 w2009 w2011] -> w1849
          tunnel: w1854 -> [w1878 w1888 w1911 w1959 w1994 w2001 w2005 w2008 w2010 w2012]
          tunnel: w1853 -> [w1876 _ w1912 w1956 w1996 w2002 w2006 w2007 w2009 w2011]
          tunnel: [w1874 w1891 w1929 w1982 w1993 w1997 _ _ _ _] -> w1851
          tunnel: [_ _ _ _ _ TRUE _ _ _ _] -> w1848
          tunnel: [w1875 w1892 w1930 w1983 w1995 w1998 _ _ _ _] -> w1845
          tunnel: w1836 -> [w1873 w1890 _ _ _ _ _ _ _ _]
          frame "Connect" {
            w1874 = PLC_Comm_State."Write"  # Enum
            w1886 = TRUE  # Use Rack/Slot for S71200/1500
            w1885 = u8 1  # Slot S7 300/400
            w1883 = u8 0  # Rack S7 300/400
            # "Reconect"
            n600 = call <vilib>:"disconnect.vi"("error in (no error)"=w1878, "S7 Connection in"=w1876) -> ("error out"=w1879:errorcluster)  [unwired: 8 in, 1 out]
            n601 = call <vilib>:"Clear Errors.vi"("error in (no error)"=w1879) -> ("error out"=w1877:errorcluster)  [unwired: 5 in, 1 out]
            n602 = call <vilib>:"connect.vi"("Use Rack/Slot for S71200/1500"=w1886, "Slot S7 300/400"=w1885, "PLC Type"=PLC_Type."S7 1200" ("PLC Type 2"), "error in (no error)"=w1877, "Rack S7 300/400"=w1883, "timeout [ms]"=1000 ("timeout [ms] 2"), "IP address"=w1873) -> ("error out"=w1880:errorcluster, "S7 Connection out"=w1881:T5)  [unwired: 3 in]
          }
          frame "Int" {
            w1891 = PLC_Comm_State."Write"  # Enum
            w1895 = TRUE  # Use Rack/Slot for S71200/1500
            w1896 = u8 1  # Slot S7 300/400
            w1897 = u8 0  # Rack S7 300/400
            w1898 = u16[] [56]  # Data Block #
            # "Initialize and set first bits"
            n603 = call "Stall Data Flow.vim"("value in"=w1888, "milliseconds to wait"=u32 387) -> ("value out"=w1887:errorcluster)  [unwired: 1 out]
            n604 = call <vilib>:"connect.vi"("Use Rack/Slot for S71200/1500"=w1895, "Slot S7 300/400"=w1896, "PLC Type"=PLC_Type."S7 1200" ("PLC Type 2"), "error in (no error)"=w1887, "Rack S7 300/400"=w1897, "timeout [ms]"=1000 ("timeout [ms] 2"), "IP address"=w1890) -> ("error out"=w1900:errorcluster, "S7 Connection out"=w1899:T5)  [unwired: 3 in]
            n605 = for {
              tunnel: w1898 -> [w1908] mode=indexing
              shift-right: [w1906] -> w1893
              shift-left: w1899 -> [w1904]
              tunnel: w1900 -> [w1905]
              tunnel: [w1903] -> w1894
              w1907 = i32[] [0, 0]  # DINT input array
              # "Reset Search and save \nbit on software start"
              n606 = call-poly <vilib>:"write DB.vi"("DINT input array"=w1907, "error in (no error)"=w1905, "Data Block #"=w1908, "S7 Connection in"=w1904) -> ("error out"=w1903:errorcluster, "S7 Connection out"=w1906:T5)  [unwired: 4 in, 2 out]
            }
          }
          frame "Write" {
            w1914 = u16 57 ("Data Block #")
            w1929 = PLC_Comm_State."Read"  # Enum
            n607 = global read "DATA LOG.vi" "OP 50 Outputs"() -> (w1928:bool)
            n608 = case shown="True" w1928 {
              tunnel: w1912 -> [w1941 w1954]
              tunnel: [w1942 w1944] -> w1927
              tunnel: [w1941 w1947] -> w1926
              tunnel: w1911 -> [w1942 w1951]
              frame False {
              }
              frame True {
                w1955 = u16 57  # Data Block #
                n609 = call "PADMINI_AUTO_BARCODE_STATUS 50.vi"("Enum"=enum16{"Read", "Write"}."Read", "error in (no error)"=w1951) -> ("error out"=w1950:errorcluster, "O/P"=w1952:i32[])  [unwired: 8 in]
                n610 = call-poly <vilib>:"write DB.vi"("DINT input array"=w1952, "error in (no error)"=w1950, "Data Block #"=w1955, "S7 Connection in"=w1954) -> ("error out"=w1945:errorcluster, "S7 Connection out"=w1946:T5)  [unwired: 4 in, 2 out]
                n611 = call-poly <vilib>:"write DB.vi"("DINT input array"=i32[] [0] ("Data Byte"), "error in (no error)"=w1945, "Data Block #"=u16 56, "S7 Connection in"=w1946) -> ("error out"=w1944:errorcluster, "S7 Connection out"=w1947:T5)  [unwired: 4 in, 2 out]
                n612 = Unbundle By Name(w1944) -> ("status"=w1943:bool)
                n613 = global write "DATA LOG.vi" "OP 50 Outputs"(w1943) -> ()
              }
            }
            n614 = global read "DATA LOG.vi" "OP 50 reset"() -> (w1925:bool)
            n615 = case shown="True" w1925 {
              tunnel: w1927 -> [w1931 w1940]
              tunnel: [w1931 w1934] -> w1920
              tunnel: w1926 -> [w1932 w1939]
              tunnel: [w1932 w1938] -> w1921
              frame False {
              }
              frame True {
                n616 = call-poly <vilib>:"write DB.vi"("Item offset [byte]"=u16 4 ("Data Block #"), "DINT input array"=i32[] [0], "error in (no error)"=w1940, "Data Block #"=u16 56, "S7 Connection in"=w1939) -> ("error out"=w1934:errorcluster, "S7 Connection out"=w1938:T5)  [unwired: 3 in, 2 out]
                n617 = Unbundle By Name(w1934) -> ("status"=w1933:bool)
                n618 = global write "DATA LOG.vi" "OP 50 reset"(w1933) -> ()
              }
            }
            n619 = global read "DATA LOG.vi" "Auto Cycle On"() -> (w1919:bool)
            n620 = global read "Global 1.vi" "Filtered BARCODE selected"() -> (w1922:string[])
            n621 = Boolean To (0,1)(Boolean=w1919) -> (0, 1=w1918:i16)
            n622 = Build Array(w1918) -> (w1917:i16[])
            n623 = call-poly <vilib>:"write DB.vi"("Item offset [byte]"=u32 20, "DINT input array"=w1917, "error in (no error)"=w1920, "Data Block #"=w1914, "S7 Connection in"=w1921) -> ("error out"=w1923:errorcluster, "S7 Connection out"=w1924:T5)  [unwired: 3 in, 2 out]
            n624 = call-poly <vilib>:"write DB.vi"("Item offset [byte]"=u32 24, "Input STRINGS"=w1922, "error in (no error)"=w1923, "String length reserved in DB (default=254)"=u16 15, "Data Block #"=w1914, "S7 Connection in"=w1924) -> ("error out"=w1910:errorcluster, "S7 Connection out"=w1909:T5)  [unwired: 2 in, 2 out]
          }
          frame "Read" {
            w1968 = u16 56 ("Data Block #")
            w1982 = PLC_Comm_State."Write"  # Enum
            # "OP 50 Read"
            n625 = call-poly <vilib>:"read DB.vi"("error in (no error)"=w1959, "items #"=u16 2 ("Items # [byte]"), "Data Block #"=w1968, "S7 Connection in"=w1956) -> ("error out"=w1980:errorcluster, "DINT result array"=w1976:i32[], "S7 Connection out"=w1979:T5)  [unwired: 5 in]
            n626 = call-poly <vilib>:"read DB.vi"("Item offset [byte]"=u32 8, "error in (no error)"=w1980, "items #"=u16 3 ("Items # [byte]"), "Data Block #"=w1968, "S7 Connection in"=w1979) -> ("error out"=w1974:errorcluster, "REAL result array"=w1978:sgl[], "S7 Connection out"=w1975:T5)  [unwired: 4 in]
            n627 = call-poly <vilib>:"read DB.vi"("Item offset [byte]"=u32 20, "String length reserved in DB (default=254)"=u16 50, "error in (no error)"=w1974, "items #"=u16 1 ("Items # [byte]"), "Data Block #"=w1968, "S7 Connection in"=w1975) -> ("error out"=w1973:errorcluster, "STRING result Array"=w1971:string[], "S7 Connection out"=w1972:T5)  [unwired: 2 in, 1 out]
            n628 = call-poly <vilib>:"read DB.vi"("Item offset [byte]"=u32 72, "String length reserved in DB (default=254)"=u16 10, "error in (no error)"=w1973, "items #"=u16 5 ("Items # [byte]"), "Data Block #"=w1968, "S7 Connection in"=w1972) -> ("error out"=w1981:errorcluster, "STRING result Array"=w1970:string[], "S7 Connection out"=w1957:T5)  [unwired: 2 in, 1 out]
            n629 = Build Array (concatenate)(w1971, w1970) -> (w1977:string[])
            n630 = case shown="No Error" w1981 {
              selector: w1981 -> [w1987 w1992]
              tunnel: w1976 -> [w1991 _]
              tunnel: w1977 -> [w1989 _]
              tunnel: w1978 -> [w1986 _]
              tunnel: [w1985 w1992] -> w1958
              frame No Error {
                w1984 = enum16{"Read", "Write"}."Write" ("Enum")
                n631 = call "PADMINI_AUTO_CYCLE VALUE 50.vi"("Enum"=w1984, "error in (no error)"=w1987, "Input"=w1986) -> ("error out"=w1988:errorcluster)  [unwired: 7 in, 1 out]
                n632 = call "PADMINI_AUTO_BARCODE_STRING 50.vi"("Enum"=w1984, "error in (no error)"=w1988, "Input"=w1989) -> ("error out"=w1990:errorcluster)  [unwired: 7 in, 1 out]
                n633 = call "PADMINI_AUTO_CYCLE STATE 50.vi"("Enum"=w1984, "error in (no error)"=w1990, "Input"=w1991) -> ("error out"=w1985:errorcluster)  [unwired: 7 in, 1 out]
              }
              frame Error {
              }
            }
          }
          frame "Error" {
            w1993 = PLC_Comm_State."Write"  # Enum
            n634 = global write "Global 1.vi" "PLC4 error"(w1994) -> ()
          }
          frame "Disconnect" {
            w1997 = PLC_Comm_State."Disconnect"  # Enum
            w2000 = T5 {"TCP Connection Ref"=refnum, "IP address"="", "timeout ms"=5000, "Connected?"=FALSE, "PLC Type"=enum."S7 1200", "Rack S7 400"=0, "Slot S7 400"=0, "PDU Size"=0, "connection semaphore"=refnum}  # S7 Connection out
            n635 = call <vilib>:"Clear Errors.vi"("error in (no error)"=w2001) -> ("error out"=w2004:errorcluster)  [unwired: 5 in, 1 out]
            n636 = call <vilib>:"disconnect.vi"("error in (no error)"=w2004, "S7 Connection in"=w2002) -> ("error out"=w2003:errorcluster)  [unwired: 8 in, 1 out]
          }
          frame "Write2" {
            # "No Use"
          }
          frame "Write3" {
            # "No Use"
          }
          frame "Read2" {
            # "No Use"
          }
          frame "Read3" {
            # "No Use"
          }
        }
        n637 = Tick Count (ms)() -> (millisecond timer value=w1835:u32)
        n638 = feedback #5() -> (w1834:u32)  [unwired: 1 in]
        n639 = feedback-in #5(w1835) -> ()
        n640 = Subtract(x=w1835, y=w1834) -> (x-y=w1833:u32)
        n641 = global write "Global 1.vi" "Loop Time PLC 4"(w1833) -> ()
        n642 = Wait (ms)(milliseconds to wait=w1852) -> ()  [unwired: 1 out]
        n643 = call "PADMINI_STOP_ALL.vi"("Enum"=enum16{"Read", "Write"}."Read") -> ("Boolean 2"=w1843:bool)  [unwired: 9 in, 1 out]
        n644 = local read "stop"() -> (w1838:bool)
        n645 = case shown="Error" w1856 {
          selector: w1856 -> [w1859 w1863]
          tunnel: [w1859 w1866] -> w1839
          tunnel: [w1858 w1860] -> w1846
          tunnel: w1851 -> [w1858 _]
          tunnel: [w1857 w1872] -> w1850
          tunnel: w1849 -> [w1857 w1872]
          tunnel: w1845 -> [_ w1870]
          frame No Error {
          }
          frame Error {
            w1861 = PLC_Comm_State."Connect"  # Enum
            w1862 = PLC_Comm_State."Error"  # Enum
            n646 = Unbundle By Name(w1863) -> ("source"=w1871:string)
            n647 = call <userlib>:"Get Strings from Enum__ogtk.vi"("Enum"=w1870) -> ("String Value"=w1869:string)  [unwired: 7 in, 3 out]
            n648 = Concatenate Strings(w1869, "    " ("string"), w1871) -> (w1867:string)
            n649 = Bundle By Name(cluster=w1863, "source"=w1867) -> (w1866:errorcluster)
            n650 = call <vilib>:"Clear Errors.vi"("error in (no error)"=w1863, "specific error code to clear (0: all)"=6002) -> ("specific error cleared?"=w1865:bool)  [unwired: 4 in, 1 out]
            n651 = Select(t=w1861, s=w1865, f=w1862) -> (s? t:f=w1860:T1)
          }
        }
        n652 = Or(x=w1838, y=w1843) -> (x .or. y?=w1841:bool)
        n653 = Select(t=w1844, s=w1841, f=w1846) -> (s? t:f=w1847:T1)
        n654 = Unbundle By Name(w1839) -> ("status"=w1840:bool)
        n655 = Not(x=w1840) -> (.not. x?=w1837:bool)
        n656 = global write "Global 1.vi" "PLC 4"(w1837) -> ()
      }
    }
  }
  n657 = disable-structure shown="Enabled" {
    disable-tunnel: w61 -> [w2025 w2150]
    disable-tunnel: w9 -> [w2018 w2149]
    disable-tunnel: [w2013 w2148] -> w6
    frame Disabled {
      w2015 = TRUE  # Use Rack/Slot for S71200/1500
      w2016 = u8 1  # Slot S7 300/400
      w2017 = u8 0  # Rack S7 300/400
      w2023 = i32[] [0, 0]  # DINT input array
      # "Reset Search and save \nbit on software start"
      n658 = call <vilib>:"connect.vi"("Use Rack/Slot for S71200/1500"=w2015, "Slot S7 300/400"=w2016, "PLC Type"=PLC_Type."S7 1200" ("PLC Type 2"), "error in (no error)"=w2018, "Rack S7 300/400"=w2017, "timeout [ms]"=1000 ("timeout [ms] 2"), "IP address"=w2025) -> ("error out"=w2019:errorcluster, "S7 Connection out"=w2020:T5)  [unwired: 3 in]
      n659 = call-poly <vilib>:"write DB.vi"("DINT input array"=w2023, "error in (no error)"=w2019, "Data Block #"=u16 43, "S7 Connection in"=w2020) -> ("error out"=w2022:errorcluster, "S7 Connection out"=w2021:T5)  [unwired: 4 in, 2 out]
      n660 = while {
        shift-right: [w2032] -> w2026
        shift-left: w2021 -> [w2042]
        shift-right: [w2040] -> w2027
        shift-left: w2022 -> [w2041]
        tunnel: w2025 -> [w2031]
        stop <- w2034 stop-if-true
        # "OP 60"
        n661 = flat-sequence {
          tunnel: [w2045] -> w2038
          tunnel: [w2043] -> w2033
          tunnel: w2041 -> [w2093]
          tunnel: w2042 -> [w2092]
          tunnel: w2031 -> [w2080]
          tunnel: [w2080] -> w2030
          tunnel: [w2121] -> w2040
          tunnel: [w2120] -> w2032
          tunnel: w2038 -> [w2123]
          tunnel: w2033 -> [w2122]
          tunnel: w2030 -> [w2119]
          frame #0 {
            w2076 = u16 44 ("Data Block #")
            w2057 = u16 43 ("Data Block #")
            # "AUTO WRITE"
            n662 = global read "DATA LOG.vi" "OP 60 Outputs"() -> (w2091:bool)
            n663 = case shown="True" w2091 {
              tunnel: w2092 -> [w2104 w2117]
              tunnel: [w2105 w2106] -> w2068
              tunnel: [w2104 w2109] -> w2067
              tunnel: w2093 -> [w2105 w2114]
              frame False {
              }
              frame True {
                w2118 = u16 44  # Data Block #
                n664 = call "PADMINI_AUTO_BARCODE_STATUS 60.vi"("Enum"=enum16{"Read", "Write"}."Read", "error in (no error)"=w2114) -> ("error out"=w2113:errorcluster, "O/P"=w2115:i32[])  [unwired: 8 in]
                n665 = global write "DATA LOG.vi" "OP 60 Outputs"(FALSE) -> ()
                n666 = call-poly <vilib>:"write DB.vi"("DINT input array"=w2115, "error in (no error)"=w2113, "Data Block #"=w2118, "S7 Connection in"=w2117) -> ("error out"=w2107:errorcluster, "S7 Connection out"=w2108:T5)  [unwired: 4 in, 2 out]
                n667 = call-poly <vilib>:"write DB.vi"("DINT input array"=i32[] [0] ("Data Byte"), "error in (no error)"=w2107, "Data Block #"=u16 43, "S7 Connection in"=w2108) -> ("error out"=w2106:errorcluster, "S7 Connection out"=w2109:T5)  [unwired: 4 in, 2 out]
              }
            }
            n668 = global read "DATA LOG.vi" "OP 60 reset"() -> (w2066:bool)
            n669 = global read "DATA LOG.vi" "Auto Cycle On"() -> (w2054:bool)
            n670 = case shown="True" w2066 {
              tunnel: w2068 -> [w2094 w2103]
              tunnel: [w2094 w2102] -> w2069
              tunnel: w2067 -> [w2095 w2101]
              tunnel: [w2095 w2100] -> w2070
              frame False {
              }
              frame True {
                n671 = global write "DATA LOG.vi" "OP 60 reset"(FALSE) -> ()
                n672 = call-poly <vilib>:"write DB.vi"("Item offset [byte]"=u16 4 ("Data Block #"), "DINT input array"=i32[] [0], "error in (no error)"=w2103, "Data Block #"=u16 43, "S7 Connection in"=w2101) -> ("error out"=w2102:errorcluster, "S7 Connection out"=w2100:T5)  [unwired: 3 in, 2 out]
              }
            }
            n673 = Boolean To (0,1)(Boolean=w2054) -> (0, 1=w2053:i16)
            n674 = Build Array(w2053) -> (w2052:i16[])
            n675 = global read "Global 1.vi" "Filtered BARCODE selected"() -> (w2079:string[])
            n676 = call-poly <vilib>:"write DB.vi"("Item offset [byte]"=u32 20, "DINT input array"=w2052, "error in (no error)"=w2069, "Data Block #"=w2076, "S7 Connection in"=w2070) -> ("error out"=w2074:errorcluster, "S7 Connection out"=w2073:T5)  [unwired: 3 in, 2 out]
            n677 = call-poly <vilib>:"write DB.vi"("Item offset [byte]"=u32 24, "Input STRINGS"=w2079, "error in (no error)"=w2074, "String length reserved in DB (default=254)"=u16 15, "Data Block #"=w2076, "S7 Connection in"=w2073) -> ("error out"=w2071:errorcluster, "S7 Connection out"=w2072:T5)  [unwired: 2 in, 2 out]
            n678 = call-poly <vilib>:"read DB.vi"("Item offset [byte]"=u32 8, "error in (no error)"=w2071, "items #"=u16 6 ("Items # [byte]"), "Data Block #"=w2057, "S7 Connection in"=w2072) -> ("error out"=w2083:errorcluster, "REAL result array"=w2081:sgl[], "S7 Connection out"=w2089:T5)  [unwired: 4 in]
            n679 = call "PADMINI_AUTO_CYCLE VALUE 60.vi"("Enum"=enum16{"Read", "Write"}."Write", "error in (no error)"=w2083, "Input"=w2081) -> ("error out"=w2082:errorcluster)  [unwired: 7 in, 1 out]
            n680 = call-poly <vilib>:"read DB.vi"("Item offset [byte]"=u32 32, "String length reserved in DB (default=254)"=u16 50, "error in (no error)"=w2082, "items #"=u16 1 ("Items # [byte]"), "Data Block #"=w2057, "S7 Connection in"=w2089) -> ("error out"=w2061:errorcluster, "STRING result Array"=w2059:string[], "S7 Connection out"=w2060:T5)  [unwired: 2 in, 1 out]
            n681 = call-poly <vilib>:"read DB.vi"("Item offset [byte]"=u32 84, "String length reserved in DB (default=254)"=u16 10, "error in (no error)"=w2061, "items #"=u16 7 ("Items # [byte]"), "Data Block #"=w2057, "S7 Connection in"=w2060) -> ("error out"=w2062:errorcluster, "STRING result Array"=w2065:string[], "S7 Connection out"=w2046:T5)  [unwired: 2 in, 1 out]
            n682 = Build Array (concatenate)(w2059, w2065) -> (w2058:string[])
            n683 = call "PADMINI_AUTO_BARCODE_STRING 60.vi"("Enum"=enum16{"Read", "Write"}."Write", "error in (no error)"=w2062, "Input"=w2058) -> ("error out"=w2044:errorcluster)  [unwired: 7 in, 1 out]
            n684 = call-poly <vilib>:"read DB.vi"("error in (no error)"=w2044, "items #"=u16 2 ("Items # [byte]"), "Data Block #"=u16 43, "S7 Connection in"=w2046) -> ("error out"=w2051:errorcluster, "DINT result array"=w2049:i32[], "S7 Connection out"=w2045:T5)  [unwired: 5 in]
            n685 = call "PADMINI_AUTO_CYCLE STATE 60.vi"("Enum"=enum16{"Read", "Write"}."Write", "error in (no error)"=w2051, "Input"=w2049) -> ("error out"=w2043:errorcluster)  [unwired: 7 in, 1 out]
          }
          frame #1 {
            # "RECONNECT"
            n686 = case shown="Error" w2122 {
              selector: w2122 -> [w2127 w2128]
              tunnel: [w2126 w2132] -> w2120
              tunnel: [w2127 w2133] -> w2121
              tunnel: w2123 -> [w2126 w2131]
              tunnel: w2119 -> [_ w2130]
              frame No Error {
              }
              frame Error {
                n687 = Unbundle By Name(w2128) -> ("code"=w2129:i32)
                n688 = call <vilib>:"Clear Errors.vi"("error in (no error)"=w2128) -> ("error out"=w2134:errorcluster)  [unwired: 5 in, 1 out]
                n689 = case shown="0, Default" w2129 {
                  tunnel: w2134 -> [w2136 w2147]
                  tunnel: [w2136 w2145] -> w2133
                  tunnel: [w2137 w2144] -> w2132
                  tunnel: w2131 -> [w2137 w2141]
                  tunnel: w2130 -> [_ w2140]
                  tunnel: w2128 -> [w2135 _]
                  frame 0, Default {
                    n690 = global write "Global 1.vi" "PLC5 error"(w2135) -> ()
                  }
                  frame 1, 66 {
                    n691 = call <vilib>:"disconnect.vi"("error in (no error)"=w2147, "S7 Connection in"=w2141) -> ("error out"=w2146:errorcluster)  [unwired: 8 in, 1 out]
                    n692 = call <vilib>:"Clear Errors.vi"("error in (no error)"=w2146) -> ("error out"=w2143:errorcluster)  [unwired: 5 in, 1 out]
                    n693 = call <vilib>:"connect.vi"("Use Rack/Slot for S71200/1500"=TRUE, "Slot S7 300/400"=u8 1, "PLC Type"=PLC_Type."S7 1200" ("PLC Type 2"), "error in (no error)"=w2143, "IP address"=w2140) -> ("error out"=w2145:errorcluster, "S7 Connection out"=w2144:T5)  [unwired: 5 in]
                  }
                }
              }
            }
            n694 = Unbundle By Name(w2122) -> ("status"=w2125:bool)
            n695 = Not(x=w2125) -> (.not. x?=w2124:bool)
            "PLC 5" <- w2124
            n696 = global write "Global 1.vi" "PLC 5"(w2124) -> ()
          }
        }
        n697 = call "PADMINI_STOP_ALL.vi"("Enum"=enum16{"Read", "Write"}."Read") -> ("Boolean 2"=w2036:bool)  [unwired: 9 in, 1 out]
        n698 = local read "stop"() -> (w2035:bool)
        n699 = Or(x=w2035, y=w2036) -> (x .or. y?=w2034:bool)
        n700 = Wait (ms)(milliseconds to wait=u32 1200) -> ()  [unwired: 1 out]
      }
      n701 = call <vilib>:"Clear Errors.vi"("error in (no error)"=w2027) -> ("error out"=w2014:errorcluster)  [unwired: 5 in, 1 out]
      n702 = call <vilib>:"disconnect.vi"("error in (no error)"=w2014, "S7 Connection in"=w2026) -> ("error out"=w2013:errorcluster)  [unwired: 8 in, 1 out]
    }
    frame Enabled {
      w2151 = PLC_Comm_State."Int"  # Enum
      n703 = while {
        shift-right: [w2166] -> _
        shift-left: w2151 -> [w2174]
        shift-right: [w2158] -> w2148
        shift-left: w2149 -> [w2173]
        shift-right: [w2169] -> _
        shift-left: _ -> [w2172]
        tunnel: w2150 -> [w2155]
        stop <- w2167 stop-if-true
        w2163 = PLC_Comm_State."Disconnect"  # Enum
        w2171 = u32 800  # milliseconds to wait
        # "Int-->Write-->Read---if--Error-->reconnect\n               ^------v                                       v\n                ^------------------------------v"
        # "OP 60"
        n704 = case shown="\"Error\"" w2174 {
          selector: w2174 -> [w2194 w2211 w2249 w2303 w2315 w2319 _ _ _ _]
          tunnel: [w2199 w2213 w2228 w2278 w2316 w2324 w2326 w2329 w2331 w2333] -> w2175
          tunnel: [w2200 w2212 w2231 w2275 w2317 w2321 w2327 w2328 w2330 w2332] -> w2168
          tunnel: w2173 -> [w2197 w2208 w2229 w2277 w2313 w2322 w2326 w2329 w2331 w2333]
          tunnel: w2172 -> [w2195 _ w2230 w2276 w2317 w2323 w2327 w2328 w2330 w2332]
          tunnel: [w2193 w2210 w2248 w2302 w2314 w2318 _ _ _ _] -> w2170
          tunnel: [_ _ _ _ _ TRUE _ _ _ _] -> w2167
          tunnel: [w2194 w2211 w2249 w2303 w2315 w2319 _ _ _ _] -> w2164
          tunnel: w2155 -> [w2192 w2209 _ _ _ _ _ _ _ _]
          frame "Connect" {
            w2193 = PLC_Comm_State."Write"  # Enum
            w2205 = TRUE  # Use Rack/Slot for S71200/1500
            w2204 = u8 1  # Slot S7 300/400
            w2202 = u8 0  # Rack S7 300/400
            # "Reconect"
            n705 = call <vilib>:"disconnect.vi"("error in (no error)"=w2197, "S7 Connection in"=w2195) -> ("error out"=w2198:errorcluster)  [unwired: 8 in, 1 out]
            n706 = call <vilib>:"Clear Errors.vi"("error in (no error)"=w2198) -> ("error out"=w2196:errorcluster)  [unwired: 5 in, 1 out]
            n707 = call <vilib>:"connect.vi"("Use Rack/Slot for S71200/1500"=w2205, "Slot S7 300/400"=w2204, "PLC Type"=PLC_Type."S7 1200" ("PLC Type 2"), "error in (no error)"=w2196, "Rack S7 300/400"=w2202, "timeout [ms]"=1000 ("timeout [ms] 2"), "IP address"=w2192) -> ("error out"=w2199:errorcluster, "S7 Connection out"=w2200:T5)  [unwired: 3 in]
          }
          frame "Int" {
            w2210 = PLC_Comm_State."Write"  # Enum
            w2214 = TRUE  # Use Rack/Slot for S71200/1500
            w2215 = u8 1  # Slot S7 300/400
            w2216 = u8 0  # Rack S7 300/400
            w2217 = u16[] [43]  # Data Block #
            # "Initialize and set first bits"
            n708 = call "Stall Data Flow.vim"("value in"=w2208, "milliseconds to wait"=u32 516) -> ("value out"=w2207:errorcluster)  [unwired: 1 out]
            n709 = call <vilib>:"connect.vi"("Use Rack/Slot for S71200/1500"=w2214, "Slot S7 300/400"=w2215, "PLC Type"=PLC_Type."S7 1200" ("PLC Type 2"), "error in (no error)"=w2207, "Rack S7 300/400"=w2216, "timeout [ms]"=1000 ("timeout [ms] 2"), "IP address"=w2209) -> ("error out"=w2219:errorcluster, "S7 Connection out"=w2218:T5)  [unwired: 3 in]
            n710 = for {
              tunnel: w2217 -> [w2227] mode=indexing
              shift-right: [w2225] -> w2212
              shift-left: w2218 -> [w2223]
              tunnel: w2219 -> [w2224]
              tunnel: [w2222] -> w2213
              w2226 = i32[] [0, 0]  # DINT input array
              # "Reset Search and save \nbit on software start"
              n711 = call-poly <vilib>:"write DB.vi"("DINT input array"=w2226, "error in (no error)"=w2224, "Data Block #"=w2227, "S7 Connection in"=w2223) -> ("error out"=w2222:errorcluster, "S7 Connection out"=w2225:T5)  [unwired: 4 in, 2 out]
            }
          }
          frame "Write" {
            w2233 = u16 44 ("Data Block #")
            w2248 = PLC_Comm_State."Read"  # Enum
            n712 = global read "DATA LOG.vi" "OP 60 Outputs"() -> (w2247:bool)
            n713 = case shown="True" w2247 {
              tunnel: w2230 -> [w2260 w2273]
              tunnel: [w2261 w2263] -> w2241
              tunnel: [w2260 w2266] -> w2240
              tunnel: w2229 -> [w2261 w2270]
              frame False {
              }
              frame True {
                w2274 = u16 44  # Data Block #
                n714 = call "PADMINI_AUTO_BARCODE_STATUS 60.vi"("Enum"=enum16{"Read", "Write"}."Read", "error in (no error)"=w2270) -> ("error out"=w2269:errorcluster, "O/P"=w2271:i32[])  [unwired: 8 in]
                n715 = call-poly <vilib>:"write DB.vi"("DINT input array"=w2271, "error in (no error)"=w2269, "Data Block #"=w2274, "S7 Connection in"=w2273) -> ("error out"=w2264:errorcluster, "S7 Connection out"=w2265:T5)  [unwired: 4 in, 2 out]
                n716 = call-poly <vilib>:"write DB.vi"("DINT input array"=i32[] [0] ("Data Byte"), "error in (no error)"=w2264, "Data Block #"=u16 43, "S7 Connection in"=w2265) -> ("error out"=w2263:errorcluster, "S7 Connection out"=w2266:T5)  [unwired: 4 in, 2 out]
                n717 = Unbundle By Name(w2263) -> ("status"=w2262:bool)
                n718 = global write "DATA LOG.vi" "OP 60 Outputs"(w2262) -> ()
              }
            }
            n719 = global read "DATA LOG.vi" "OP 60 reset"() -> (w2239:bool)
            n720 = global read "DATA LOG.vi" "Auto Cycle On"() -> (w2238:bool)
            n721 = case shown="True" w2239 {
              tunnel: w2241 -> [w2250 w2259]
              tunnel: [w2250 w2253] -> w2242
              tunnel: w2240 -> [w2251 w2258]
              tunnel: [w2251 w2257] -> w2243
              frame False {
              }
              frame True {
                n722 = call-poly <vilib>:"write DB.vi"("Item offset [byte]"=u16 4 ("Data Block #"), "DINT input array"=i32[] [0], "error in (no error)"=w2259, "Data Block #"=u16 43, "S7 Connection in"=w2258) -> ("error out"=w2253:errorcluster, "S7 Connection out"=w2257:T5)  [unwired: 3 in, 2 out]
                n723 = Unbundle By Name(w2253) -> ("status"=w2252:bool)
                n724 = global write "DATA LOG.vi" "OP 60 reset"(w2252) -> ()
              }
            }
            n725 = Boolean To (0,1)(Boolean=w2238) -> (0, 1=w2237:i16)
            n726 = Build Array(w2237) -> (w2236:i16[])
            n727 = global read "Global 1.vi" "Filtered BARCODE selected"() -> (w2246:string[])
            n728 = call-poly <vilib>:"write DB.vi"("Item offset [byte]"=u32 20, "DINT input array"=w2236, "error in (no error)"=w2242, "Data Block #"=w2233, "S7 Connection in"=w2243) -> ("error out"=w2245:errorcluster, "S7 Connection out"=w2244:T5)  [unwired: 3 in, 2 out]
            n729 = call-poly <vilib>:"write DB.vi"("Item offset [byte]"=u32 24, "Input STRINGS"=w2246, "error in (no error)"=w2245, "String length reserved in DB (default=254)"=u16 15, "Data Block #"=w2233, "S7 Connection in"=w2244) -> ("error out"=w2228:errorcluster, "S7 Connection out"=w2231:T5)  [unwired: 2 in, 2 out]
          }
          frame "Read" {
            w2284 = u16 43 ("Data Block #")
            w2302 = PLC_Comm_State."Write"  # Enum
            n730 = call-poly <vilib>:"read DB.vi"("Item offset [byte]"=u32 8, "error in (no error)"=w2277, "items #"=u16 6 ("Items # [byte]"), "Data Block #"=w2284, "S7 Connection in"=w2276) -> ("error out"=w2298:errorcluster, "REAL result array"=w2301:sgl[], "S7 Connection out"=w2299:T5)  [unwired: 4 in]
            n731 = call-poly <vilib>:"read DB.vi"("Item offset [byte]"=u32 32, "String length reserved in DB (default=254)"=u16 50, "error in (no error)"=w2298, "items #"=u16 1 ("Items # [byte]"), "Data Block #"=w2284, "S7 Connection in"=w2299) -> ("error out"=w2295:errorcluster, "STRING result Array"=w2293:string[], "S7 Connection out"=w2294:T5)  [unwired: 2 in, 1 out]
            n732 = call-poly <vilib>:"read DB.vi"("Item offset [byte]"=u32 84, "String length reserved in DB (default=254)"=u16 10, "error in (no error)"=w2295, "items #"=u16 7 ("Items # [byte]"), "Data Block #"=w2284, "S7 Connection in"=w2294) -> ("error out"=w2296:errorcluster, "STRING result Array"=w2297:string[], "S7 Connection out"=w2290:T5)  [unwired: 2 in, 1 out]
            n733 = Build Array (concatenate)(w2293, w2297) -> (w2300:string[])
            n734 = call-poly <vilib>:"read DB.vi"("error in (no error)"=w2296, "items #"=u16 2 ("Items # [byte]"), "Data Block #"=u16 43, "S7 Connection in"=w2290) -> ("error out"=w2292:errorcluster, "DINT result array"=w2291:i32[], "S7 Connection out"=w2275:T5)  [unwired: 5 in]
            n735 = case shown="No Error" w2292 {
              selector: w2292 -> [w2305 w2312]
              tunnel: w2291 -> [w2304 _]
              tunnel: w2300 -> [w2311 _]
              tunnel: w2301 -> [w2309 _]
              tunnel: [w2306 w2312] -> w2278
              frame No Error {
                w2310 = enum16{"Read", "Write"}."Write" ("Enum")
                n736 = call "PADMINI_AUTO_BARCODE_STRING 60.vi"("Enum"=w2310, "error in (no error)"=w2305, "Input"=w2311) -> ("error out"=w2308:errorcluster)  [unwired: 7 in, 1 out]
                n737 = call "PADMINI_AUTO_CYCLE VALUE 60.vi"("Enum"=w2310, "error in (no error)"=w2308, "Input"=w2309) -> ("error out"=w2307:errorcluster)  [unwired: 7 in, 1 out]
                n738 = call "PADMINI_AUTO_CYCLE STATE 60.vi"("Enum"=w2310, "error in (no error)"=w2307, "Input"=w2304) -> ("error out"=w2306:errorcluster)  [unwired: 7 in, 1 out]
              }
              frame Error {
              }
            }
          }
          frame "Error" {
            w2314 = PLC_Comm_State."Write"  # Enum
            n739 = global write "Global 1.vi" "PLC5 error"(w2313) -> ()
            n740 = call <vilib>:"Clear Errors.vi"("error in (no error)"=w2313) -> ("error out"=w2316:errorcluster)  [unwired: 5 in, 1 out]
          }
          frame "Disconnect" {
            w2318 = PLC_Comm_State."Disconnect"  # Enum
            w2321 = T5 {"TCP Connection Ref"=refnum, "IP address"="", "timeout ms"=5000, "Connected?"=FALSE, "PLC Type"=enum."S7 1200", "Rack S7 400"=0, "Slot S7 400"=0, "PDU Size"=0, "connection semaphore"=refnum}  # S7 Connection out
            n741 = call <vilib>:"Clear Errors.vi"("error in (no error)"=w2322) -> ("error out"=w2325:errorcluster)  [unwired: 5 in, 1 out]
            n742 = call <vilib>:"disconnect.vi"("error in (no error)"=w2325, "S7 Connection in"=w2323) -> ("error out"=w2324:errorcluster)  [unwired: 8 in, 1 out]
          }
          frame "Write2" {
            # "No Use"
          }
          frame "Write3" {
            # "No Use"
          }
          frame "Read2" {
            # "No Use"
          }
          frame "Read3" {
            # "No Use"
          }
        }
        n743 = Tick Count (ms)() -> (millisecond timer value=w2154:u32)
        n744 = feedback #6() -> (w2153:u32)  [unwired: 1 in]
        n745 = feedback-in #6(w2154) -> ()
        n746 = Subtract(x=w2154, y=w2153) -> (x-y=w2152:u32)
        n747 = global write "Global 1.vi" "Loop Time PLC 5"(w2152) -> ()
        n748 = Wait (ms)(milliseconds to wait=w2171) -> ()  [unwired: 1 out]
        n749 = call "PADMINI_STOP_ALL.vi"("Enum"=enum16{"Read", "Write"}."Read") -> ("Boolean 2"=w2162:bool)  [unwired: 9 in, 1 out]
        n750 = local read "stop"() -> (w2157:bool)
        n751 = case shown="Error" w2175 {
          selector: w2175 -> [w2178 w2181]
          tunnel: [w2178 w2185] -> w2158
          tunnel: [w2177 w2180] -> w2165
          tunnel: w2170 -> [w2177 _]
          tunnel: [w2176 w2191] -> w2169
          tunnel: w2168 -> [w2176 w2191]
          tunnel: w2164 -> [_ w2189]
          frame No Error {
          }
          frame Error {
            w2182 = PLC_Comm_State."Connect"  # Enum
            w2179 = PLC_Comm_State."Error"  # Enum
            n752 = Unbundle By Name(w2181) -> ("source"=w2190:string)
            n753 = call <userlib>:"Get Strings from Enum__ogtk.vi"("Enum"=w2189) -> ("String Value"=w2188:string)  [unwired: 7 in, 3 out]
            n754 = Concatenate Strings(w2188, "    " ("string"), w2190) -> (w2186:string)
            n755 = Bundle By Name(cluster=w2181, "source"=w2186) -> (w2185:errorcluster)
            n756 = call <vilib>:"Clear Errors.vi"("error in (no error)"=w2181, "specific error code to clear (0: all)"=6002) -> ("specific error cleared?"=w2184:bool)  [unwired: 4 in, 1 out]
            n757 = Select(t=w2182, s=w2184, f=w2179) -> (s? t:f=w2180:T1)
          }
        }
        n758 = Or(x=w2157, y=w2162) -> (x .or. y?=w2160:bool)
        n759 = Select(t=w2163, s=w2160, f=w2165) -> (s? t:f=w2166:T1)
        n760 = Unbundle By Name(w2158) -> ("status"=w2159:bool)
        n761 = Not(x=w2159) -> (.not. x?=w2156:bool)
        n762 = global write "Global 1.vi" "PLC 5"(w2156) -> ()
      }
    }
  }
  n763 = disable-structure shown="Enabled" {
    disable-tunnel: [w2347 _] -> w117
    disable-tunnel: [w2344 _] -> w106
    disable-tunnel: w82 -> [w2343 w2409]
    disable-tunnel: w9 -> [w2337 w2408]
    frame Disabled {
      n764 = call <vilib>:"connect.vi"("Use Rack/Slot for S71200/1500"=TRUE, "Slot S7 300/400"=u8 1, "PLC Type"=PLC_Type."S7 1200" ("PLC Type 2"), "error in (no error)"=w2337, "Rack S7 300/400"=u8 0, "timeout [ms]"=1000, "IP address"=w2343) -> ("error out"=w2339:errorcluster, "S7 Connection out"=w2338:T5)  [unwired: 3 in]
      n765 = for {
        tunnel: u16[] [83, 94] ("Data Block #") -> [w2353] mode=indexing
        shift-right: [w2351] -> w2341
        shift-left: w2338 -> [w2348]
        tunnel: w2339 -> [w2349]
        tunnel: [w2350] -> w2340
        w2352 = i32[] [0, 0]  # DINT input array
        # "Reset Search and save \nbit on software start"
        n766 = call-poly <vilib>:"write DB.vi"("DINT input array"=w2352, "error in (no error)"=w2349, "Data Block #"=w2353, "S7 Connection in"=w2348) -> ("error out"=w2350:errorcluster, "S7 Connection out"=w2351:T5)  [unwired: 4 in, 2 out]
      }
      n767 = while {
        shift-right: [w2356] -> w2344
        shift-left: w2341 -> [w2366]
        shift-right: [w2364] -> w2347
        shift-left: w2340 -> [w2365]
        tunnel: w2343 -> [w2354]
        stop <- w2359 stop-if-true
        # "OP 10 AND 20"
        n768 = flat-sequence {
          tunnel: [w2369] -> w2358
          tunnel: [w2375] -> w2357
          tunnel: w2365 -> [w2376]
          tunnel: w2366 -> [w2377]
          tunnel: [w2374] -> w2355
          tunnel: w2354 -> [w2374]
          tunnel: [w2381] -> w2364
          tunnel: [w2380] -> w2356
          tunnel: w2358 -> [w2382]
          tunnel: w2357 -> [w2378]
          tunnel: w2355 -> [w2379]
          frame #0 {
            # "NEW CHANGES"
            n769 = call "PLC_OP10_Write.vi"("error in (no error)"=w2376, "S7 Connection in"=w2377) -> ("error out"=w2372:errorcluster, "S7 Connection out"=w2373:T5)  [unwired: 8 in]
            n770 = call "PLC_OP10_Read.vi"("error in (no error)"=w2372, "S7 Connection in"=w2373) -> ("error out"=w2371:errorcluster, "S7 Connection out"=w2370:T5)  [unwired: 8 in]
            n771 = call "PLC_OP20_Write.vi"("error in (no error)"=w2371, "S7 Connection in"=w2370) -> ("error out"=w2367:errorcluster, "S7 Connection out"=w2368:T5)  [unwired: 8 in]
            n772 = call "PLC_OP20_Read.vi"("error in (no error)"=w2367, "S7 Connection in"=w2368) -> ("error out"=w2375:errorcluster, "S7 Connection out 2"=w2369:T5)  [unwired: 8 in]
          }
          frame #1 {
            # "RECONNECT"
            n773 = case shown="Error" w2378 {
              selector: w2378 -> [w2386 w2388]
              tunnel: [w2385 w2391] -> w2380
              tunnel: [w2386 w2392] -> w2381
              tunnel: w2382 -> [w2385 w2390]
              tunnel: w2379 -> [_ w2389]
              frame No Error {
              }
              frame Error {
                n774 = Unbundle By Name(w2388) -> ("code"=w2387:i32)
                n775 = case shown="1, 66" w2387 {
                  tunnel: w2388 -> [w2393 w2406]
                  tunnel: [w2394 w2404] -> w2392
                  tunnel: [w2395 w2403] -> w2391
                  tunnel: w2390 -> [w2395 w2400]
                  tunnel: w2389 -> [_ w2399]
                  frame 0, Default {
                    n776 = call <vilib>:"Clear Errors.vi"("error in (no error)"=w2393) -> ("error out"=w2394:errorcluster)  [unwired: 5 in, 1 out]
                    n777 = global write "Global 1.vi" "PLC1 error"(w2393) -> ()
                  }
                  frame 1, 66 {
                    w2398 = 1000  # timeout [ms]
                    n778 = call <vilib>:"Clear Errors.vi"("error in (no error)"=w2406) -> ("error out"=w2407:errorcluster)  [unwired: 5 in, 1 out]
                    n779 = call <vilib>:"disconnect.vi"("error in (no error)"=w2407, "S7 Connection in"=w2400) -> ("error out"=w2405:errorcluster)  [unwired: 8 in, 1 out]
                    n780 = call <vilib>:"Clear Errors.vi"("error in (no error)"=w2405) -> ("error out"=w2402:errorcluster)  [unwired: 5 in, 1 out]
                    n781 = call <vilib>:"connect.vi"("Use Rack/Slot for S71200/1500"=TRUE, "Slot S7 300/400"=u8 1, "PLC Type"=PLC_Type."S7 1200" ("PLC Type 2"), "error in (no error)"=w2402, "timeout [ms]"=w2398, "IP address"=w2399) -> ("error out"=w2404:errorcluster, "S7 Connection out"=w2403:T5)  [unwired: 4 in]
                  }
                }
              }
            }
            n782 = Unbundle By Name(w2378) -> ("status"=w2384:bool)
            n783 = Not(x=w2384) -> (.not. x?=w2383:bool)
            "PLC 1" <- w2383
            n784 = global write "Global 1.vi" "PLC 1"(w2383) -> ()
          }
        }
        n785 = call "PADMINI_STOP_ALL.vi"("Enum"=enum16{"Read", "Write"}."Read") -> ("Boolean 2"=w2361:bool)  [unwired: 9 in, 1 out]
        n786 = Wait (ms)(milliseconds to wait=u32 1200) -> ()  [unwired: 1 out]
        n787 = Or(x="stop", y=w2361) -> (x .or. y?=w2359:bool)
      }
    }
    frame Enabled {
      w2410 = PLC_Comm_State."Int"  # Enum
      n788 = while {
        shift-right: [w2425] -> _
        shift-left: w2410 -> [w2433]
        shift-right: [w2417] -> _
        shift-left: w2408 -> [w2432]
        shift-right: [w2428] -> _
        shift-left: _ -> [w2431]
        tunnel: w2409 -> [w2414]
        stop <- w2426 stop-if-true
        w2422 = PLC_Comm_State."Disconnect"  # Enum
        w2430 = u32 800  # milliseconds to wait
        # "Int-->Write-->Read---if--Error-->reconnect\n               ^------v                                       v\n                ^------------------------------v"
        # "OP 10-20"
        n789 = case shown="\"Error\"" w2433 {
          selector: w2433 -> [w2453 w2468 w2490 w2495 w2502 w2507 w2511 w2515 _ _]
          tunnel: [w2458 w2471 w2487 w2491 w2499 w2505 w2512 w2520 w2523 w2525] -> w2434
          tunnel: [w2459 w2470 w2485 w2493 w2497 w2503 w2513 w2517 w2522 w2524] -> w2427
          tunnel: w2432 -> [w2456 w2469 w2488 w2492 w2500 w2506 w2509 w2518 w2523 w2525]
          tunnel: w2431 -> [w2454 _ w2486 w2494 w2498 w2504 w2513 w2519 w2522 w2524]
          tunnel: [w2452 w2467 w2489 w2496 w2501 w2508 w2510 w2514 _ _] -> w2429
          tunnel: [_ _ _ _ _ _ _ TRUE _ _] -> w2426
          tunnel: [w2453 w2468 w2490 w2495 w2502 w2507 w2511 w2515 _ _] -> w2423
          tunnel: w2414 -> [w2451 w2466 _ _ _ _ _ _ _ _]
          frame "Connect" {
            w2452 = PLC_Comm_State."Write"  # Enum
            w2464 = TRUE  # Use Rack/Slot for S71200/1500
            w2463 = u8 1  # Slot S7 300/400
            w2461 = u8 0  # Rack S7 300/400
            # "Reconect"
            n790 = call <vilib>:"disconnect.vi"("error in (no error)"=w2456, "S7 Connection in"=w2454) -> ("error out"=w2457:errorcluster)  [unwired: 8 in, 1 out]
            n791 = call <vilib>:"Clear Errors.vi"("error in (no error)"=w2457) -> ("error out"=w2455:errorcluster)  [unwired: 5 in, 1 out]
            n792 = call <vilib>:"connect.vi"("Use Rack/Slot for S71200/1500"=w2464, "Slot S7 300/400"=w2463, "PLC Type"=PLC_Type."S7 1200" ("PLC Type 2"), "error in (no error)"=w2455, "Rack S7 300/400"=w2461, "timeout [ms]"=1000 ("timeout [ms] 2"), "IP address"=w2451) -> ("error out"=w2458:errorcluster, "S7 Connection out"=w2459:T5)  [unwired: 3 in]
          }
          frame "Int" {
            w2467 = PLC_Comm_State."Write"  # Enum
            w2472 = TRUE  # Use Rack/Slot for S71200/1500
            w2473 = u8 1  # Slot S7 300/400
            w2474 = u8 0  # Rack S7 300/400
            # "Initialize and set first bits"
            n793 = call <vilib>:"connect.vi"("Use Rack/Slot for S71200/1500"=w2472, "Slot S7 300/400"=w2473, "PLC Type"=PLC_Type."S7 1200" ("PLC Type 2"), "error in (no error)"=w2469, "Rack S7 300/400"=w2474, "timeout [ms]"=1000 ("timeout [ms] 2"), "IP address"=w2466) -> ("error out"=w2476:errorcluster, "S7 Connection out"=w2475:T5)  [unwired: 3 in]
            n794 = for {
              tunnel: u16[] [83, 94] ("Data Block #") -> [w2484] mode=indexing
              shift-right: [w2482] -> w2470
              shift-left: w2475 -> [w2480]
              tunnel: w2476 -> [w2481]
              tunnel: [w2479] -> w2471
              w2483 = i32[] [0, 0]  # DINT input array
              # "Reset Search and save \nbit on software start"
              n795 = call-poly <vilib>:"write DB.vi"("DINT input array"=w2483, "error in (no error)"=w2481, "Data Block #"=w2484, "S7 Connection in"=w2480) -> ("error out"=w2479:errorcluster, "S7 Connection out"=w2482:T5)  [unwired: 4 in, 2 out]
            }
          }
          frame "Write" {
            w2489 = PLC_Comm_State."Write2"  # Enum
            # "OP 10 Write"
            n796 = call "PLC_OP10_Write.vi"("S7 Connection in"=w2486, "error in (no error)"=w2488) -> ("S7 Connection out"=w2485:T5, "error out"=w2487:errorcluster)  [unwired: 12 in]
          }
          frame "Write2" {
            w2496 = PLC_Comm_State."Read"  # Enum
            # "op 20 wirte 2"
            n797 = call "PLC_OP20_Write.vi"("S7 Connection in"=w2494, "error in (no error)"=w2492) -> ("S7 Connection out"=w2493:T5, "error out"=w2491:errorcluster)  [unwired: 7 in]
          }
          frame "Read" {
            w2501 = PLC_Comm_State."Read2"  # Enum
            # "OP10 read"
            n798 = call "PLC_OP10_Read.vi"("error in (no error)"=w2500, "S7 Connection in"=w2498) -> ("error out"=w2499:errorcluster, "S7 Connection out"=w2497:T5)  [unwired: 8 in]
          }
          frame "Read2" {
            w2508 = PLC_Comm_State."Write"  # Enum
            # "Op20 Read2"
            n799 = call "PLC_OP20_Read.vi"("error in (no error)"=w2506, "S7 Connection in"=w2504) -> ("error out"=w2505:errorcluster, "S7 Connection out 2"=w2503:T5)  [unwired: 8 in]
          }
          frame "Error" {
            w2510 = PLC_Comm_State."Write"  # Enum
            n800 = global write "Global 1.vi" "PLC1 error"(w2509) -> ()
            n801 = call <vilib>:"Clear Errors.vi"("error in (no error)"=w2509) -> ("error out"=w2512:errorcluster)  [unwired: 5 in, 1 out]
          }
          frame "Disconnect" {
            w2514 = PLC_Comm_State."Disconnect"  # Enum
            w2517 = T5 {"TCP Connection Ref"=refnum, "IP address"="", "timeout ms"=5000, "Connected?"=FALSE, "PLC Type"=enum."S7 1200", "Rack S7 400"=0, "Slot S7 400"=0, "PDU Size"=0, "connection semaphore"=refnum}  # S7 Connection out
            n802 = call <vilib>:"Clear Errors.vi"("error in (no error)"=w2518) -> ("error out"=w2521:errorcluster)  [unwired: 5 in, 1 out]
            n803 = call <vilib>:"disconnect.vi"("error in (no error)"=w2521, "S7 Connection in"=w2519) -> ("error out"=w2520:errorcluster)  [unwired: 8 in, 1 out]
          }
          frame "Write3" {
            # "No Use"
          }
          frame "Read3" {
            # "No Use"
          }
        }
        n804 = Tick Count (ms)() -> (millisecond timer value=w2413:u32)
        n805 = feedback #7() -> (w2412:u32)  [unwired: 1 in]
        n806 = feedback-in #7(w2413) -> ()
        n807 = Subtract(x=w2413, y=w2412) -> (x-y=w2411:u32)
        n808 = global write "Global 1.vi" "Loop Time PLC 1"(w2411) -> ()
        n809 = Wait (ms)(milliseconds to wait=w2430) -> ()  [unwired: 1 out]
        n810 = call "PADMINI_STOP_ALL.vi"("Enum"=enum16{"Read", "Write"}."Read") -> ("Boolean 2"=w2421:bool)  [unwired: 9 in, 1 out]
        n811 = local read "stop"() -> (w2416:bool)
        n812 = case shown="Error" w2434 {
          selector: w2434 -> [w2437 w2442]
          tunnel: [w2437 w2444] -> w2417
          tunnel: [w2436 w2438] -> w2424
          tunnel: w2429 -> [w2436 _]
          tunnel: [w2435 w2450] -> w2428
          tunnel: w2427 -> [w2435 w2450]
          tunnel: w2423 -> [_ w2448]
          frame No Error {
          }
          frame Error {
            w2440 = PLC_Comm_State."Connect"  # Enum
            w2439 = PLC_Comm_State."Error"  # Enum
            n813 = Unbundle By Name(w2442) -> ("source"=w2449:string)
            n814 = call <userlib>:"Get Strings from Enum__ogtk.vi"("Enum"=w2448) -> ("String Value"=w2447:string)  [unwired: 7 in, 3 out]
            n815 = call <vilib>:"Clear Errors.vi"("error in (no error)"=w2442, "specific error code to clear (0: all)"=6002) -> ("specific error cleared?"=w2441:bool)  [unwired: 4 in, 1 out]
            n816 = Concatenate Strings(w2447, "    " ("string"), w2449) -> (w2445:string)
            n817 = Bundle By Name(cluster=w2442, "source"=w2445) -> (w2444:errorcluster)
            n818 = Select(t=w2440, s=w2441, f=w2439) -> (s? t:f=w2438:T1)
          }
        }
        n819 = Or(x=w2416, y=w2421) -> (x .or. y?=w2419:bool)
        n820 = Select(t=w2422, s=w2419, f=w2424) -> (s? t:f=w2425:T1)
        n821 = Unbundle By Name(w2417) -> ("status"=w2418:bool)
        n822 = Not(x=w2418) -> (.not. x?=w2415:bool)
        n823 = global write "Global 1.vi" "PLC 1"(w2415) -> ()
      }
    }
  }
  n824 = while {
    shift-right: [w2539] -> _
    shift-left: w1 -> [w2548]
    shift-right: [w2529] -> w84
    shift-left: w9 -> [w2547]
    shift-right: [w2542] -> _
    shift-left: _ -> [w2546]
    tunnel: w83 -> [w2545]
    stop <- w2540 stop-if-true
    w2536 = PLC_Comm_State."Disconnect"  # Enum
    w2544 = u32 800  # milliseconds to wait
    # "Int-->Write-->Read---if--Error-->reconnect\n               ^------v                                       v\n                ^------------------------------v"
    # "OP 30"
    n825 = case shown="\"Error\"" w2548 {
      selector: w2548 -> [w2567 w2583 w2607 w2613 w2616 w2620 _ _ _ _]
      tunnel: [w2572 w2587 w2602 w2609 w2617 w2625 w2627 w2630 w2632 w2634] -> w2549
      tunnel: [w2573 w2586 w2604 w2610 w2618 w2622 w2628 w2629 w2631 w2633] -> w2541
      tunnel: w2547 -> [w2570 w2585 w2603 w2608 w2614 w2623 w2627 w2630 w2632 w2634]
      tunnel: w2546 -> [w2568 _ w2605 w2611 w2618 w2624 w2628 w2629 w2631 w2633]
      tunnel: w2545 -> [w2574 w2584 _ _ _ _ _ _ _ _]
      tunnel: [w2566 w2582 w2606 w2612 w2615 w2619 _ _ _ _] -> w2543
      tunnel: [_ _ _ _ _ TRUE _ _ _ _] -> w2540
      tunnel: [w2567 w2583 w2607 w2613 w2616 w2620 _ _ _ _] -> w2537
      frame "Connect" {
        w2566 = PLC_Comm_State."Write"  # Enum
        w2579 = TRUE  # Use Rack/Slot for S71200/1500
        w2578 = u8 1  # Slot S7 300/400
        w2576 = u8 0  # Rack S7 300/400
        # "Reconect"
        n826 = call <vilib>:"disconnect.vi"("error in (no error)"=w2570, "S7 Connection in"=w2568) -> ("error out"=w2571:errorcluster)  [unwired: 8 in, 1 out]
        n827 = call <vilib>:"Clear Errors.vi"("error in (no error)"=w2571) -> ("error out"=w2569:errorcluster)  [unwired: 5 in, 1 out]
        n828 = call <vilib>:"connect.vi"("Use Rack/Slot for S71200/1500"=w2579, "Slot S7 300/400"=w2578, "PLC Type"=PLC_Type."S7 1200" ("PLC Type 2"), "error in (no error)"=w2569, "Rack S7 300/400"=w2576, "timeout [ms]"=1000 ("timeout [ms] 2"), "IP address"=w2574) -> ("error out"=w2572:errorcluster, "S7 Connection out"=w2573:T5)  [unwired: 3 in]
      }
      frame "Int" {
        w2582 = PLC_Comm_State."Write"  # Enum
        w2588 = TRUE  # Use Rack/Slot for S71200/1500
        w2589 = u8 1  # Slot S7 300/400
        w2590 = u8 0  # Rack S7 300/400
        w2591 = u16[] [37]  # Data Block #
        n829 = call "Stall Data Flow.vim"("value in"=w2585, "milliseconds to wait"=u32 129) -> ("value out"=w2581:errorcluster)  [unwired: 1 out]
        n830 = call <vilib>:"connect.vi"("Use Rack/Slot for S71200/1500"=w2588, "Slot S7 300/400"=w2589, "PLC Type"=PLC_Type."S7 1200" ("PLC Type 2"), "error in (no error)"=w2581, "Rack S7 300/400"=w2590, "timeout [ms]"=1000 ("timeout [ms] 2"), "IP address"=w2584) -> ("error out"=w2593:errorcluster, "S7 Connection out"=w2592:T5)  [unwired: 3 in]
        n831 = for {
          tunnel: w2591 -> [w2601] mode=indexing
          shift-right: [w2599] -> w2586
          shift-left: w2592 -> [w2597]
          tunnel: w2593 -> [w2598]
          tunnel: [w2596] -> w2587
          w2600 = i32[] [0, 0]  # DINT input array
          # "Reset Search and save \nbit on software start"
          n832 = call-poly <vilib>:"write DB.vi"("DINT input array"=w2600, "error in (no error)"=w2598, "Data Block #"=w2601, "S7 Connection in"=w2597) -> ("error out"=w2596:errorcluster, "S7 Connection out"=w2599:T5)  [unwired: 4 in, 2 out]
        }
      }
      frame "Write" {
        w2606 = PLC_Comm_State."Read"  # Enum
        n833 = call "PLC_OP30_Write.vi"("error in (no error)"=w2603, "S7 Connection in"=w2605) -> ("error out"=w2602:errorcluster, "S7 Connection out"=w2604:T5)  [unwired: 8 in]
      }
      frame "Read" {
        w2612 = PLC_Comm_State."Write"  # Enum
        # "OP100 OK\nOP 100 NG"
        n834 = call "PLC_OP30_Read.vi"("error in (no error)"=w2608, "S7 Connection in"=w2611) -> ("error out"=w2609:errorcluster, "S7 Connection out 2"=w2610:T5)  [unwired: 8 in]
      }
      frame "Error" {
        w2615 = PLC_Comm_State."Write"  # Enum
        n835 = global write "Global 1.vi" "PLC2 error"(w2614) -> ()
        n836 = call <vilib>:"Clear Errors.vi"("error in (no error)"=w2614) -> ("error out"=w2617:errorcluster)  [unwired: 5 in, 1 out]
      }
      frame "Disconnect" {
        w2619 = PLC_Comm_State."Disconnect"  # Enum
        w2622 = T5 {"TCP Connection Ref"=refnum, "IP address"="", "timeout ms"=5000, "Connected?"=FALSE, "PLC Type"=enum."S7 1200", "Rack S7 400"=0, "Slot S7 400"=0, "PDU Size"=0, "connection semaphore"=refnum}  # S7 Connection out
        n837 = call <vilib>:"Clear Errors.vi"("error in (no error)"=w2623) -> ("error out"=w2626:errorcluster)  [unwired: 5 in, 1 out]
        n838 = call <vilib>:"disconnect.vi"("error in (no error)"=w2626, "S7 Connection in"=w2624) -> ("error out"=w2625:errorcluster)  [unwired: 8 in, 1 out]
      }
      frame "Write2" {
        # "SPARE"
      }
      frame "Write3" {
        # "No Use"
      }
      frame "Read2" {
        # "No Use"
      }
      frame "Read3" {
        # "No Use"
      }
    }
    n839 = Tick Count (ms)() -> (millisecond timer value=w2528:u32)
    n840 = feedback #8() -> (w2527:u32)  [unwired: 1 in]
    n841 = feedback-in #8(w2528) -> ()
    n842 = Subtract(x=w2528, y=w2527) -> (x-y=w2526:u32)
    n843 = global write "Global 1.vi" "Loop Time PLC 2"(w2526) -> ()
    n844 = Wait (ms)(milliseconds to wait=w2544) -> ()  [unwired: 1 out]
    n845 = call "PADMINI_STOP_ALL.vi"("Enum"=enum16{"Read", "Write"}."Read") -> ("Boolean 2"=w2535:bool)  [unwired: 9 in, 1 out]
    n846 = local read "stop"() -> (w2534:bool)
    n847 = case shown="Error" w2549 {
      selector: w2549 -> [w2552 w2555]
      tunnel: [w2552 w2559] -> w2529
      tunnel: [w2551 w2554] -> w2538
      tunnel: w2543 -> [w2551 _]
      tunnel: [w2550 w2565] -> w2542
      tunnel: w2541 -> [w2550 w2565]
      tunnel: w2537 -> [_ w2563]
      frame No Error {
      }
      frame Error {
        w2556 = PLC_Comm_State."Connect"  # Enum
        w2553 = PLC_Comm_State."Error"  # Enum
        n848 = Unbundle By Name(w2555) -> ("source"=w2564:string)
        n849 = call <userlib>:"Get Strings from Enum__ogtk.vi"("Enum"=w2563) -> ("String Value"=w2562:string)  [unwired: 7 in, 3 out]
        n850 = Concatenate Strings(w2562, "    " ("string"), w2564) -> (w2560:string)
        n851 = Bundle By Name(cluster=w2555, "source"=w2560) -> (w2559:errorcluster)
        n852 = call <vilib>:"Clear Errors.vi"("error in (no error)"=w2555, "specific error code to clear (0: all)"=6002) -> ("specific error cleared?"=w2558:bool)  [unwired: 4 in, 1 out]
        n853 = Select(t=w2556, s=w2558, f=w2553) -> (s? t:f=w2554:T1)
      }
    }
    n854 = Or(x=w2534, y=w2535) -> (x .or. y?=w2532:bool)
    n855 = Select(t=w2536, s=w2532, f=w2538) -> (s? t:f=w2539:T1)
    n856 = Unbundle By Name(w2529) -> ("status"=w2531:bool)
    n857 = Not(x=w2531) -> (.not. x?=w2530:bool)
    n858 = global write "Global 1.vi" "PLC 2"(w2530) -> ()
  }
  n859 = Merge Errors(w84, w3, w4, w6) -> (w80:errorcluster)
  n860 = call <vilib>:"Clear Errors.vi"("error in (no error)"=w117) -> ("error out"=w107:errorcluster)  [unwired: 5 in, 1 out]
  n861 = call <vilib>:"disconnect.vi"("error in (no error)"=w107, "S7 Connection in"=w106) -> ("error out"=w105:errorcluster)  [unwired: 8 in, 1 out]
  n862 = Merge Errors(w5, w2, w7) -> (w28:errorcluster)
  n863 = Merge Errors(w105, w80, w28) -> (w122:errorcluster)
  n864 = call <vilib>:"Simple Error Handler.vi"("type of dialog (OK msg:1)"=w10, "error in (no error)"=w122) -> ("error out"=w121:errorcluster)  [unwired: 3 in, 4 out]
  n865 = control-ref of="This VI"() -> (w11:refnum<vi>)
  n866 = call <vilib>:"Clear Errors.vi"("error in (no error)"=w121) -> ("error out"=w120:errorcluster)  [unwired: 5 in, 1 out]
  n867 = invoke class="VI" method="FP.Close"(reference=w11, error in=w120) -> (error out=→"error out":errorcluster)  [unwired: 1 in, 2 out]
